vi "Controle_Manip_Main_GUI.vi"() -> ()   [LabVIEW 2019]
doc: "VI for micro-photoluminescence setup in GH013 to study the emission properties of single nanoemitters in the visible range."
uses:
  subVIs/TypeDefs/AcqMode.ctl
  D:/Users/manip-thz/Documents/Controle_Manip_2020/Thorlabs.MotionControl.Controls.dll
  Thorlabs.MotionControl.Controls.dll
  D:/Users/manip-thz/Documents/Controle_Manip_2020/Thorlabs.MotionControl.KCube.SolenoidCLI.dll
  Thorlabs.MotionControl.KCube.SolenoidCLI.dll
  D:/Users/manip-thz/Documents/Controle_Manip_2020/Thorlabs.MotionControl.KCube.PiezoCLI.dll
  Thorlabs.MotionControl.KCube.PiezoCLI.dll
  subVIs/Light Field/lightfield-automation-labview/LightField Automation.lvclass
  subVIs/Light Field/lightfield-automation-labview/VIs/TypeDefs/OpticalPortLocation.ctl
  C:/Program Files/Thorlabs/Scientific Imaging/DCx Camera Support/Develop/DotNet/uc480DotNet.dll
  <vilib>/DAQmx/write.llb/DAQmx Write (Analog DBL 1Chan 1Samp).vi
  <vilib>/DAQmx/create/channels.llb/DAQmx Create Channel (AO-Voltage-Basic).vi
  <vilib>/DAQmx/miscellaneous.llb/DAQmx Fill In Error Info.vi
  subVIs/Globals/Stops.vi
  subVIs/Newport/Newport ESP301/Newport ESP301.lvlib
panel:
  out "Shutter Ctrls":u16(ring)
  out "Laser on?":bool
  in  "Cryostat":enum16{"Montana", "Oxford"}(ring) caption="Cryo :"
  out "Excitation Power (uW)":dbl=0.2 caption="P    =" format="%#_3p"
  in  "Acq Time (ms)":dbl=100.0 caption="Acq Time :" min=0.0 max=360000.0 step=50.0
  in  "Auto< ?":bool
  in  "Acq Mode":T1=enum."Spectrum" caption="Mode :"
  in  "Comment":string
  out "Log file":string caption="Status"
  in  "Experiment Name":string="B1802CF_QD0"
  in  "Experiment Graph Controls":T2(tab)
  in  "CCD 1D Spectrum Main  Cursor2WL 2 Mono 2":bool caption="CCD 1D Spectrum Main  Cursor2WL"
  in  "CCD 1D Spectrum Main  Cursor2WL 1 Mono 2":bool caption="CCD 1D Spectrum Main  Cursor2WL"
  in  "CCD 1D Spectrum Main  Cursor2WL 2 Mono 1":bool caption="CCD 1D Spectrum Main  Cursor2WL"
  in  "CCD 1D Spectrum Main  Cursor2WL 1 Mono 1":bool caption="CCD 1D Spectrum Main  Cursor2WL"
  out "CCD 1D Spectrum Main Cursor 1 nm":dbl caption="nm"
  out "CCD 1D Spectrum Main Cursor 2 nm":dbl caption="nm"
  in  "Full scale":bool
  in  "Acquire Continuous Spectrum":bool
  in  "Acquire Spectrum":bool
  out "CCD 2D Image Main":dbl[][](graph)
  in  "Save Spectrum N":bool
  in  "Save Spectrum":bool
  out "CCD 1D Spectrum Main":cluster{dbl[], dbl[]}(graph)
  in  "Stop continuous":bool
  out "CCD 1D Spectrum Main Energy Scale":cluster{dbl[], dbl[]}(graph)
  out "CCD 1D Spectrum Main Cursor":dbl caption="eV" format="%#_6p"
  out "CCD 1D Spectrum Main Cursor 2":dbl caption="eV" format="%#_6p"
  out "CCD 1D Spectrum Main deltaE":dbl caption="eV" format="%#_3p"
  out "CCD 1D Spectrum Main deltanm":dbl caption="m" format="%#_3p"
  out "XY Intensity Map":dbl[][](graph)=[[3.904687043201515e-13, 6.684989195773002e-11, 3.649880430807626e-09, 6.355065252727497e-08, 3.5287820878809013e-07, 6.248749509463085e-07, 3.5287820878809013e-07, 6.355065252727497e-08, 3.649880430807626e-09, 6.684989195773002e-11, 3.904687043201515e-13], [6.684989195773002e-11, 1.1444983952148092e-08, 6.248749509463097e-07, 1.0880140221963334e-05, 6.041424029819161e-05, 0.0001069812317752422, 6.041424029819161e-05, 1.0880140221963334e-05, 6.248749509463097e-07, 1.1444983952148092e-08, 6.684989195773002e-11], [3.649880430807626e-09, 6.248749509463097e-07, 3.41170163237202e-05, 0.0005940355282204004, 0.003298505755939091, 0.005840977343195246, 0.003298505755939091, 0.0005940355282204004, 3.41170163237202e-05, 6.248749509463097e-07, 3.649880430807626e-09], [6.355065252727497e-08, 1.0880140221963334e-05, 0.0005940355282204004, 0.01034317319661825, 0.05743261926761737, 0.10170139230422684, 0.05743261926761737, 0.01034317319661825, 0.0005940355282204004, 1.0880140221963334e-05, 6.355065252727497e-08], [3.5287820878809013e-07, 6.041424029819161e-05, 0.003298505755939091, 0.05743261926761737, 0.31890655732397044, 0.5647181220077593, 0.31890655732397044, 0.05743261926761737, 0.003298505755939091, 6.041424029819161e-05, 3.5287820878809013e-07], [6.248749509463085e-07, 0.0001069812317752422, 0.005840977343195246, 0.10170139230422684, 0.5647181220077593, 1.0, 0.5647181220077593, 0.10170139230422684, 0.005840977343195246, 0.0001069812317752422, 6.248749509463085e-07], [3.5287820878809013e-07, 6.041424029819161e-05, 0.003298505755939091, 0.05743261926761737, 0.31890655732397044, 0.5647181220077593, 0.31890655732397044, 0.05743261926761737, 0.003298505755939091, 6.041424029819161e-05, 3.5287820878809013e-07], [6.355065252727497e-08, 1.0880140221963334e-05, 0.0005940355282204004, 0.01034317319661825, 0.05743261926761737, 0.10170139230422684, 0.05743261926761737, 0.01034317319661825, 0.0005940355282204004, 1.0880140221963334e-05, 6.355065252727497e-08], [3.649880430807626e-09, 6.248749509463097e-07, 3.41170163237202e-05, 0.0005940355282204004, 0.003298505755939091, 0.005840977343195246, 0.003298505755939091, 0.0005940355282204004, 3.41170163237202e-05, 6.248749509463097e-07, 3.649880430807626e-09], [6.684989195773002e-11, 1.1444983952148092e-08, 6.248749509463097e-07, 1.0880140221963334e-05, 6.041424029819161e-05, 0.0001069812317752422, 6.041424029819161e-05, 1.0880140221963334e-05, 6.248749509463097e-07, 1.1444983952148092e-08, 6.684989195773002e-11], [3.904687043201515e-13, 6.684989195773002e-11, 3.649880430807626e-09, 6.355065252727497e-08, 3.5287820878809013e-07, 6.248749509463085e-07, 3.5287820878809013e-07, 6.355065252727497e-08, 3.649880430807626e-09, 6.684989195773002e-11, 3.904687043201515e-13]]
  out "CCD 2D Image XY Map":dbl[][](graph)
  out "CCD 1D Spectrum XY Map":dbl[][](graph)
  out "Polarisation 2D Image":dbl[][](graph)
  out "Polarisation 1D Spectrum":cluster{dbl[], dbl[]}(graph) caption="64.0°"
  out "Polarisation 1D Spectrum Energy Scale":cluster{dbl[], dbl[]}(graph)
  out "Contrast":dbl
  out "Contrast Oscillations":cluster{dbl[], dbl[]}(graph)
  out "Contrast 1D Spectrum":cluster{dbl[], dbl[]}(graph) caption="143871"
  in  "Cursor controls":bool
  out "Contrast 1D Spectrum from Cursors":cluster{dbl[], dbl[]}(graph) caption="2708"
  in  "Conv/Energy (eV)":dbl caption="Energy :" format="%#_6p"
  in  "Conv/Wavelength (nm)":dbl caption="Wavelength :"
  in  "Conv/Wavenumber (m-1)":dbl caption="Wavenumber :"
  in  "Conv/Time (s)":dbl caption="Time :" format="%#_6p"
  in  "PZC200 COM Port":dbl=10.0 caption="COM Port"
  in  "PZC200 On?":bool
  in  "Laser Diode Current Set":dbl(slide)=0.02 caption="Laser Power (a.u.)" min=0.02 max=0.061 scale=0.02..0.05 scale format="%#_3g"
  in  "Laser on? Control":bool
  in  "Diode Driver COM":refnum<visa-resource-name>="USB0::0x1313::0x804F::M00549740::INSTR"
  in  "Laser Comm On?":bool
  in  "KCube Shutter On?":bool
  in  "KCubes Piezo On?":bool
  in  "LightField On?":bool
  in  "PM16-120 On?":bool
  in  "ESP 300 On?":bool
  in  "ESP 301 On?":bool
  in  "FSM 300 On?":bool
  in  "ESP 300 COM Port":refnum<visa-resource-name>="COM1" caption="COM Port"
  in  "Excitation Wavelength (nm)":dbl=450.0 caption="Exc WL (nm)" min=400.0 max=1100.0 step=1.0
  out "Photodiode Status":bool caption="Status"
  in  "Photodiode COM Port":refnum<visa-resource-name>="USB0::0x1313::0x807B::190927109::INSTR" caption="COM Port"
  in  "ESP 301 COM Port":refnum<visa-resource-name>="COM4" caption="COM Port"
  in  "FSM Y Axis":tag="cDAQ2Mod1/ao1"
  in  "FSM X Axis":tag="cDAQ2Mod1/ao2"
  in  "Slit Width (mm)":dbl
  out "Initialise all devices?":bool caption="OK"
  in  "TEC Output":bool
  out "TEC Temperature":dbl caption="TEC Temp" format="%#_4f"
  out "Laser Safety":u16(ring)
  in  "LF Visible":bool=TRUE
  out "PZC200 Instrument Channel":string="RS232/10"
  out "Left Limit (mm)":dbl format="%#.3g"
  out "Right Limit (mm)":dbl format="%#.3g"
  out "PZC Error":errorcluster
  in  "Diode Driver Error":errorcluster caption="error in (no error)" {"code" format="%.0x"}
  in  "ESP 301 Error":errorcluster
  out "KCubeSolenoidControl Reference":refnum<k24>
  out "KCube Shutter Device Reference":refnum<k24>
  out "KCubePiezoDevice Z Reference":refnum<k24>
  out "KCubePiezoControl Z Reference":refnum<k24>
  out "KCubePiezoControl Y Reference":refnum<k24>
  out "KCubePiezoDevice Y Reference":refnum<k24>
  out "KCubePiezoDevice X Reference":refnum<k24>
  out "KCubePiezoControl X Reference":refnum<k24>
  out "Wavelength calibration":dbl[](array[numeric])
  out "Photodiode handle out":refnum<visa-resource-name> caption="instrument handle out"
  out "Photodiode error out":errorcluster caption="error out" {"code" format="%.0x"}
  out "LightField Automation error out":errorcluster
  out "Scan Polar Params":refnum<vi>[](array[refnum])
  out "Angles":dbl[](array[numeric])
  out "Scan XY Map Params":refnum<vi>[](array[refnum])
  out "Thorcam Error":errorcluster caption="Error Out"
  out "Data":T3(array[cluster])
  in  "ESP300 Error":errorcluster
  out "Serial Number":string
  out "ThorCam Reference":refnum<k24>
  out "LightField Automation out":refnum<class "LightField Automation.lvclass">
  out "Response":string
  out "Scan LinTFine Params":refnum<vi>[](array[refnum])
  out "Contrast Oscill data":dbl[](array[numeric])
  out "PZA12 Positions":dbl[](array[numeric])
  out "Contrast Array Out":dbl[][](array[numeric])
  out "Michelson Array Out":dbl[][][](array[numeric])
  in  "Stop Everything & Quit?":bool
  in  "Excitation Source":enum16{"P", "CW"}(ring)=enum."CW" caption="Laser"
  in  "Temperature (K)":dbl=5.0 caption="T ="
  in  "Experimental parameters tab":T4(tab)
  in  "Center Wavelength (nm) Mono 2":dbl
  in  "Mono2 Motor Position":dbl
  out "Mono2 On":bool
  in  "CCD ROI":T5(ring)
  in  "Spectrum Step Wavelength (nm)":dbl=490.12 caption="Step WL (nm)"
  in  "Spectrum End Wavelength (nm)":dbl=490.12 caption="End WL (nm)"
  in  "Spectrum Start Wavelength (nm)":dbl=490.12 caption="Start WL (nm)"
  in  "Accumulations":dbl=1.0 caption="Accum."
  in  "Background substract":enum16{"None", "Shutter"}(ring) caption="Bkg substract"
  in  "Exit mirror":enum16{"CCD", "APD"}(ring) caption="Exit :"
  in  "Center Wavelength (nm)":dbl=490.12 caption="Center WL :"
  in  "Exposure Time (ms)":dbl=500.0 caption="Exp Time :" min=0.0 max=360000.0 step=50.0
  in  "Grating":string(combo)="[h-vis,2400][0][0]"
  out "CCD T° :":dbl
  out "Exit Port Location":T6 items=["None"=1, "SideEntrance"=2, "FrontEntrance"=3, "SideExit"=5, "FrontExit"=4]
  out "Scan Spectrum Progess Bar":u8(slide) scale=0.0..100.0
  in  "Stop XY Map":bool
  out "Scan X Readout (V)":dbl caption="X Readout (V)" min=-10.0 max=10.0
  out "Scan Y Readout (V)":dbl caption="Y Readout (V)" min=-10.0 max=10.0
  out "Scan XY Map Progess Bar":u8(slide) scale=0.0..100.0
  in  "Scan Y Tot. Length":dbl caption="Y Length"
  in  "Scan X Tot. Length (V)":dbl caption="X Length (V)"
  in  "Scan Y Num. Pts":dbl caption="Y # Pts"
  in  "Scan X Num. Pts":dbl caption="X # Pts"
  in  "Scan Y Res. (V)":dbl caption="Res. Y (V)"
  in  "Scan X Res. (V)":dbl caption="Res. X (V)"
  in  "Scan Y Center (V)":dbl caption="Y Center (V)"
  in  "Scan X Center (V)":dbl caption="X Center (V)"
  in  "FSM Home":bool
  in  "FSM Right":bool
  in  "FSM Left":bool
  in  "FSM Down":bool
  in  "FSM Up":bool
  in  "FSM X Axis Pos":dbl min=-10.0 max=10.0
  in  "FSM Y Axis Pos":dbl min=-10.0 max=10.0
  in  "FSM Axis Step":dbl=0.1
  in  "Save XY Map":bool
  in  "Acquire XY Map":bool
  in  "Scanning Mode":T7(ring) caption="Mode"
  in  "Scan Fast Axis":enum16{"Y", "X"}(ring)=enum."X" caption="Fast Axis"
  in  "PausePolar":bool
  out "RotStage Det Angle Readout (°)":dbl=2.0 caption="Readout (°)" min=-360.0 max=360.0 format="%#_4g"
  out "RotStage Exc Angle Readout (°)":dbl=2.0 caption="Readout (°)" min=-360.0 max=360.0 format="%#_4g"
  in  "Acquire Polarisation":bool
  in  "RotStage Det Angle Step (°)":dbl=10.0 caption="Step (°)"
  in  "RotStage Exc Angle Step (°)":dbl=10.0 caption="Step (°)"
  in  "RotStage Det Jog Forward":bool
  in  "RotStage Exc Jog Forward":bool
  in  "RotStage Det Jog Backward":bool
  in  "RotStage Det Home":bool caption="Home"
  in  "RotStage Exc Home":bool caption="Home"
  in  "RotStage Det Angle (°)":dbl=2.0 caption="Target (°)" min=-360.0 max=360.0 format="%#_4g"
  in  "RotStage Exc Angle (°)":dbl=2.0 caption="Target (°)" min=-360.0 max=360.0 format="%#_4g"
  in  "RotStage Exc Jog Backward":bool
  in  "Polar Start Angle (°)":dbl caption="Start angle (°)" min=0.0 max=360.0 step=10.0
  in  "Polar End Angle (°)":dbl=360.0 caption="End Angle (°)" min=0.0 max=360.0 step=10.0
  in  "Polar Step Angle (°)":dbl=10.0 caption="Step Angle (°)" min=1.0 max=360.0
  in  "Polar mode":u16(ring)=3 caption="Rotate polarisation" items=["Excitation"=3, "Detection"=2]
  in  "Save Polarisation":bool
  out "Scan Polarisation Progess Bar":u8(slide) scale=0.0..100.0
  in  "RotStage Det Velocity (°/s)":dbl=2.0 caption="Velocity (°/s)" min=1.0 max=20.0 step=1.0
  in  "RotStage Exc Velocity (°/s)":dbl=2.0 caption="Velocity (°/s)" min=1.0 max=20.0 step=1.0
  in  "StopPolar":bool
  in  "Motor RotStage Exc On?":bool
  in  "Motor RotStage Det On?":bool
  in  "Stop Contrast":bool
  in  "Pause Contrast":bool
  in  "Save Contrast":bool
  in  "Newport PZA12 Stage Position (usteps)":dbl caption="Target (usteps)" min=-8.0 max=392.0
  in  "Reset origins":bool
  in  "LinTFine Motor On?":bool caption="Motor on?"
  in  "Acquire Contrast":bool
  in  "LinTFines Step Pos (usteps)":dbl=1.0 caption="Step pos (usteps)" min=1.0 max=100.0 step=1.0
  in  "LinTFine End Pos (usteps)":dbl=10.0 caption="End pos (usteps)" min=-1000000.0 max=1000000.0 step=1.0
  in  "LinTFine Start Pos (usteps)":dbl caption="Start pos (usteps)" min=-1000000.0 max=1000000.0 step=1.0
  in  "PZC Speed (usteps/s)":u16(ring) caption="Velocity (usteps/s)" items=["0", "3.2", "16", "80", "400", "2000", "10000", "48000"]
  in  "PZC Jog Forward":bool
  in  "PZC Jog Backward":bool
  in  "PZC Home":bool caption="Home"
  out "PZC Position Readout (usteps)":dbl caption="Readout (usteps)" min=-8.0 max=392.0
  out "Newport Linear Translation Stage Position Readout (mm)":dbl caption="Readout (mm)" min=-8.0 max=392.0 format="%#_7g"
  in  "Newport Linear Translation Stage Step (mm)":dbl=5.0 caption="Step (mm)"
  in  "Delay Line Position (mm)":dbl caption="Delay line position (mm)"
  in  "Newport Linear Translation Stage Position (mm)":dbl caption="Target (mm)" min=-8.0 max=392.0
  out "Scan Linear Stage Progess Bar":u8(slide) scale=0.0..100.0
  in  "Newport Linear Translation Stage Home":bool caption="Home"
  in  "Newport Linear Translation Stage Jog Forward":bool
  in  "Newport Linear Translation Stage Jog Backward":bool
  in  "Newport Linear Translation Stage Velocity (mm/s)":dbl=1.0 caption="Velocity (mm/s)" min=1.0 max=100.0 step=1.0
  in  "LinT Step Pos (mm)":dbl=10.0 caption="Step pos (mm)" min=1.0 max=250.0 step=0.001
  in  "LinT End pos (mm)":dbl=250.0 caption="End pos (mm)" min=0.0 max=250.0 step=10.0
  in  "LinT Start Pos (mm)":dbl caption="Start pos (mm)" min=0.0 max=360.0 step=10.0
  in  "Motor LinT On?":bool
  in  "KCubePiezoControl Z":refnum<k24>(container) caption="Focus"
  in  "KCubePiezoControl X":refnum<k24>(container) caption="Lateral"
  in  "KCubePiezoControl Y":refnum<k24>(container) caption="Vertical"
  in  "KCubeSolenoidControl":refnum<k24>(container)
  in  "Shutter Mode":i32(ring)=1 items=["Manual"=1, "SingleToggle"=2, "AutoToggle"=3, "Triggered"=4]
  in  "Shutter mode":bool
  # "K"
  # "exc"
  # "W"
  # "ms"
  # "Mono 1"
  # "Mono 2"
  # "--|--"
  # "CenterWL"
  # "l   ="
  # "E  ="
  # "DE ="
  # "1"
  # "1"
  # "--|--"
  # "Dl ="
  # "CenterWL"
  # "l   ="
  # "E   ="
  # "2"
  # "2"
  # "Absolute conversions"
  # "change one value manually and the others will update automatically"
  # "Relative conversions"
  # "eV"
  # "nm"
  # "-1"
  # "cm"
  # "s"
  # "Thorlabs Laser Diode Driver CLD1010"
  # "Newport FSM-300-01"
  # "Newport ESP 301"
  # "Newport PZC200"
  # "Newport ESP 300"
  # "Thorlabs PM16-120"
  # "Thorlabs Shutter SH05"
  # "Thorlabs NanoMax + 3 Axis Piezos"
  # "Princeton HRS-500 + Pixis"
  # "min"
  # "max"
  # "Controls"
  # "Scans"
  # "add functionnality spectrum with APD 1 or APD 2\nwith option AcqMode (with frw&bckw talk to Exit mirror)"
  # "Possibly add a slit size option to determine the resolution"
  # "nm"
  # "ms"
  # "°C"
  # "Controls"
  # "Scans"
  # "Controls"
  # "Scans"
  # "Excitation"
  # "Detection"
  # "Controls"
  # "Scans"
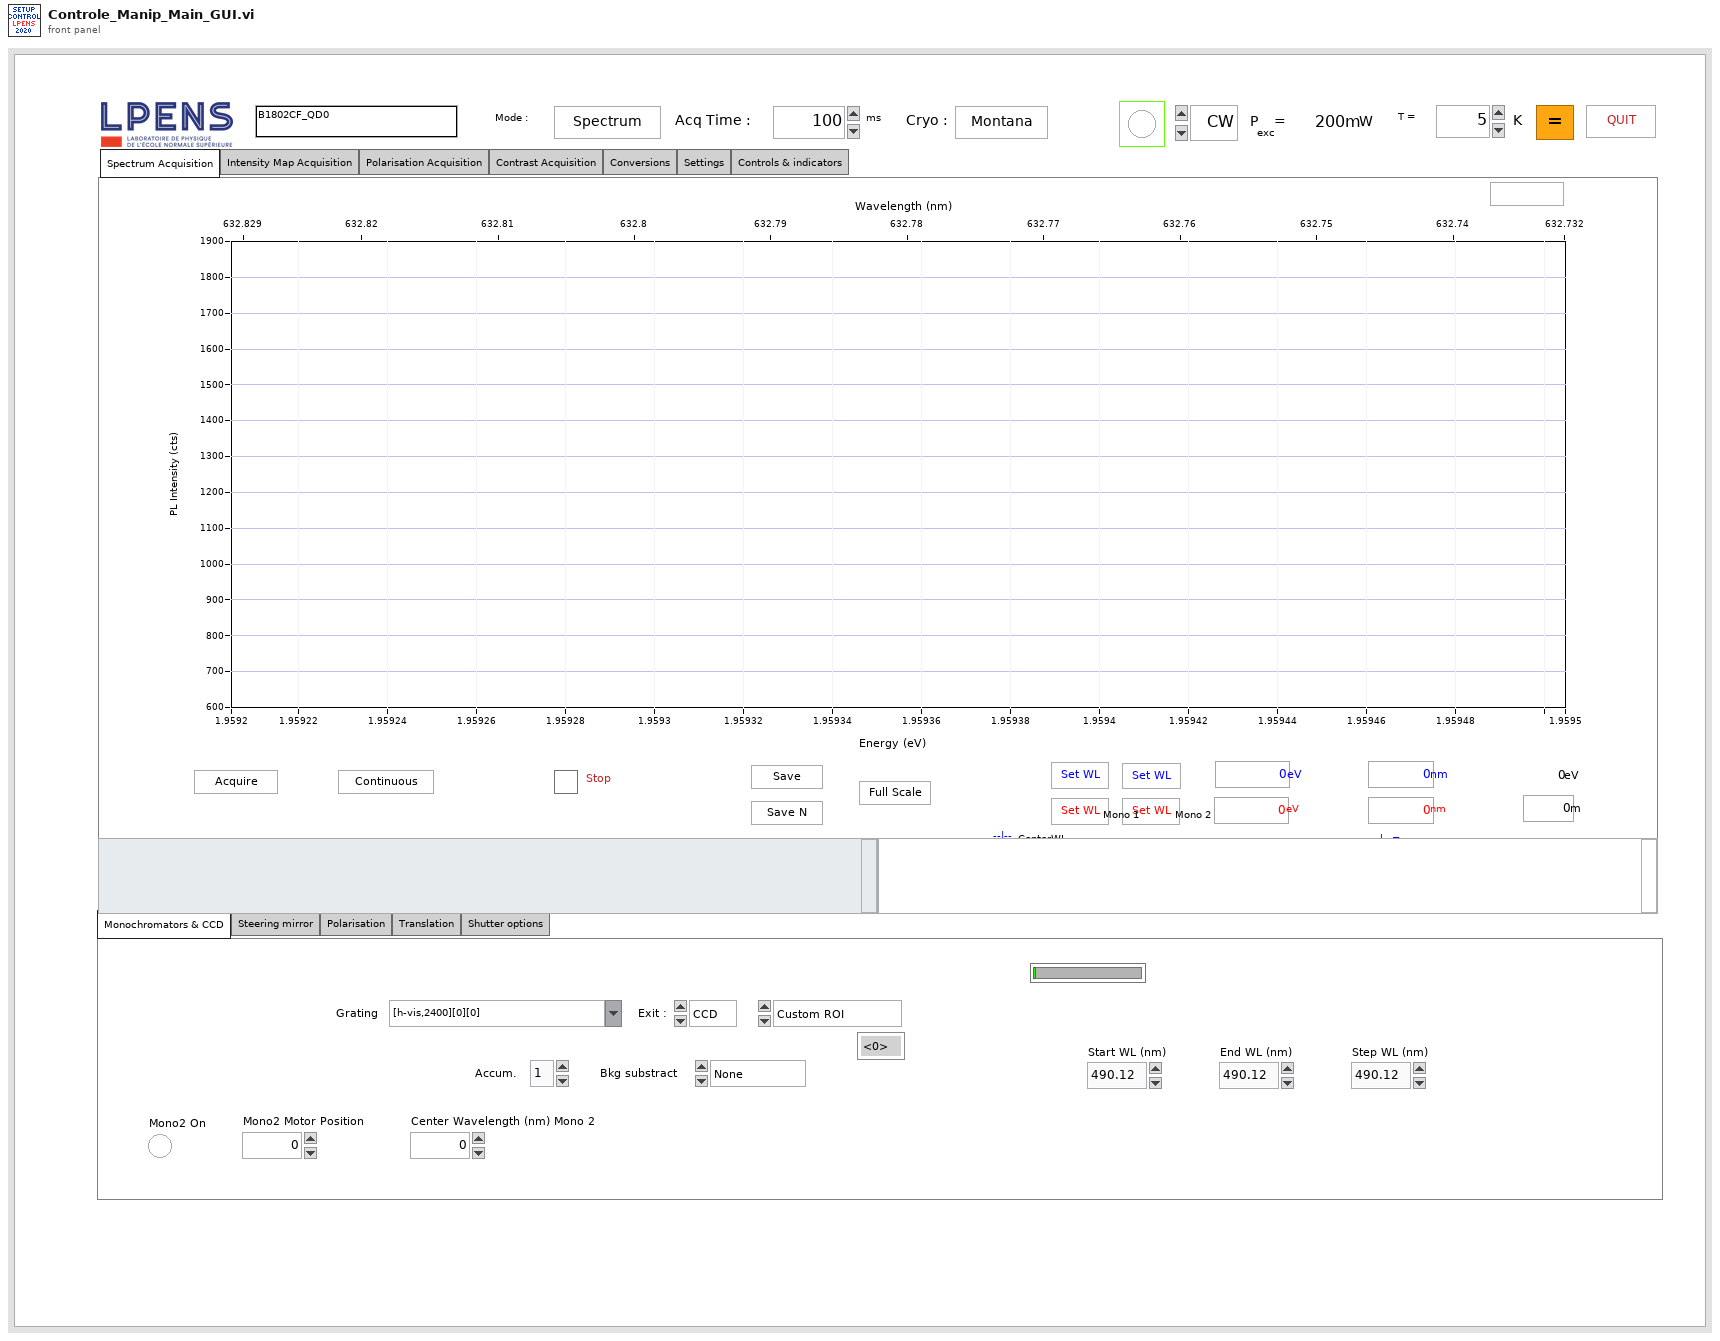
[diagram p1: front panel]
types:
  T1 = typedef "AcqMode.ctl" = enum16{"Image", "Spectrum", "APD 1", "APD 2", "APD 1+2"}
  T2 = enum32{"Spectrum Acquisition", "Intensity Map Acquisition", "Polarisation Acquisition", "Contrast Acquisition", "APDs Acquisition", "Conversions", "Settings", "Controls & indicators"}
  T3 = cluster{"Image":dbl[][][], "Frame Size":cluster{"F":i32, "Y":i32, "X":i32}}[]
  T4 = enum32{"Monochromators & CCD", "Steering mirror", "Polarisation", "Translation", "Microscope objective", "Shutter options"}
  T5 = enum16{"Custom ROI", "Full sensor", "Binned full sensor"}
  T6 = typedef "LightField Automation.lvclass/OpticalPortLocation.ctl" = i32
  T7 = enum16{"Default", "Snail", "Random", "Snake", "Line"}
  T8 = enum32{"Page Enabled", "Page Disabled", "Page Disabled & Grayed"}
  T9 = enum16{"Contrast", "Spectre", "Polarisation", "XY Intensity Map"}
  T10 = enum16{"Image", "Spectrum", "APD 1", "APD 2", "APD 1+2"}
  T11 = enum32{"Spectrum Acquisition", "XY Intensity Map Acquisition", "Polarisation Acquisition", "APDs Acquisition", "Conversions", "Settings"}
  T12 = enum16{"Contrast", "XY Intensity Map", "Polarisation", "Spectrum"}
  T13 = typedef "LVRangeTypeDef.ctl" = cluster{"Minimum":dbl, "Maximum":dbl, "Increment":dbl, "Minor Increment":dbl, "Start":dbl}
  T14 = cluster{"PZA12 Positions":dbl[], "Contrast of ROI vs PZC":dbl[]}
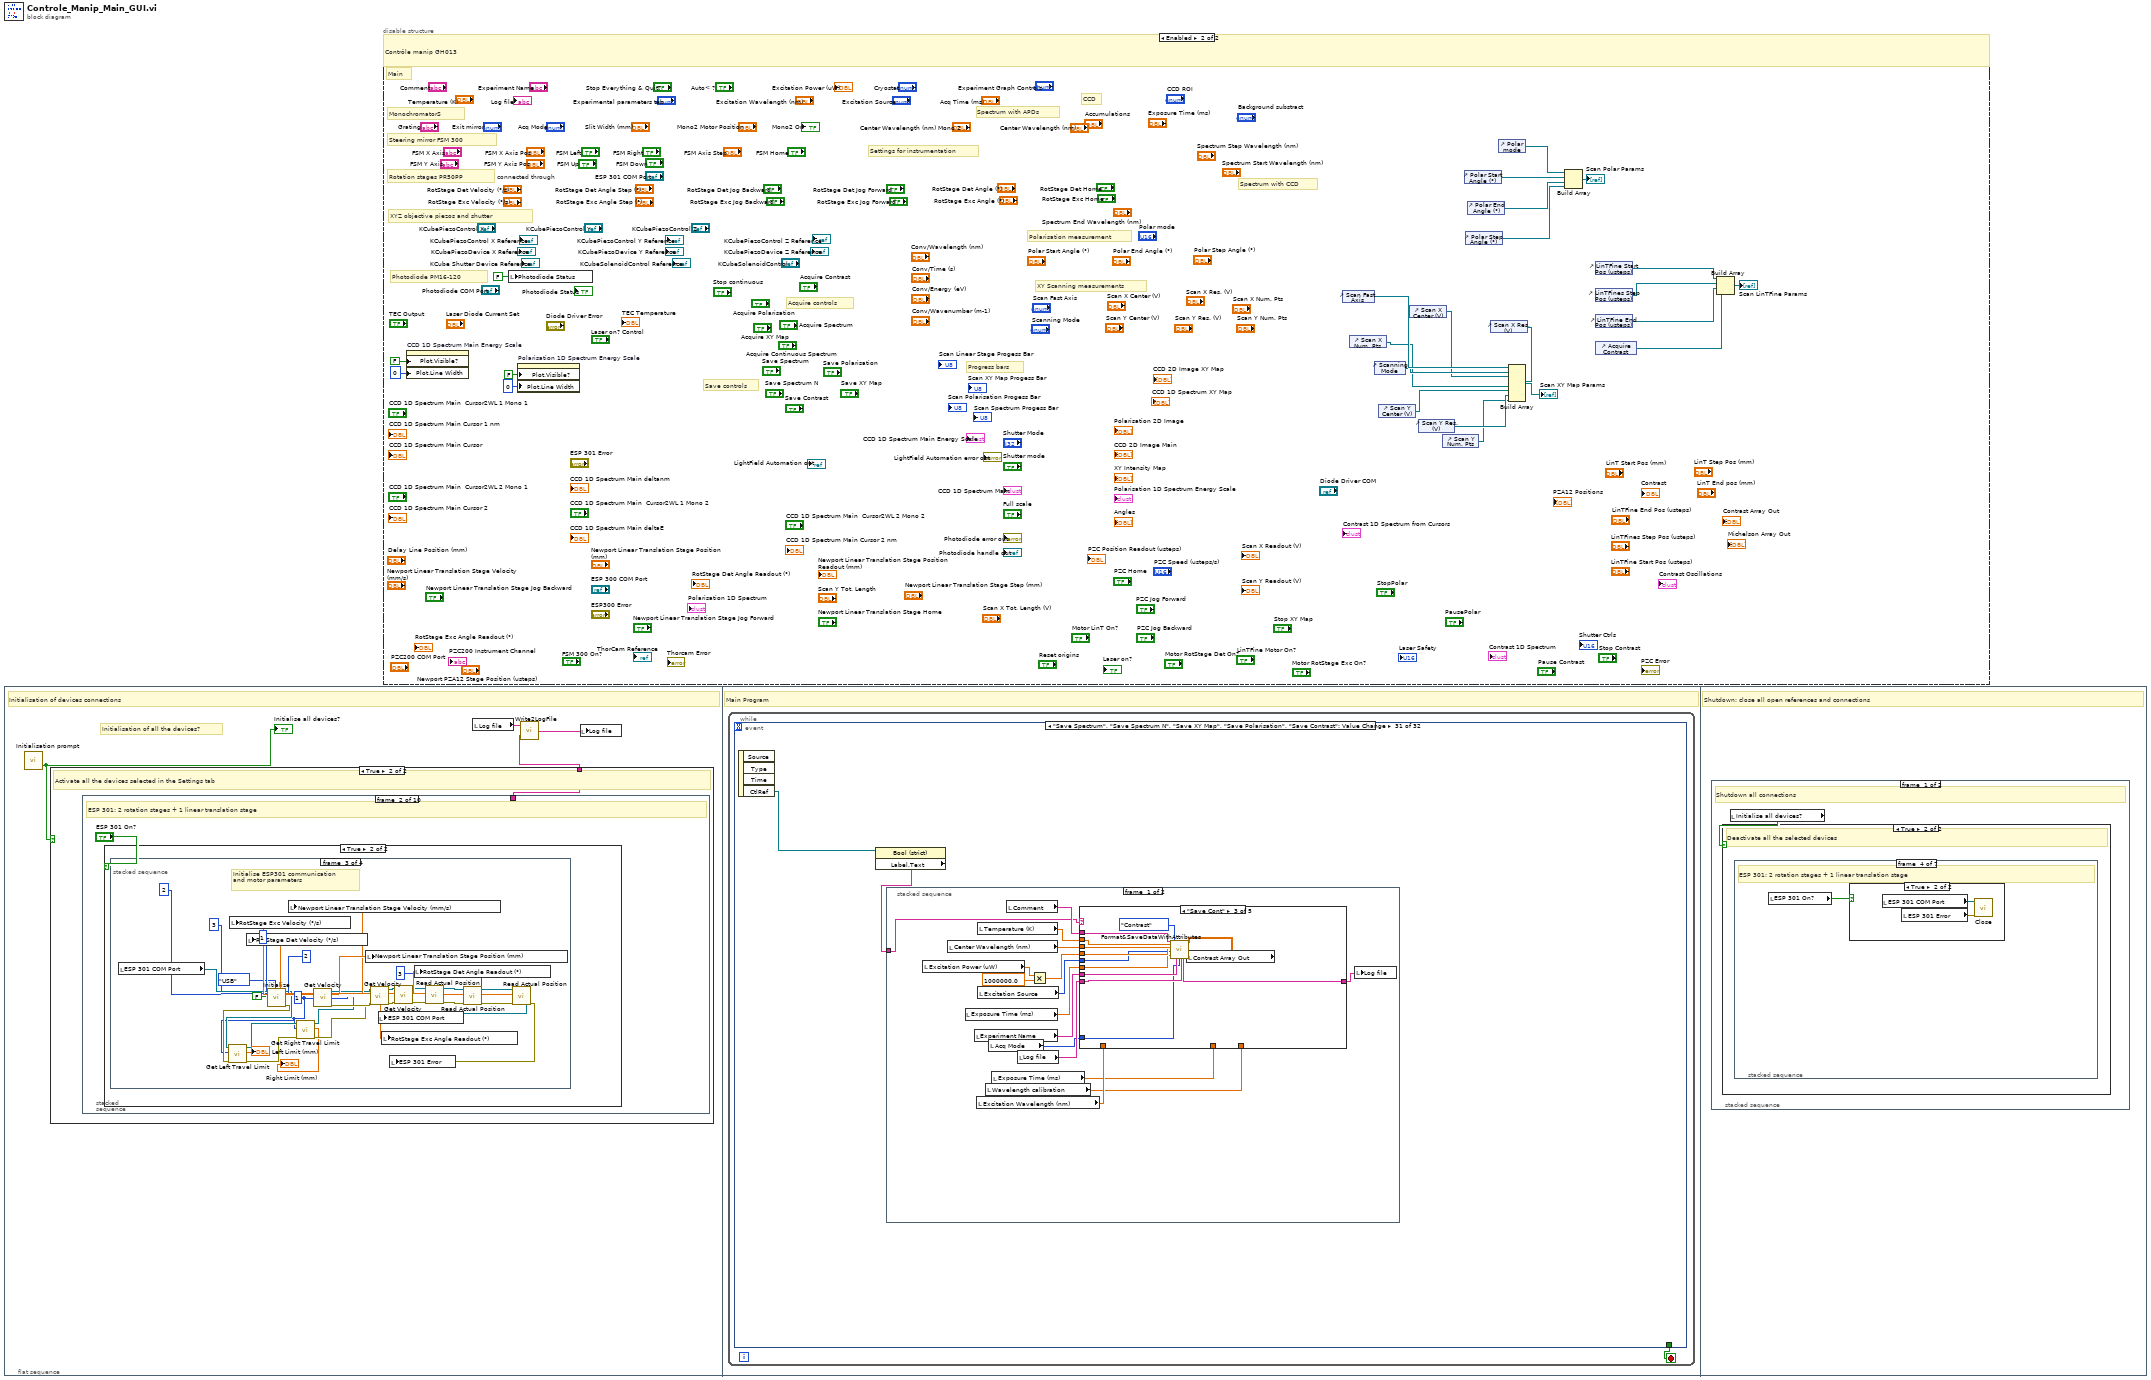
[diagram p0: block diagram]
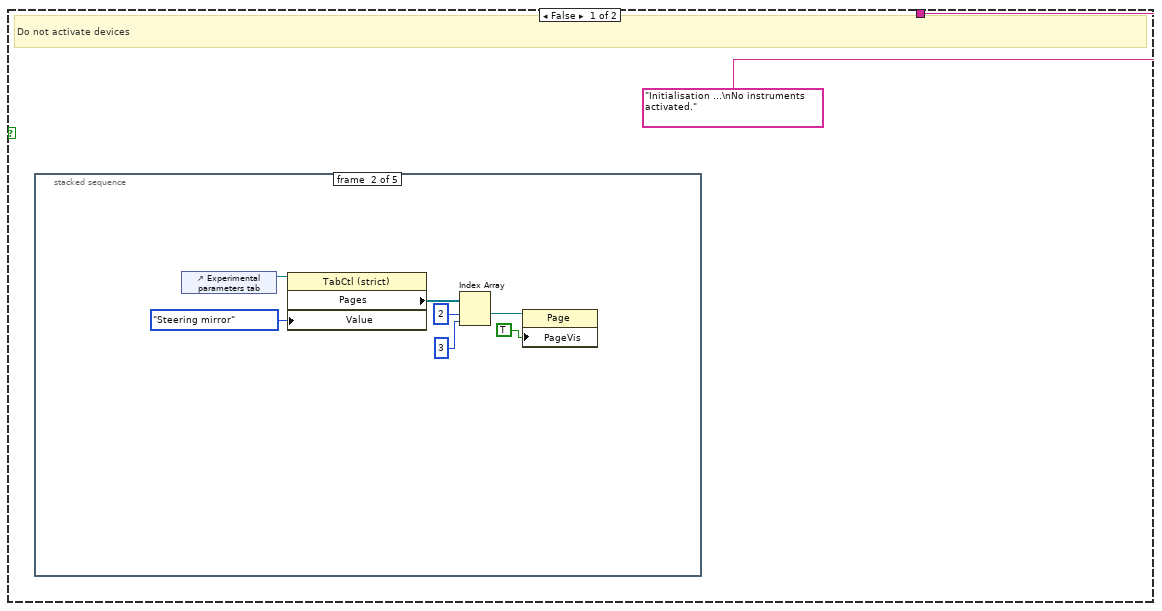
[diagram p3: hidden frame]
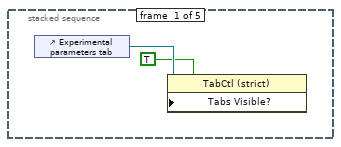
[diagram p4: hidden frame]
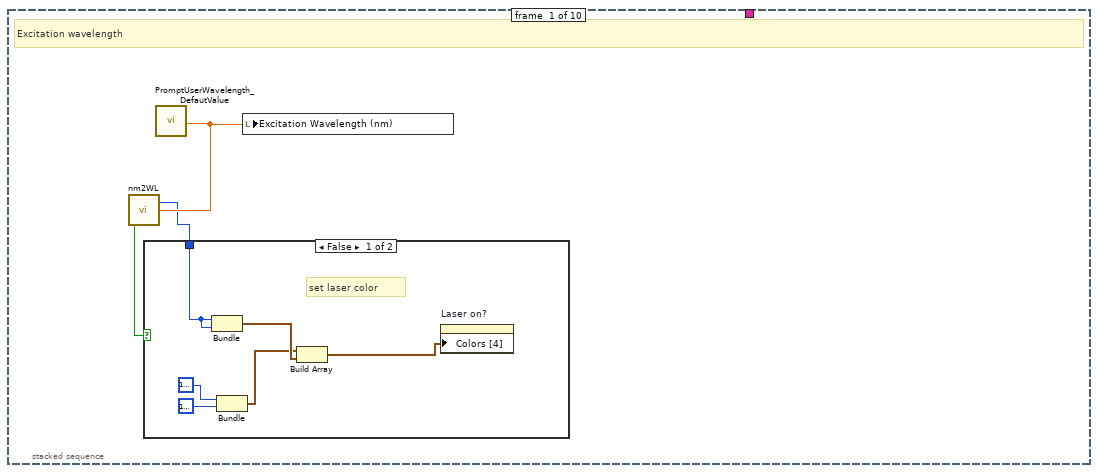
[diagram p8: hidden frame]
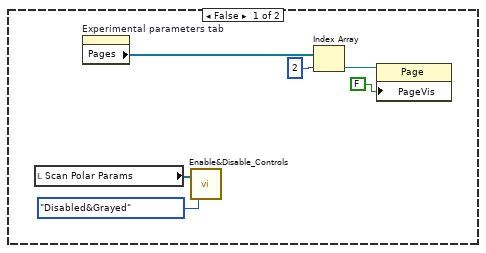
[diagram p10: hidden frame]
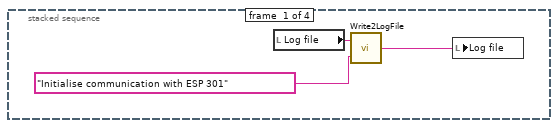
[diagram p11: hidden frame]
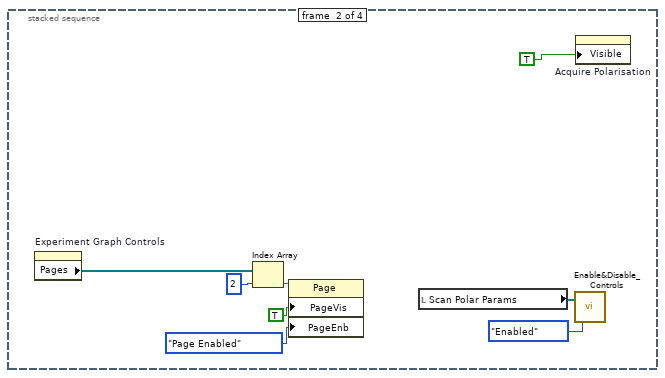
[diagram p12: hidden frame]
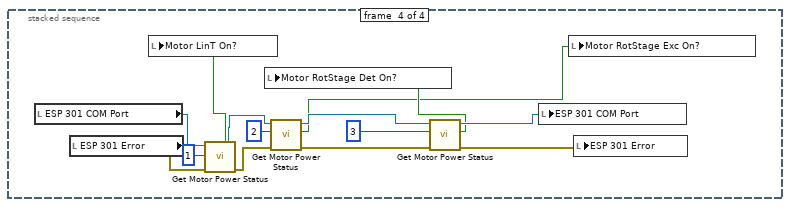
[diagram p13: hidden frame]
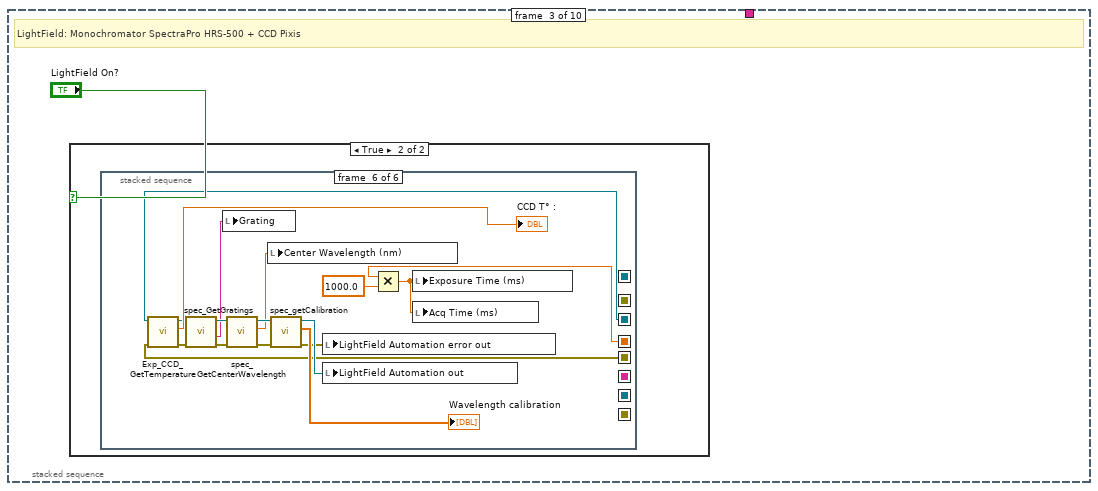
[diagram p14: hidden frame]
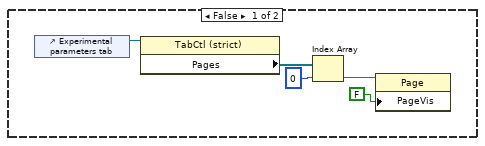
[diagram p15: hidden frame]
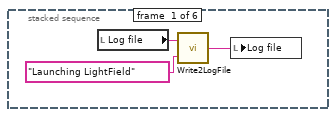
[diagram p16: hidden frame]
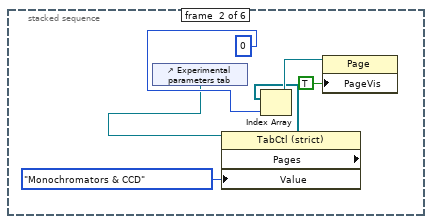
[diagram p17: hidden frame]
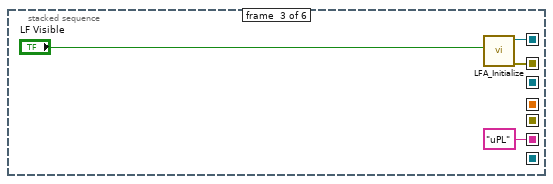
[diagram p18: hidden frame]
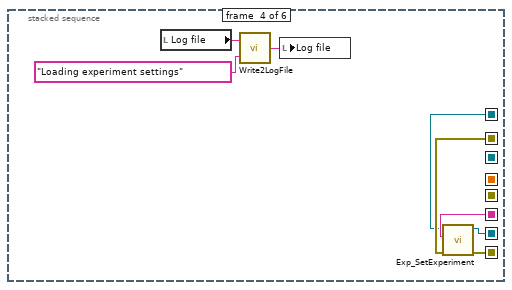
[diagram p19: hidden frame]
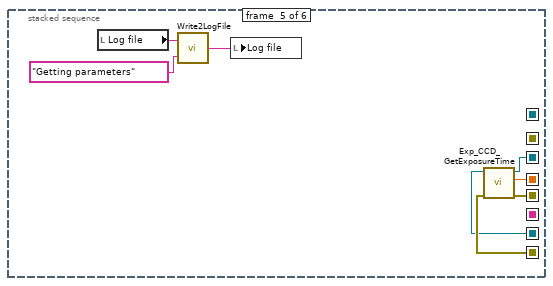
[diagram p20: hidden frame]
diagram:
  n1 = flat-sequence {
    frame #0 {
      # "Initialisation of all the devices?"
      # "Initialisation of devices connections"
      n2 = call "Initialisation prompt"() -> ("Yes please!"=w1:bool)  [unwired: 18 in, 1 out]
      "Initialise all devices?" <- w1
      n3 = case shown="True" w1 {
        tunnel: ["Initialisation ...\nNo instruments activated." w15] -> w3
        frame False {
          # "Do not activate devices"
          n4 = stacked-sequence {
            frame #0 {
              n5 = control-ref of="Experimental parameters tab"() -> (w7:refnum<vi>)
              n6 = property class="TabCtl (strict)"(reference=w7, "Tabs Visible?"=TRUE) -> ()  [unwired: 1 in, 2 out]
            }
            frame #1 {
              n7 = control-ref of="Experimental parameters tab"() -> (w12:refnum<vi>)
              n8 = property class="TabCtl (strict)"(reference=w12, "Value"=T4."Steering mirror") -> ("Pages"=w13:refnum<vi>[])  [unwired: 1 in, 2 out]
              n9 = Index Array(array=w13, index #1=2 ("index"), index #2=3 ("index")) -> (element #1=w14:refnum<vi>)  [unwired: 1 out]
              n10 = property class="Page"(reference=w14, "PageVis"=TRUE ("Page Visible")) -> ()  [unwired: 1 in, 2 out]
            }
            frame #2 {
            }
            frame #3 {
            }
            frame #4 {
            }
          }
        }
        frame True {
          # "Activate all the devices selected in the Settings tab"
          n11 = stacked-sequence {
            tunnel: [_ _ _ _ _ _ _ _ _ "All devices activated !"] -> w15
            frame #0 {
              # "Excitation wavelength"
              n12 = call "PromptUserWavelength_DefautValue.vi"() -> ("Wavelength"=w18:dbl)  [unwired: 17 in, 2 out]
              n13 = call "nm2WL.vi"("Wavelength (380 - 780)"=w18) -> ("Color"=w16:u32, "Out Of Range"=w17:bool)
              n14 = case shown="False" w17 {
                tunnel: w16 -> [w22 _]
                frame False {
                  # "set laser color"
                  n15 = Bundle("Color"=w22, "Color"=w22) -> (w21:cluster{"Color":u32, "Color":u32})  [unwired: 1 in]
                  n16 = Bundle(u32 16777216, u32 16777216) -> (w20:cluster{u32, u32})  [unwired: 1 in]
                  n17 = Build Array(w20, w21) -> (w19:cluster{"Color":u32, "Color":u32}[])
                  n18 = property on="Laser on?" class="Bool (strict)"("Colors [4]"=w19) -> ()  [unwired: 2 in, 2 out]
                }
                frame True {
                }
              }
              n19 = local write "Excitation Wavelength (nm)"(w18) -> ()
            }
            frame #1 {
              # "ESP 301: 2 rotation stages + 1 linear translation stage"
              n20 = case shown="True" "ESP 301 On?" {
                frame False {
                  n21 = local read "Scan Polar Params"() -> (w27:refnum<vi>[])
                  n22 = property on="Experimental parameters tab" class="TabCtl (strict)"() -> ("Pages"=w31:refnum<vi>[])  [unwired: 2 in, 2 out]
                  n23 = call "Enable&Disable_Controls.vi"("Enum"=enum16{"Enabled", "Disabled", "Disabled&Grayed"}."Disabled&Grayed", "References"=w27) -> ()  [unwired: 1 in]
                  n24 = Index Array(array=w31, index=2) -> (element=w29:refnum<vi>)
                  n25 = property class="Page"(reference=w29, "PageVis"=FALSE ("Page Visible")) -> ()  [unwired: 1 in, 2 out]
                }
                frame True {
                  n26 = stacked-sequence {
                    frame #0 {
                      n27 = local read "Log file"() -> (w34:string)
                      n28 = call "Write2LogFile.vi"("Add to log file"="Initialise communication with ESP 301", "Log file before"=w34) -> ("Log file after"=w32:string)
                      n29 = local write "Log file"(w32) -> ()
                    }
                    frame #1 {
                      n30 = property on="Experiment Graph Controls" class="TabCtl (strict)"() -> ("Pages"=w39:refnum<vi>[])  [unwired: 2 in, 2 out]
                      n31 = Index Array(array=w39, index=2) -> (element=w37:refnum<vi>)
                      n32 = property class="Page"(reference=w37, "PageVis"=TRUE ("Page Visible"), "PageEnb"=T8."Page Enabled" ("Page Enabled State")) -> ()  [unwired: 1 in, 2 out]
                      n33 = local read "Scan Polar Params"() -> (w42:refnum<vi>[])
                      n34 = call "Enable&Disable_Controls.vi"("Enum"=enum16{"Enabled", "Disabled", "Disabled&Grayed"}."Enabled", "References"=w42) -> ()  [unwired: 1 in]
                      n35 = property on="Acquire Polarisation" class="Bool (strict)"("Visible"=TRUE ("Acquire Polarisation")) -> ()  [unwired: 2 in, 2 out]
                    }
                    frame #2 {
                      w44 = 1 ("Axis (1)")
                      # "Initialise ESP301 communication\nand motor parameters"
                      n36 = local read "ESP 301 COM Port"() -> (w59:refnum<visa-resource-name>)
                      n37 = call "Initialize.vi"("VISA resource name"=w59, "ID Query (True)"=FALSE, "Serial Link (RS232)"=enum16{"RS232", "USB"}."USB") -> ("VISA resource name out"=w48:refnum<visa-resource-name>, "error out"=w45:errorcluster)  [unwired: 6 in]
                      n38 = call "Get Left Travel Limit.vi"("error in (no error)"=w45, "Axis (1)"=w44, "VISA resource name"=w48) -> ("error out"=w46:errorcluster, "Left Travel Limit (units)"=→"Left Limit (mm)":dbl, "VISA resource name out"=w47:refnum<visa-resource-name>)  [unwired: 2 in]
                      n39 = call "Get Right Travel Limit.vi"("error in (no error)"=w46, "Axis (1)"=w44, "VISA resource name"=w47) -> ("error out"=w50:errorcluster, "Right Travel Limit (units)"=→"Right Limit (mm)":dbl, "VISA resource name out"=w51:refnum<visa-resource-name>)  [unwired: 2 in]
                      n40 = call "Get Velocity.vi"("error in (no error)"=w50, "Axis (1)"=w44, "VISA resource name"=w51) -> ("error out"=w62:errorcluster, "Velocity (units/s)"=w64:dbl, "VISA resource name out"=w61:refnum<visa-resource-name>)  [unwired: 2 in]
                      n41 = local write "Newport Linear Translation Stage Velocity (mm/s)"(w64) -> ()
                      n42 = call "Get Velocity.vi"("error in (no error)"=w62, "Axis (1)"=2, "VISA resource name"=w61) -> ("error out"=w63:errorcluster, "Velocity (units/s)"=w66:dbl, "VISA resource name out"=w60:refnum<visa-resource-name>)  [unwired: 2 in]
                      n43 = local write "RotStage Exc Velocity (°/s)"(w66) -> ()
                      n44 = call "Get Velocity.vi"("error in (no error)"=w63, "Axis (1)"=3, "VISA resource name"=w60) -> ("error out"=w68:errorcluster, "Velocity (units/s)"=w65:dbl, "VISA resource name out"=w67:refnum<visa-resource-name>)  [unwired: 2 in]
                      n45 = local write "RotStage Det Velocity (°/s)"(w65) -> ()
                      n46 = call "Read Actual Position.vi"("error in (no error)"=w68, "Axis (1)"=1, "VISA resource name"=w67) -> ("error out"=w74:errorcluster, "Position (units)"=w75:dbl, "VISA resource name out"=w73:refnum<visa-resource-name>)  [unwired: 2 in]
                      n47 = local write "Newport Linear Translation Stage Position (mm)"(w75) -> ()
                      n48 = call "Read Actual Position.vi"("error in (no error)"=w74, "Axis (1)"=2, "VISA resource name"=w73) -> ("error out"=w71:errorcluster, "Position (units)"=w69:dbl, "VISA resource name out"=w72:refnum<visa-resource-name>)  [unwired: 2 in]
                      n49 = local write "RotStage Det Angle Readout (°)"(w69) -> ()
                      n50 = call "Read Actual Position.vi"("error in (no error)"=w71, "Axis (1)"=3, "VISA resource name"=w72) -> ("error out"=w77:errorcluster, "Position (units)"=w70:dbl, "VISA resource name out"=w76:refnum<visa-resource-name>)  [unwired: 2 in]
                      n51 = local write "ESP 301 COM Port"(w76) -> ()
                      n52 = local write "RotStage Exc Angle Readout (°)"(w70) -> ()
                      n53 = local write "ESP 301 Error"(w77) -> ()
                    }
                    frame #3 {
                      n54 = local read "ESP 301 COM Port"() -> (w91:refnum<visa-resource-name>)
                      n55 = local read "ESP 301 Error"() -> (w90:errorcluster)
                      n56 = call "Get Motor Power Status.vi"("error in (no error)"=w90, "Axis (1)"=1, "VISA resource name"=w91) -> ("error out"=w84:errorcluster, "Power Status"=w80:bool, "VISA resource name out"=w85:refnum<visa-resource-name>)  [unwired: 2 in]
                      n57 = local write "Motor LinT On?"(w80) -> ()
                      n58 = call "Get Motor Power Status.vi"("error in (no error)"=w84, "Axis (1)"=2, "VISA resource name"=w85) -> ("error out"=w87:errorcluster, "Power Status"=w78:bool, "VISA resource name out"=w86:refnum<visa-resource-name>)  [unwired: 2 in]
                      n59 = call "Get Motor Power Status.vi"("error in (no error)"=w87, "Axis (1)"=3, "VISA resource name"=w86) -> ("error out"=w88:errorcluster, "Power Status"=w79:bool, "VISA resource name out"=w89:refnum<visa-resource-name>)  [unwired: 2 in]
                      n60 = local write "Motor RotStage Det On?"(w79) -> ()
                      n61 = local write "ESP 301 COM Port"(w89) -> ()
                      n62 = local write "Motor RotStage Exc On?"(w78) -> ()
                      n63 = local write "ESP 301 Error"(w88) -> ()
                    }
                  }
                }
              }
            }
            frame #2 {
              # "LightField: Monochromator SpectraPro HRS-500 + CCD Pixis"
              n64 = case shown="True" "LightField On?" {
                frame False {
                  n65 = control-ref of="Experimental parameters tab"() -> (w93:refnum<vi>)
                  n66 = property class="TabCtl (strict)"(reference=w93) -> ("Pages"=w96:refnum<vi>[])  [unwired: 1 in, 2 out]
                  n67 = Index Array(array=w96, index=0) -> (element=w97:refnum<vi>)
                  n68 = property class="Page"(reference=w97, "PageVis"=FALSE ("Page Visible")) -> ()  [unwired: 1 in, 2 out]
                }
                frame True {
                  n69 = stacked-sequence {
                    seq-local: [_ _ "uPL" ("ExperimentName") _ _ _] -> [_ _ _ w117 _ _]
                    seq-local: [_ _ w109 _ _ _] -> [_ _ _ w118 _ _]
                    seq-local: [_ _ w108 _ _ _] -> [_ _ _ w116 _ _]
                    seq-local: [_ _ _ w115 _ _] -> [_ _ _ _ w126 _]
                    seq-local: [_ _ _ w114 _ _] -> [_ _ _ _ w125 _]
                    seq-local: [_ _ _ _ w120 _] -> [_ _ _ _ _ w128]
                    seq-local: [_ _ _ _ w121 _] -> [_ _ _ _ _ w129]
                    seq-local: [_ _ _ _ w119 _] -> [_ _ _ _ _ w127]
                    frame #0 {
                      n70 = local read "Log file"() -> (w99:string)
                      n71 = call "Write2LogFile.vi"("Add to log file"="Launching LightField", "Log file before"=w99) -> ("Log file after"=w100:string)
                      n72 = local write "Log file"(w100) -> ()
                    }
                    frame #1 {
                      n73 = control-ref of="Experimental parameters tab"() -> (w102:refnum<vi>)
                      n74 = property class="TabCtl (strict)"(reference=w102, "Value"=T4."Monochromators & CCD") -> ("Pages"=w105:refnum<vi>[])  [unwired: 1 in, 2 out]
                      n75 = Index Array(array=w105, index=0) -> (element=w106:refnum<vi>)
                      n76 = property class="Page"(reference=w106, "PageVis"=TRUE ("Page Visible")) -> ()  [unwired: 1 in, 2 out]
                    }
                    frame #2 {
                      n77 = call "LFA_Initialize.vi"("Is Visible?"="LF Visible") -> ("error out"=w109:errorcluster, "LightField Automation out"=w108:refnum<class "LightField Automation.lvclass">)  [unwired: 9 in]
                    }
                    frame #3 {
                      n78 = local read "Log file"() -> (w111:string)
                      n79 = call "Write2LogFile.vi"("Add to log file"="Loading experiment settings", "Log file before"=w111) -> ("Log file after"=w112:string)
                      n80 = local write "Log file"(w112) -> ()
                      n81 = call "Exp_SetExperiment.vi"("error in (no error)"=w118, "ExperimentName"=w117, "LightField Automation in"=w116) -> ("error out"=w115:errorcluster, "LightField Automation out"=w114:refnum<class "LightField Automation.lvclass">)  [unwired: 7 in]
                    }
                    frame #4 {
                      n82 = local read "Log file"() -> (w124:string)
                      n83 = call "Write2LogFile.vi"("Add to log file"="Getting parameters", "Log file before"=w124) -> ("Log file after"=w123:string)
                      n84 = local write "Log file"(w123) -> ()
                      n85 = call "Exp_CCD_GetExposureTime.vi"("error in (no error)"=w126, "LightField Automation in"=w125) -> ("error out"=w120:errorcluster, "Exposure Time (s)"=w119:dbl, "LightField Automation out"=w121:refnum<class "LightField Automation.lvclass">)  [unwired: 7 in]
                    }
                    frame #5 {
                      n86 = call "Exp_CCD_GetTemperature.vi"("error in (no error)"=w128, "LightField Automation in"=w129) -> ("error out"=w133:errorcluster, "Temperature (°C)"=→"CCD T° :":dbl, "LightField Automation out"=w132:refnum<class "LightField Automation.lvclass">)  [unwired: 7 in]
                      n87 = call "spec_GetGratings.vi"("error in (no error)"=w133, "LightField Automation in"=w132) -> ("error out"=w142:errorcluster, "Current Grating"=w135:string, "LightField Automation out"=w143:refnum<class "LightField Automation.lvclass">)  [unwired: 6 in, 1 out]
                      n88 = local write "Grating"(w135) -> ()
                      n89 = call "spec_GetCenterWavelength.vi"("error in (no error)"=w142, "LightField Automation in"=w143) -> ("error out"=w140:errorcluster, "Center Wavelength"=w136:dbl, "LightField Automation out"=w138:refnum<class "LightField Automation.lvclass">)  [unwired: 7 in]
                      n90 = local write "Center Wavelength (nm)"(w136) -> ()
                      n91 = call "spec_getCalibration.vi"("error in (no error)"=w140, "LightField Automation in"=w138) -> ("error out"=w131:errorcluster, "ColumnCalibration"=→"Wavelength calibration":dbl[], "LightField Automation out"=w139:refnum<class "LightField Automation.lvclass">)  [unwired: 7 in]
                      n92 = local write "LightField Automation error out"(w131) -> ()
                      n93 = local write "LightField Automation out"(w139) -> ()
                      n94 = Multiply(x=w127, y=1000.0) -> (x*y=w137:dbl)
                      n95 = local write "Exposure Time (ms)"(w137) -> ()
                      n96 = local write "Acq Time (ms)"(w137) -> ()
                    }
                  }
                }
              }
            }
            frame #3 {
              # "Thorlabs USB photodiode"
              n97 = case shown="False" "PM16-120 On?" {
                frame False {
                  n98 = property on="Excitation Power (uW)" class="DigNum (strict)"("Label.BG Color"=u32 16711680 ("Label.Colors:BG Color")) -> ()  [unwired: 2 in, 2 out]
                }
                frame True {
                  # "Initialise powermeter"
                  n99 = call <instrlib>:"TLPM Find Resources.vi"("instrument handle"=refnum<visa-resource-name> refnum) -> ("error out"=w151:errorcluster, "Resource Count"=w153:u32)  [unwired: 8 in, 1 out]
                  n100 = property on="Excitation Power (uW)" class="DigNum (strict)"("Blinking"=FALSE) -> ()  [unwired: 2 in, 2 out]
                  n101 = Greater Or Equal?(x=w153, y=1) -> (x >= y?=w152:bool)
                  n102 = case shown="True" w152 {
                    tunnel: w151 -> [_ w162]
                    frame False {
                    }
                    frame True {
                      w161 = FALSE ("Reset Device (Reset Device)")
                      # "Select first Device\n(Device Index 0)"
                      n103 = call <instrlib>:"TLPM Get Resource Name.vi"("error in (no error)"=w162, "Index (0)"=u32 0) -> ("error out"=w159:errorcluster, "Resource Name"=w160:string)  [unwired: 7 in, 1 out]
                      n104 = local write "Photodiode Status"(TRUE) -> ()
                      n105 = call <instrlib>:"TLPM Initialize.vi"("error in (no error)"=w159, "Reset Device (Reset Device)"=w161, "ID Query (Do Query)"=w161, "resource name"=w160) -> ("error out"=w156:errorcluster, "instrument handle out"=w157:refnum<visa-resource-name>)  [unwired: 6 in]
                      n106 = local write "Photodiode handle out"(w157) -> ()
                      n107 = local write "Photodiode error out"(w156) -> ()
                    }
                  }
                  n108 = local read "Log file"() -> (w149:string)
                  n109 = call "Write2LogFile.vi"("Add to log file"="Initialise communication with Photodiode", "Log file before"=w149) -> ("Log file after"=w148:string)
                  n110 = local write "Log file"(w148) -> ()
                }
              }
            }
            frame #4 {
              # "Set all graph styles according to CCD Acq Mode: Spectrum or 2D Image"
              n111 = local read "Acq Mode"() -> (w163:T1)
              n112 = case shown="\"APD 1+2\"" w163 {
                frame "Image" {
                  w170 = TRUE
                  w169 = FALSE
                  n113 = property on="CCD 2D Image Main" class="IntGraph (strict)"("Visible"=w170) -> ()  [unwired: 2 in, 2 out]
                  n114 = property on="CCD 2D Image XY Map" class="IntGraph (strict)"("Visible"=w170) -> ()  [unwired: 2 in, 2 out]
                  n115 = property on="CCD 1D Spectrum Main" class="XYGraph (strict)"("Visible"=w169) -> ()  [unwired: 2 in, 2 out]
                  n116 = property on="CCD 1D Spectrum XY Map" class="WFGraph (strict)"("Visible"=w169) -> ()  [unwired: 2 in, 2 out]
                  n117 = control-ref of="Experiment Graph Controls"() -> (w167:refnum<vi>)
                  n118 = property class="TabCtl (strict)"(reference=w167) -> ("Pages"=w166:refnum<vi>[])  [unwired: 1 in, 2 out]
                  n119 = Index Array(array=w166, index=4) -> (element=w165:refnum<vi>)
                  n120 = property class="Page"(reference=w165, "PageVis"=FALSE ("Page Visible")) -> ()  [unwired: 1 in, 2 out]
                }
                frame "Spectrum" {
                  w176 = FALSE
                  w177 = TRUE
                  n121 = property on="CCD 2D Image Main" class="IntGraph (strict)"("Visible"=w176) -> ()  [unwired: 2 in, 2 out]
                  n122 = property on="CCD 2D Image XY Map" class="IntGraph (strict)"("Visible"=w176) -> ()  [unwired: 2 in, 2 out]
                  n123 = property on="CCD 1D Spectrum Main" class="XYGraph (strict)"("Visible"=w177) -> ()  [unwired: 2 in, 2 out]
                  n124 = property on="CCD 1D Spectrum XY Map" class="WFGraph (strict)"("Visible"=w177) -> ()  [unwired: 2 in, 2 out]
                  n125 = control-ref of="Experiment Graph Controls"() -> (w173:refnum<vi>)
                  n126 = property class="TabCtl (strict)"(reference=w173) -> ("Pages"=w172:refnum<vi>[])  [unwired: 1 in, 2 out]
                  n127 = Index Array(array=w172, index=4) -> (element=w171:refnum<vi>)
                  n128 = property class="Page"(reference=w171, "PageVis"=FALSE ("Page Visible")) -> ()  [unwired: 1 in, 2 out]
                }
                frame "APD 1" {
                  w183 = FALSE
                  w184 = TRUE
                  n129 = property on="CCD 2D Image Main" class="IntGraph (strict)"("Visible"=w183) -> ()  [unwired: 2 in, 2 out]
                  n130 = property on="CCD 2D Image XY Map" class="IntGraph (strict)"("Visible"=w183) -> ()  [unwired: 2 in, 2 out]
                  n131 = property on="CCD 1D Spectrum Main" class="XYGraph (strict)"("Visible"=w184) -> ()  [unwired: 2 in, 2 out]
                  n132 = property on="CCD 1D Spectrum XY Map" class="WFGraph (strict)"("Visible"=w184) -> ()  [unwired: 2 in, 2 out]
                  n133 = control-ref of="Experiment Graph Controls"() -> (w180:refnum<vi>)
                  n134 = property class="TabCtl (strict)"(reference=w180) -> ("Pages"=w179:refnum<vi>[])  [unwired: 1 in, 2 out]
                  n135 = Index Array(array=w179, index=4) -> (element=w178:refnum<vi>)
                  n136 = property class="Page"(reference=w178, "PageVis"=TRUE ("Page Visible")) -> ()  [unwired: 1 in, 2 out]
                }
                frame "APD 2" {
                  w190 = FALSE
                  w191 = TRUE
                  n137 = property on="CCD 2D Image Main" class="IntGraph (strict)"("Visible"=w190) -> ()  [unwired: 2 in, 2 out]
                  n138 = property on="CCD 2D Image XY Map" class="IntGraph (strict)"("Visible"=w190) -> ()  [unwired: 2 in, 2 out]
                  n139 = property on="CCD 1D Spectrum Main" class="XYGraph (strict)"("Visible"=w191) -> ()  [unwired: 2 in, 2 out]
                  n140 = property on="CCD 1D Spectrum XY Map" class="WFGraph (strict)"("Visible"=w191) -> ()  [unwired: 2 in, 2 out]
                  n141 = control-ref of="Experiment Graph Controls"() -> (w187:refnum<vi>)
                  n142 = property class="TabCtl (strict)"(reference=w187) -> ("Pages"=w186:refnum<vi>[])  [unwired: 1 in, 2 out]
                  n143 = Index Array(array=w186, index=4) -> (element=w185:refnum<vi>)
                  n144 = property class="Page"(reference=w185, "PageVis"=TRUE ("Page Visible")) -> ()  [unwired: 1 in, 2 out]
                }
                frame "APD 1+2" {
                  w197 = FALSE
                  w198 = TRUE
                  n145 = property on="CCD 2D Image Main" class="IntGraph (strict)"("Visible"=w197) -> ()  [unwired: 2 in, 2 out]
                  n146 = property on="CCD 2D Image XY Map" class="IntGraph (strict)"("Visible"=w197) -> ()  [unwired: 2 in, 2 out]
                  n147 = property on="CCD 1D Spectrum Main" class="XYGraph (strict)"("Visible"=w198) -> ()  [unwired: 2 in, 2 out]
                  n148 = property on="CCD 1D Spectrum XY Map" class="WFGraph (strict)"("Visible"=w198) -> ()  [unwired: 2 in, 2 out]
                  n149 = control-ref of="Experiment Graph Controls"() -> (w196:refnum<vi>)
                  n150 = property class="TabCtl (strict)"(reference=w196) -> ("Pages"=w195:refnum<vi>[])  [unwired: 1 in, 2 out]
                  n151 = Index Array(array=w195, index=4) -> (element=w194:refnum<vi>)
                  n152 = property class="Page"(reference=w194, "PageVis"=TRUE ("Page Visible")) -> ()  [unwired: 1 in, 2 out]
                }
              }
            }
            frame #5 {
              # "KCubes: 1 Shutter + 3 Piezos for XYZ microscope objective"
              n153 = case shown="True" "KCubes Piezo On?" {
                frame False {
                  n154 = control-ref of="Experimental parameters tab"() -> (w226:refnum<vi>)
                  n155 = property class="TabCtl (strict)"(reference=w226) -> ("Pages"=w229:refnum<vi>[])  [unwired: 1 in, 2 out]
                  n156 = Index Array(array=w229, index=4) -> (element=w230:refnum<vi>)
                  n157 = property class="Page"(reference=w230, "PageVis"=FALSE ("Page Visible")) -> ()  [unwired: 1 in, 2 out]
                }
                frame True {
                  n158 = stacked-sequence {
                    frame #0 {
                      n159 = local read "Log file"() -> (w232:string)
                      n160 = call "Write2LogFile.vi"("Add to log file"="Initialise communication with Piezos", "Log file before"=w232) -> ("Log file after"=w233:string)
                      n161 = local write "Log file"(w233) -> ()
                    }
                    frame #1 {
                      n162 = control-ref of="Experimental parameters tab"() -> (w236:refnum<vi>)
                      n163 = property class="TabCtl (strict)"(reference=w236) -> ("Pages"=w237:refnum<vi>[])  [unwired: 1 in, 2 out]
                      n164 = Index Array(array=w237, index=4) -> (element=w238:refnum<vi>)
                      n165 = property class="Page"(reference=w238, "PageVis"=TRUE ("Page Visible")) -> ()  [unwired: 1 in, 2 out]
                    }
                    frame #2 {
                      n166 = local read "KCubePiezoControl X"() -> (w244:refnum<k24>)
                      n167 = property class="KCubePiezoControl"(reference=w244, "SerialNumber"="29250034") -> (reference out=w242:refnum<k24>)  [unwired: 1 in, 1 out]
                      n168 = invoke class="KCubePiezoControl" method="CreateDevice"(reference=w242) -> (reference out=w241:refnum<k24>)  [unwired: 2 in, 2 out]
                      n169 = property class="KCubePiezoControl"(reference=w241) -> (reference out=w239:refnum<k24>, "Device"=w240:refnum<k24>)  [unwired: 1 in, 1 out]
                      n170 = local write "KCubePiezoDevice X Reference"(w240) -> ()
                      n171 = local write "KCubePiezoControl X Reference"(w239) -> ()
                    }
                    frame #3 {
                      n172 = local read "KCubePiezoControl Y"() -> (w245:refnum<k24>)
                      n173 = property class="KCubePiezoControl"(reference=w245, "SerialNumber"="29502721") -> (reference out=w247:refnum<k24>)  [unwired: 1 in, 1 out]
                      n174 = invoke class="KCubePiezoControl" method="CreateDevice"(reference=w247) -> (reference out=w248:refnum<k24>)  [unwired: 2 in, 2 out]
                      n175 = property class="KCubePiezoControl"(reference=w248) -> (reference out=w249:refnum<k24>, "Device"=w250:refnum<k24>)  [unwired: 1 in, 1 out]
                      n176 = local write "KCubePiezoControl Y Reference"(w249) -> ()
                      n177 = local write "KCubePiezoDevice Y Reference"(w250) -> ()
                    }
                    frame #4 {
                      n178 = local read "KCubePiezoControl Z"() -> (w252:refnum<k24>)
                      n179 = property class="KCubePiezoControl"(reference=w252, "SerialNumber"="29502682") -> (reference out=w253:refnum<k24>)  [unwired: 1 in, 1 out]
                      n180 = invoke class="KCubePiezoControl" method="CreateDevice"(reference=w253) -> (reference out=w254:refnum<k24>)  [unwired: 2 in, 2 out]
                      n181 = property class="KCubePiezoControl"(reference=w254) -> (reference out=w255:refnum<k24>, "Device"=w256:refnum<k24>)  [unwired: 1 in, 1 out]
                      n182 = local write "KCubePiezoControl Z Reference"(w255) -> ()
                      n183 = local write "KCubePiezoDevice Z Reference"(w256) -> ()
                    }
                  }
                }
              }
              n184 = case shown="True" "KCube Shutter On?" {
                frame False {
                  n185 = control-ref of="Experimental parameters tab"() -> (w205:refnum<vi>)
                  n186 = property class="TabCtl (strict)"(reference=w205) -> ("Pages"=w203:refnum<vi>[])  [unwired: 1 in, 2 out]
                  n187 = Index Array(array=w203, index=5) -> (element=w202:refnum<vi>)
                  n188 = property class="Page"(reference=w202, "PageVis"=FALSE ("Page Visible")) -> ()  [unwired: 1 in, 2 out]
                }
                frame True {
                  n189 = stacked-sequence {
                    frame #0 {
                      n190 = local read "Log file"() -> (w208:string)
                      n191 = call "Write2LogFile.vi"("Add to log file"="Initialise communication with Shutter", "Log file before"=w208) -> ("Log file after"=w207:string)
                      n192 = local write "Log file"(w207) -> ()
                    }
                    frame #1 {
                      n193 = control-ref of="Experimental parameters tab"() -> (w214:refnum<vi>)
                      n194 = property class="TabCtl (strict)"(reference=w214, "Value"=T4."Shutter options") -> ("Pages"=w212:refnum<vi>[])  [unwired: 1 in, 2 out]
                      n195 = Index Array(array=w212, index=5) -> (element=w211:refnum<vi>)
                      n196 = property class="Page"(reference=w211, "PageVis"=TRUE ("Page Visible")) -> ()  [unwired: 1 in, 2 out]
                    }
                    frame #2 {
                      n197 = Wait (ms)(milliseconds to wait=u32 50) -> ()  [unwired: 1 out]
                    }
                    frame #3 {
                      n198 = local read "KCubeSolenoidControl"() -> (w217:refnum<k24>)
                      n199 = property class="KCubeSolenoidControl"(reference=w217, "SerialNumber"="68001425") -> (reference out=w218:refnum<k24>)  [unwired: 1 in, 1 out]
                      n200 = invoke class="KCubeSolenoidControl" method="CreateDevice"(reference=w218) -> (reference out=w219:refnum<k24>)  [unwired: 2 in, 2 out]
                      n201 = property class="KCubeSolenoidControl"(reference=w219) -> (reference out=w220:refnum<k24>, "Device"=w221:refnum<k24>)  [unwired: 1 in, 1 out]
                      n202 = local write "KCubeSolenoidControl Reference"(w220) -> ()
                      n203 = invoke class="KCubeSolenoid" method="GetOperatingState"(reference=w221) -> (reference out=w222:refnum<k24>, "GetOperatingState"=w223:i32)  [unwired: 2 in, 1 out]
                      n204 = local write "KCube Shutter Device Reference"(w222) -> ()
                      n205 = case shown="2, Default" w223 {
                        frame 1 {
                          n206 = property on="Shutter Ctrls" class="Ring (strict)"("Value"=u16 5 ("Shutter Ctrls")) -> ()  [unwired: 2 in, 2 out]
                        }
                        frame 2, Default {
                          n207 = property on="Shutter Ctrls" class="Ring (strict)"("Value"=u16 0 ("Shutter Ctrls")) -> ()  [unwired: 2 in, 2 out]
                        }
                      }
                    }
                  }
                }
              }
            }
            frame #6 {
              # "ESP 300: 1 Jobin Yvon 320 Monochromator"
              n208 = case shown="True" "ESP 300 On?" {
                frame False {
                }
                frame True {
                  w266 = 1 ("Axis")
                  # "Initialise communication with ESP300"
                  n209 = local read "ESP 300 COM Port"() -> (w271:refnum<visa-resource-name>)
                  n210 = local read "ESP300 Error"() -> (w270:errorcluster)
                  n211 = local read "Log file"() -> (w260:string)
                  n212 = call "Write2LogFile.vi"("Add to log file"="Initialise communication with ESP 300", "Log file before"=w260) -> ("Log file after"=w259:string)
                  n213 = call "Init Communication.vi"("error in (no error)"=w270, "VISA resource name in"=w271) -> ("error out"=w268:errorcluster, "VISA resource name out"=w269:refnum<visa-resource-name>)  [unwired: 8 in]
                  n214 = local write "Log file"(w259) -> ()
                  n215 = call "QMotor On.vi"("error in (no error)"=w268, "Axis"=w266, "VISA resource name in"=w269) -> ("error out"=w265:errorcluster, "Motor On?"=w267:bool, "VISA resource name out"=w262:refnum<visa-resource-name>)  [unwired: 6 in]
                  n216 = local write "Mono2 On"(w267) -> ()
                  n217 = call "QPosition.vi"("error in (no error)"=w265, "Axis"=w266, "VISA resource name in"=w262) -> ("error out"=w264:errorcluster, "Position"=w261:dbl, "VISA resource name out"=w263:refnum<visa-resource-name>)  [unwired: 6 in]
                  n218 = local write "ESP 300 COM Port"(w263) -> ()
                  n219 = local write "Mono2 Motor Position"(w261) -> ()
                  n220 = local write "ESP300 Error"(w264) -> ()
                }
              }
            }
            frame #7 {
              # "448.3nm Laser Diode + Temp Controller & Driver"
              n221 = case shown="True" "Laser Comm On?" {
                frame False {
                  w273 = FALSE ("Visible")
                  n222 = property on="TEC Temperature" class="DigNum (strict)"("Visible"=w273) -> ()  [unwired: 2 in, 2 out]
                  n223 = property on="Laser on? Control" class="Bool (strict)"("Visible"=w273) -> ()  [unwired: 2 in, 2 out]
                  n224 = property on="TEC Output" class="Bool (strict)"("Visible"=w273) -> ()  [unwired: 2 in, 2 out]
                  n225 = property on="Laser Diode Current Set" class="Slide (strict)"("Visible"=w273) -> ()  [unwired: 2 in, 2 out]
                }
                frame True {
                  n226 = local read "Diode Driver Error"() -> (w282:errorcluster)
                  n227 = call <instrlib>:"TL4000 Initialize.vi"("error in (no error)"=w282, "resource name"=refnum<visa-resource-name> "USB0::0x1313::0x804F::M00549740::INSTR" ("Diode Driver COM")) -> ("error out"=w290:errorcluster, "instrument handle out"=w291:refnum<visa-resource-name>)  [unwired: 8 in]
                  n228 = call <instrlib>:"TL4000 Identification Query.vi"("error in (no error)"=w290, "instrument handle"=w291) -> ("error out"=w286:errorcluster, "instrument handle out"=w288:refnum<visa-resource-name>, "Serial Number"=→"Serial Number":string)  [unwired: 4 in, 3 out]
                  n229 = local read "Laser Diode Current Set"() -> (w293:dbl)
                  n230 = call <instrlib>:"TL4000 Beep.vi"("error in (no error)"=w286, "instrument handle"=w288) -> ("error out"=w285:errorcluster, "instrument handle out"=w287:refnum<visa-resource-name>)  [unwired: 8 in]
                  n231 = call <instrlib>:"TL4000 Get TEC Output State.vi"("error in (no error)"=w285, "instrument handle"=w287) -> ("error out"=w300:errorcluster, "TEC Output"=w274:bool, "instrument handle out"=w299:refnum<visa-resource-name>)  [unwired: 7 in]
                  n232 = property on="Laser Safety" class="Ring (strict)"("Visible"=w274) -> ()  [unwired: 2 in, 2 out]
                  n233 = property on="Laser on? Control" class="Bool (strict)"("Visible"=w274) -> ()  [unwired: 2 in, 2 out]
                  n234 = Not(x=w274) -> (.not. x?=w296:bool)
                  n235 = local write "TEC Output"(w274) -> ()
                  n236 = call <instrlib>:"TL4000 Get LD Output State.vi"("error in (no error)"=w300, "instrument handle"=w299) -> ("error out"=w297:errorcluster, "LD Output"=w301:bool, "instrument handle out"=w298:refnum<visa-resource-name>)  [unwired: 7 in]
                  n237 = local write "Laser on?"(w301) -> ()
                  n238 = call <instrlib>:"TL4000 Measure Temperature.vi"("error in (no error)"=w297, "instrument handle"=w298) -> ("error out"=w294:errorcluster, "Temperature"=w275:dbl, "instrument handle out"=w295:refnum<visa-resource-name>)  [unwired: 7 in]
                  n239 = property on="TEC Output" class="Bool (strict)"("Visible"=w296) -> ()  [unwired: 2 in, 2 out]
                  n240 = call <instrlib>:"TL4000 Set Laser Diode Current Setpoint.vi"("error in (no error)"=w294, "Laser Diode Current Setpoint (0.0)"=w293, "instrument handle"=w295) -> ("error out"=w280:errorcluster, "instrument handle out"=w279:refnum<visa-resource-name>)  [unwired: 7 in]
                  n241 = property on="Laser Diode Current Set" class="Slide (strict)"("Visible"=w274) -> ()  [unwired: 2 in, 2 out]
                  n242 = call <instrlib>:"TL4000 Set Laser Diode Current Limit.vi"("error in (no error)"=w280, "Laser Diode Current Limit (0.0)"=0.061, "instrument handle"=w279) -> ("error out"=w277:errorcluster, "instrument handle out"=w278:refnum<visa-resource-name>)  [unwired: 7 in]
                  n243 = local write "TEC Temperature"(w275) -> ()
                  n244 = call <instrlib>:"TL4000 Set Temperature Setpoint.vi"("error in (no error)"=w277, "Temperature Setpoint (25.0)"=25.0, "instrument handle"=w278) -> ("error out"=w284:errorcluster, "instrument handle out"=w283:refnum<visa-resource-name>)  [unwired: 7 in]
                  n245 = local write "Diode Driver COM"(w283) -> ()
                  n246 = local write "Diode Driver Error"(w284) -> ()
                }
              }
            }
            frame #8 {
              # "PZA12 Fine Delay Translation Stage"
              n247 = case shown="True" "PZC200 On?" {
                frame False {
                  n248 = local read "Scan LinTFine Params"() -> (w304:refnum<vi>[])
                  n249 = call "Enable&Disable_Controls.vi"("Enum"=enum16{"Enabled", "Disabled", "Disabled&Grayed"}."Disabled&Grayed", "References"=w304) -> ()  [unwired: 1 in]
                }
                frame True {
                  n250 = stacked-sequence {
                    frame #0 {
                      w306 = TRUE
                      w305 = FALSE
                      n251 = property on="Stop Contrast" class="Bool (strict)"("Visible"=w305) -> ()  [unwired: 2 in, 2 out]
                      n252 = property on="Pause Contrast" class="Bool (strict)"("Visible"=w305) -> ()  [unwired: 2 in, 2 out]
                      n253 = property on="Save Contrast" class="Bool (strict)"("Visible"=w306) -> ()  [unwired: 2 in, 2 out]
                      n254 = property on="Acquire Contrast" class="Bool (strict)"("Visible"=w306) -> ()  [unwired: 2 in, 2 out]
                      n255 = local read "Scan LinTFine Params"() -> (w308:refnum<vi>[])
                      n256 = call "Enable&Disable_Controls.vi"("Enum"=enum16{"Enabled", "Disabled", "Disabled&Grayed"}."Enabled", "References"=w308) -> ()  [unwired: 1 in]
                    }
                    frame #1 {
                      n257 = local read "PZC200 COM Port"() -> (w321:dbl)
                      n258 = call "Create Instrument Channel.vi"("XON/XOFF Handshaking(F)"=TRUE, "Baud Rate (38400)"=u32 19200, "COM Port (1)"=w321, "(T) - GPIB, F - RS232"=FALSE) -> ("Instrument Channel out"=w309:string)  [unwired: 5 in, 2 out]
                      n259 = call "SendCommand.vi"("Command"="1TS?", "Instrument Channel"=w309) -> ("error out"=w314:errorcluster)  [unwired: 8 in, 1 out]
                      n260 = call "ReadCommand.vi"("Disable MAV check (F)"=FALSE, "error in"=w314, "Instrument Channel"=w309) -> ("error out"=w311:errorcluster, "Response"=w312:string)  [unwired: 6 in, 1 out]
                      "Response" <- w312
                      n261 = String Length(string=w312) -> (length=w319:i32)
                      n262 = Subtract(x=w319, y=1) -> (x-y=w317:i32)
                      n263 = String Subset(string=w312, offset (0)=w317) -> (substring=w316:string)  [unwired: 1 in]
                      n264 = case shown="\"Q\"" w316 {
                        tunnel: w316 -> [_ _ _]
                        tunnel: [FALSE TRUE TRUE] -> w315
                        frame "@", Default {
                        }
                        frame "Q" {
                        }
                        frame "P" {
                        }
                      }
                      n265 = local write "LinTFine Motor On?"(w315) -> ()
                      n266 = call "PZCGetPos.vi"("error in"=w311, "Instrument Channel"=w309) -> ("Position"=w310:i32)  [unwired: 2 out]
                      n267 = local write "PZC Position Readout (usteps)"(w310) -> ()
                    }
                  }
                }
              }
            }
            frame #9 {
              # "Final activation message"
              n268 = property on="Experiment Graph Controls" class="TabCtl (strict)"("Value"=T2."Settings" ("Experiment Graph Controls")) -> ()  [unwired: 2 in, 2 out]
            }
          }
        }
      }
      n269 = local read "Log file"() -> (w4:string)
      n270 = call "Write2LogFile.vi"("Add to log file"=w3, "Log file before"=w4) -> ("Log file after"=w2:string)
      n271 = local write "Log file"(w2) -> ()
    }
    frame #1 {
      # "Main Program"
      n272 = while {
        stop <- w330 stop-if-true
        n273 = event shown="[30] \"Save Spectrum\", \"Save Spectrum N\", \"Save XY Map\", \"Save Polarisation\", \"Save Contrast\": Value Change" {
          selector: _ -> [_ _ _ _ _ _ _ _ _ _ _ _ _ _ _ _ _ _ _ _ _ _ _ _ _ _ _ _ _ _ _ _]
          dyn-events: _ -> [_ _ _ _ _ _ _ _ _ _ _ _ _ _ _ _ _ _ _ _ _ _ _ _ _ _ _ _ _ _ _ _]
          timeout: _ -> [_ _ _ _ _ _ _ _ _ _ _ _ _ _ _ _ _ _ _ _ _ _ _ _ _ _ _ _ _ _ _ _]
          tunnel: [w331 _ _ _ _ _ _ _ _ _ _ _ _ _ _ _ _ _ _ _ _ _ _ _ _ _ _ _ _ _ _ _] -> w330
          event "Stop Everything & Quit?": Value Change {
            n274 = event-data() -> ("NewVal"=w331:bool)  [unwired: 1 in, 5 out]
          }
          event Value Change {
            n275 = event-data() -> ()  [unwired: 1 in, 6 out]
            n276 = local read "Acq Mode"() -> (w332:T1)
            n277 = case shown="\"APD 1\"" w332 {
              frame "Image" {
                w334 = TRUE
                w335 = FALSE
                n278 = property on="CCD 1D Spectrum XY Map" class="WFGraph (strict)"("Visible"=w335) -> ()  [unwired: 2 in, 2 out]
                n279 = property on="CCD 1D Spectrum Main" class="XYGraph (strict)"("Visible"=w335) -> ()  [unwired: 2 in, 2 out]
                n280 = property on="Exit mirror" class="Enum (strict)"("Val(Sgnl)"=enum16{"CCD", "APD"}."CCD" ("Exit mirror")) -> ()  [unwired: 2 in, 2 out]
                n281 = property on="Background substract" class="Enum (strict)"("Visible"=w334) -> ()  [unwired: 2 in, 2 out]
                n282 = property on="CCD ROI" class="Enum (strict)"("Visible"=w334) -> ()  [unwired: 2 in, 2 out]
                n283 = property on="Accumulations" class="DigNum (strict)"("Visible"=w334) -> ()  [unwired: 2 in, 2 out]
                n284 = property on="CCD 2D Image Main" class="IntGraph (strict)"("Visible"=w334) -> ()  [unwired: 2 in, 2 out]
                n285 = property on="CCD 2D Image XY Map" class="IntGraph (strict)"("Visible"=w334) -> ()  [unwired: 2 in, 2 out]
                n286 = property on="Exposure Time (ms)" class="DigNum (strict)"("Visible"=w334) -> ()  [unwired: 2 in, 2 out]
              }
              frame "Spectrum" {
                w338 = FALSE
                w337 = TRUE
                n287 = property on="Exit mirror" class="Enum (strict)"("Val(Sgnl)"=enum16{"CCD", "APD"}."CCD" ("Exit mirror")) -> ()  [unwired: 2 in, 2 out]
                n288 = property on="CCD 2D Image XY Map" class="IntGraph (strict)"("Visible"=w338) -> ()  [unwired: 2 in, 2 out]
                n289 = property on="CCD 2D Image Main" class="IntGraph (strict)"("Visible"=w338) -> ()  [unwired: 2 in, 2 out]
                n290 = property on="Background substract" class="Enum (strict)"("Visible"=w337) -> ()  [unwired: 2 in, 2 out]
                n291 = property on="CCD ROI" class="Enum (strict)"("Visible"=w337) -> ()  [unwired: 2 in, 2 out]
                n292 = property on="Accumulations" class="DigNum (strict)"("Visible"=w337) -> ()  [unwired: 2 in, 2 out]
                n293 = property on="CCD 1D Spectrum XY Map" class="WFGraph (strict)"("Visible"=w337) -> ()  [unwired: 2 in, 2 out]
                n294 = property on="Exposure Time (ms)" class="DigNum (strict)"("Visible"=w337) -> ()  [unwired: 2 in, 2 out]
                n295 = property on="CCD 1D Spectrum Main" class="XYGraph (strict)"("Visible"=w337) -> ()  [unwired: 2 in, 2 out]
              }
              frame "APD 1" {
                w340 = FALSE
                w341 = TRUE
                n296 = property on="CCD 1D Spectrum XY Map" class="WFGraph (strict)"("Visible"=w341) -> ()  [unwired: 2 in, 2 out]
                n297 = property on="CCD 1D Spectrum Main" class="XYGraph (strict)"("Visible"=w341) -> ()  [unwired: 2 in, 2 out]
                n298 = property on="Exit mirror" class="Enum (strict)"("Val(Sgnl)"=enum16{"CCD", "APD"}."APD" ("Exit mirror")) -> ()  [unwired: 2 in, 2 out]
                n299 = property on="Background substract" class="Enum (strict)"("Visible"=w340) -> ()  [unwired: 2 in, 2 out]
                n300 = property on="CCD ROI" class="Enum (strict)"("Visible"=w340) -> ()  [unwired: 2 in, 2 out]
                n301 = property on="Accumulations" class="DigNum (strict)"("Visible"=w340) -> ()  [unwired: 2 in, 2 out]
                n302 = property on="CCD 2D Image Main" class="IntGraph (strict)"("Visible"=w340) -> ()  [unwired: 2 in, 2 out]
                n303 = property on="CCD 2D Image XY Map" class="IntGraph (strict)"("Visible"=w340) -> ()  [unwired: 2 in, 2 out]
                n304 = property on="Exposure Time (ms)" class="DigNum (strict)"("Visible"=w340) -> ()  [unwired: 2 in, 2 out]
              }
              frame "APD 2" {
                w343 = FALSE
                w344 = TRUE
                n305 = property on="CCD 1D Spectrum XY Map" class="WFGraph (strict)"("Visible"=w344) -> ()  [unwired: 2 in, 2 out]
                n306 = property on="CCD 1D Spectrum Main" class="XYGraph (strict)"("Visible"=w344) -> ()  [unwired: 2 in, 2 out]
                n307 = property on="Exit mirror" class="Enum (strict)"("Val(Sgnl)"=enum16{"CCD", "APD"}."APD" ("Exit mirror")) -> ()  [unwired: 2 in, 2 out]
                n308 = property on="Background substract" class="Enum (strict)"("Visible"=w343) -> ()  [unwired: 2 in, 2 out]
                n309 = property on="CCD ROI" class="Enum (strict)"("Visible"=w343) -> ()  [unwired: 2 in, 2 out]
                n310 = property on="Accumulations" class="DigNum (strict)"("Visible"=w343) -> ()  [unwired: 2 in, 2 out]
                n311 = property on="CCD 2D Image Main" class="IntGraph (strict)"("Visible"=w343) -> ()  [unwired: 2 in, 2 out]
                n312 = property on="CCD 2D Image XY Map" class="IntGraph (strict)"("Visible"=w343) -> ()  [unwired: 2 in, 2 out]
                n313 = property on="Exposure Time (ms)" class="DigNum (strict)"("Visible"=w343) -> ()  [unwired: 2 in, 2 out]
              }
              frame "APD 1+2" {
                w346 = FALSE
                w347 = TRUE
                n314 = property on="CCD 1D Spectrum XY Map" class="WFGraph (strict)"("Visible"=w347) -> ()  [unwired: 2 in, 2 out]
                n315 = property on="CCD 1D Spectrum Main" class="XYGraph (strict)"("Visible"=w347) -> ()  [unwired: 2 in, 2 out]
                n316 = property on="Exit mirror" class="Enum (strict)"("Val(Sgnl)"=enum16{"CCD", "APD"}."APD" ("Exit mirror")) -> ()  [unwired: 2 in, 2 out]
                n317 = property on="Background substract" class="Enum (strict)"("Visible"=w346) -> ()  [unwired: 2 in, 2 out]
                n318 = property on="Accumulations" class="DigNum (strict)"("Visible"=w346) -> ()  [unwired: 2 in, 2 out]
                n319 = property on="CCD ROI" class="Enum (strict)"("Visible"=w346) -> ()  [unwired: 2 in, 2 out]
                n320 = property on="CCD 2D Image Main" class="IntGraph (strict)"("Visible"=w346) -> ()  [unwired: 2 in, 2 out]
                n321 = property on="CCD 2D Image XY Map" class="IntGraph (strict)"("Visible"=w346) -> ()  [unwired: 2 in, 2 out]
                n322 = property on="Exposure Time (ms)" class="DigNum (strict)"("Visible"=w346) -> ()  [unwired: 2 in, 2 out]
              }
            }
          }
          event "FSM X Axis Pos", "FSM Y Axis Pos": Value Change {
            n323 = event-data() -> ("CtlRef"=w350:refnum<vi>, "NewVal"=w349:dbl)  [unwired: 1 in, 4 out]
            n324 = local read "FSM 300 On?"() -> (w348:bool)
            n325 = case shown="True" w348 {
              tunnel: w350 -> [_ w357]
              tunnel: w349 -> [_ w356]
              frame False {
              }
              frame True {
                w352 = 10.0 ("maximum value")
                n326 = property class="DigNum (strict)"(reference=w357) -> ("Label.Text"=w355:string)  [unwired: 1 in, 2 out]
                n327 = case shown="\"FSM X Axis Pos\", Default" w355 {
                  tunnel: [w358 w359] -> w351
                  frame "FSM Y Axis Pos" {
                    n328 = local read "FSM Y Axis"() -> (w358:tag)
                  }
                  frame "FSM X Axis Pos", Default {
                    n329 = local read "FSM X Axis"() -> (w359:tag)
                  }
                }
                n330 = Negate(x=w352) -> (-x=w353:dbl)
                n331 = call-poly <vilib>:"DAQmx Create Virtual Channel.vi"("maximum value"=w352, "minimum value"=w353, "physical channels"=w351) -> ("task out"=w354:refnum<k21>)  [unwired: 11 in, 1 out]
                n332 = call-poly <vilib>:"DAQmx Write.vi"("task/channels in"=w354, "data"=w356) -> ()  [unwired: 11 in, 3 out]
              }
            }
          }
          event "FSM Up", "FSM Down", "FSM Left", "FSM Right": Mouse Down {
            n333 = event-data() -> ("CtlRef"=w361:refnum<vi>)  [unwired: 1 in, 5 out]
            n334 = local read "FSM 300 On?"() -> (w360:bool)
            n335 = case shown="True" w360 {
              tunnel: w361 -> [_ w369]
              frame False {
              }
              frame True {
                w367 = 10.0 ("maximum value")
                n336 = property class="Bool (strict)"(reference=w369) -> ("Label.Text"=w362:string)  [unwired: 1 in, 2 out]
                n337 = local read "FSM Axis Step"() -> (w365:dbl)
                n338 = case shown="\"FSM Right\"" w362 {
                  tunnel: [w373 w377 w381 w385] -> w368
                  tunnel: w365 -> [w371 w375 w379 w383]
                  tunnel: [w370 w374 w378 w382] -> w364
                  frame "FSM Up", Default {
                    n339 = local read "FSM Y Axis Pos"() -> (w372:dbl)
                    n340 = Add(x=w372, y=w371) -> (x+y=w370:dbl)
                    n341 = local write "FSM Y Axis Pos"(w370) -> ()
                    n342 = local read "FSM Y Axis"() -> (w373:tag)
                  }
                  frame "FSM Down" {
                    n343 = local read "FSM Y Axis Pos"() -> (w376:dbl)
                    n344 = Subtract(x=w376, y=w375) -> (x-y=w374:dbl)
                    n345 = local write "FSM Y Axis Pos"(w374) -> ()
                    n346 = local read "FSM Y Axis"() -> (w377:tag)
                  }
                  frame "FSM Left" {
                    n347 = local read "FSM X Axis Pos"() -> (w380:dbl)
                    n348 = Subtract(x=w380, y=w379) -> (x-y=w378:dbl)
                    n349 = local write "FSM X Axis Pos"(w378) -> ()
                    n350 = local read "FSM X Axis"() -> (w381:tag)
                  }
                  frame "FSM Right" {
                    n351 = local read "FSM X Axis Pos"() -> (w384:dbl)
                    n352 = Add(x=w384, y=w383) -> (x+y=w382:dbl)
                    n353 = local write "FSM X Axis Pos"(w382) -> ()
                    n354 = local read "FSM X Axis"() -> (w385:tag)
                  }
                }
                n355 = Negate(x=w367) -> (-x=w366:dbl)
                n356 = call-poly <vilib>:"DAQmx Create Virtual Channel.vi"("maximum value"=w367, "minimum value"=w366, "physical channels"=w368) -> ("task out"=w363:refnum<k21>)  [unwired: 11 in, 1 out]
                n357 = call-poly <vilib>:"DAQmx Write.vi"("task/channels in"=w363, "data"=w364) -> ()  [unwired: 11 in, 3 out]
              }
            }
          }
          event "Conv/Energy (eV)", "Conv/Wavelength (nm)", "Conv/Time (s)", "Conv/Wavenumber (m-1)": Value Change {
            n358 = event-data() -> ("CtlRef"=w388:refnum<vi>, "NewVal"=w386:dbl)  [unwired: 1 in, 4 out]
            n359 = property class="DigNum (strict)"(reference=w388) -> ("Label.Text"=w387:string)  [unwired: 1 in, 2 out]
            n360 = case shown="\"Conv/Wavenumber (m-1)\"" w387 {
              tunnel: w386 -> [w396 _ w409 _]
              frame "Conv/Wavelength (nm)", Default {
                n361 = Multiply(x=w396, y=1e-09) -> (x*y=w394:dbl)
                n362 = Divide(x=1.0, y=w394) -> (x/y=w391:dbl)
                n363 = Divide(x=w394, y=299792458.0) -> (x/y=w393:dbl)
                n364 = Divide(x=w391, y=100.0) -> (x/y=w389:dbl)
                n365 = Divide(x=1239.841, y=w396) -> (x/y=w398:dbl)
                n366 = local write "Conv/Energy (eV)"(w398) -> ()
                n367 = local write "Conv/Wavenumber (m-1)"(w389) -> ()
                n368 = local write "Conv/Time (s)"(w393) -> ()
              }
              frame "Conv/Time (s)" {
              }
              frame "Conv/Energy (eV)" {
                n369 = Divide(x=1239.841, y=w409) -> (x/y=w408:dbl)
                n370 = Multiply(x=w408, y=1e-09) -> (x*y=w405:dbl)
                n371 = local write "Conv/Wavelength (nm)"(w408) -> ()
                n372 = Divide(x=1.0, y=w405) -> (x/y=w402:dbl)
                n373 = Divide(x=w402, y=100.0) -> (x/y=w400:dbl)
                n374 = Divide(x=w405, y=299792458.0) -> (x/y=w403:dbl)
                n375 = local write "Conv/Wavenumber (m-1)"(w400) -> ()
                n376 = local write "Conv/Time (s)"(w403) -> ()
              }
              frame "Conv/Wavenumber (m-1)" {
              }
            }
          }
          event "FSM Home": Mouse Down {
            w415 = 0.0 ("FSM X Axis Pos")
            w416 = 0.0 ("FSM X Axis Pos")
            n377 = event-data() -> ()  [unwired: 1 in, 6 out]
            n378 = local read "FSM X Axis"() -> (w417:tag)
            n379 = local read "FSM Y Axis"() -> (w414:tag)
            n380 = Negate(x=10.0 ("maximum value")) -> (-x=w411:dbl)
            n381 = Negate(x=10.0 ("maximum value")) -> (-x=w420:dbl)
            n382 = call-poly <vilib>:"DAQmx Create Virtual Channel.vi"("minimum value"=w411, "physical channels"=w414) -> ("task out"=w413:refnum<k21>)  [unwired: 12 in, 1 out]
            n383 = call-poly <vilib>:"DAQmx Create Virtual Channel.vi"("minimum value"=w420, "physical channels"=w417) -> ("task out"=w418:refnum<k21>)  [unwired: 12 in, 1 out]
            n384 = local write "FSM Y Axis Pos"(w415) -> ()
            n385 = local write "FSM X Axis Pos"(w416) -> ()
            n386 = call-poly <vilib>:"DAQmx Write.vi"("task/channels in"=w413, "data"=w415) -> ()  [unwired: 11 in, 3 out]
            n387 = call-poly <vilib>:"DAQmx Write.vi"("task/channels in"=w418, "data"=w416) -> ()  [unwired: 11 in, 3 out]
          }
          event "Exit mirror": Value Change {
            n388 = event-data() -> ("NewVal"=w422:enum16{"CCD", "APD"})  [unwired: 1 in, 5 out]
            n389 = case shown="\"CCD\"" w422 {
              tunnel: ["uPL" w455] -> w425
              tunnel: [TRUE FALSE] -> w424
              tunnel: ["CCD" w455] -> w421
              frame "CCD" {
                # "mono + CCD"
              }
              frame "APD" {
                w455 = "APD"
                # "mono only\nAPD exit port"
              }
            }
            n390 = local read "LightField Automation error out"() -> (w428:errorcluster)
            n391 = local read "LightField Automation out"() -> (w429:refnum<class "LightField Automation.lvclass">)
            n392 = stacked-sequence {
              seq-local: [w438 _ _] -> [_ w444 _]
              seq-local: [w437 _ _] -> [_ w443 _]
              seq-local: [w436 _ _] -> [_ w440 _]
              seq-local: [w435 _ _] -> [_ w439 _]
              seq-local: [_ w442 _] -> [_ _ w451]
              seq-local: [_ w441 _] -> [_ _ w450]
              seq-local: [_ w439 _] -> [_ _ w447]
              tunnel: w429 -> [w438 _ _]
              tunnel: w428 -> [w437 _ _]
              tunnel: w425 -> [w436 _ _]
              tunnel: w421 -> [w435 _ _]
              tunnel: [_ _ w451] -> w427
              tunnel: [_ _ w450] -> w426
              frame #0 {
                n393 = local read "Log file"() -> (w433:string)
                n394 = call "Write2LogFile.vi"("Add to log file"="Changing SpectraPro HRS-500 exit port ...", "Log file before"=w433) -> ("Log file after"=w434:string)
                n395 = local write "Log file"(w434) -> ()
              }
              frame #1 {
                n396 = call "Exp_SetExperiment.vi"("error in (no error)"=w443, "ExperimentName"=w440, "LightField Automation in"=w444) -> ("error out"=w442:errorcluster, "LightField Automation out"=w441:refnum<class "LightField Automation.lvclass">)  [unwired: 7 in]
              }
              frame #2 {
                n397 = local read "Log file"() -> (w449:string)
                n398 = Concatenate Strings("SpectraPro HRS-500 exit mirror set to " ("string"), w447) -> (w445:string)
                n399 = call "Write2LogFile.vi"("Add to log file"=w445, "Log file before"=w449) -> ("Log file after"=w448:string)
                n400 = local write "Log file"(w448) -> ()
              }
            }
            n401 = call "spec_GetOpticalExitPort.vi"("error in (no error)"=w427, "LightField Automation in"=w426) -> ("error out"=w430:errorcluster, "Exit Port Location"=→"Exit Port Location":T6, "LightField Automation out"=w431:refnum<class "LightField Automation.lvclass">)  [unwired: 7 in]
            n402 = local write "LightField Automation error out"(w430) -> ()
            n403 = local write "LightField Automation out"(w431) -> ()
            n404 = property on="Exposure Time (ms)" class="DigNum (strict)"("Visible"=w424) -> ()  [unwired: 2 in, 2 out]
          }
          event "Mono2 On": Value Change {
            n405 = event-data() -> ("NewVal"=w457:bool)  [unwired: 1 in, 5 out]
            n406 = case shown="True" w457 {
              frame False {
                n407 = stacked-sequence {
                  frame #0 {
                    n408 = local read "ESP 300 COM Port"() -> (w461:refnum<visa-resource-name>)
                    n409 = local read "ESP300 Error"() -> (w462:errorcluster)
                    n410 = call "Motor Off.vi"("error in (no error)"=w462, "Axis"=1, "VISA resource name in"=w461) -> ("error out"=w459:errorcluster, "VISA resource name out"=w458:refnum<visa-resource-name>)  [unwired: 7 in]
                    n411 = local write "ESP 300 COM Port"(w458) -> ()
                    n412 = local write "ESP300 Error"(w459) -> ()
                  }
                  frame #1 {
                    n413 = local read "Log file"() -> (w464:string)
                    n414 = call "Write2LogFile.vi"("Add to log file"="Mono2 motor turned off", "Log file before"=w464) -> ("Log file after"=w465:string)
                    n415 = local write "Log file"(w465) -> ()
                  }
                }
              }
              frame True {
                n416 = stacked-sequence {
                  frame #0 {
                    n417 = local read "ESP 300 COM Port"() -> (w469:refnum<visa-resource-name>)
                    n418 = local read "ESP300 Error"() -> (w470:errorcluster)
                    n419 = call "Motor On.vi"("error in (no error)"=w470, "Axis"=1, "VISA resource name in"=w469) -> ("error out"=w467:errorcluster, "VISA resource name out"=w466:refnum<visa-resource-name>)  [unwired: 7 in]
                    n420 = local write "ESP 300 COM Port"(w466) -> ()
                    n421 = local write "ESP300 Error"(w467) -> ()
                  }
                  frame #1 {
                    n422 = local read "Log file"() -> (w472:string)
                    n423 = call "Write2LogFile.vi"("Add to log file"="Mono2 motor turned on", "Log file before"=w472) -> ("Log file after"=w473:string)
                    n424 = local write "Log file"(w473) -> ()
                  }
                }
              }
            }
          }
          event "Excitation Power (uW)": Mouse Down; "Excitation Wavelength (nm)": Value Change {
            n425 = event-data() -> ()  [unwired: 1 in, 4 out]
            n426 = local read "Excitation Wavelength (nm)"() -> (w480:dbl)
            n427 = local read "Photodiode handle out"() -> (w481:refnum<visa-resource-name>)
            n428 = local read "Photodiode error out"() -> (w479:errorcluster)
            n429 = call <instrlib>:"TLPM Set Wavelength.vi"("error in (no error)"=w479, "Wavelength (0.0)"=w480, "instrument handle"=w481) -> ("error out"=w478:errorcluster, "instrument handle out"=w477:refnum<visa-resource-name>)  [unwired: 7 in]
            n430 = call <instrlib>:"TLPM Measure Power.vi"("error in (no error)"=w478, "instrument handle"=w477) -> ("error out"=w474:errorcluster, "Power"=w476:dbl, "instrument handle out"=w475:refnum<visa-resource-name>)  [unwired: 7 in]
            n431 = local write "Photodiode handle out"(w475) -> ()
            n432 = local write "Excitation Power (uW)"(w476) -> ()
            n433 = local write "Photodiode error out"(w474) -> ()
          }
          event "CCD 1D Spectrum Main", "Polarisation 1D Spectrum": Scale Range Change {
            n434 = event-data() -> ("CtlRef"=w483:refnum<vi>, "ScaleRef"=w485:refnum<vi>, "NewRange"=w482:T13)  [unwired: 1 in, 5 out]
            n435 = property class="GrphScl"(reference=w485) -> ("NameLbl.Text"=w484:string)  [unwired: 1 in, 2 out]
            n436 = case shown="\"PL Intensity (cts)\", Default" w484 {
              tunnel: w483 -> [w488 _]
              tunnel: w482 -> [w486 _]
              frame "Energy (eV)" {
                w487 = 1239.841
                n437 = property class="XYGraph (strict)"(reference=w488) -> ("Label.Text"=w493:string)  [unwired: 1 in, 2 out]
                n438 = Unbundle By Name(w486) -> ("Minimum"=w490:dbl, "Maximum"=w489:dbl)
                n439 = Divide(x=w487, y=w490) -> (x/y=w491:dbl)
                n440 = Divide(x=w487, y=w489) -> (x/y=w492:dbl)
                n441 = case shown="\"Polarisation 1D Spectrum\"" w493 {
                  tunnel: w491 -> [w495 w497]
                  tunnel: w492 -> [w494 w496]
                  frame "CCD 1D Spectrum Main", Default {
                    n442 = property on="CCD 1D Spectrum Main Energy Scale" class="XYGraph (strict)"("XScale.Maximum"=w495, "XScale.Minimum"=w494) -> ()  [unwired: 2 in, 2 out]
                  }
                  frame "Polarisation 1D Spectrum" {
                    n443 = property on="Polarisation 1D Spectrum Energy Scale" class="XYGraph (strict)"("XScale.Maximum"=w497, "XScale.Minimum"=w496) -> ()  [unwired: 2 in, 2 out]
                  }
                }
              }
              frame "PL Intensity (cts)", Default {
              }
            }
          }
          event "Full scale": Mouse Down {
            w502 = 1239.84
            n444 = event-data() -> ()  [unwired: 1 in, 8 out]
            n445 = property on="CCD 1D Spectrum Main" class="XYGraph (strict)"("XScale.ScaleFit"=u8 1 ("X Scale.Scale Fit")) -> ("XScale.Minimum"=w501:dbl, "XScale.Maximum"=w500:dbl)  [unwired: 2 in, 2 out]
            n446 = Divide(x=w502, y=w501) -> (x/y=w499:dbl)
            n447 = Divide(x=w502, y=w500) -> (x/y=w498:dbl)
            n448 = property on="CCD 1D Spectrum Main Energy Scale" class="XYGraph (strict)"("XScale.Maximum"=w499, "XScale.Minimum"=w498) -> ()  [unwired: 2 in, 2 out]
          }
          event "Grating": Value Change {
            n449 = event-data() -> ("NewVal"=w512:string)  [unwired: 1 in, 5 out]
            n450 = local read "LightField Automation error out"() -> (w513:errorcluster)
            n451 = local read "LightField Automation out"() -> (w514:refnum<class "LightField Automation.lvclass">)
            n452 = stacked-sequence {
              seq-local: [w520 _ _] -> [_ w525 _]
              seq-local: [w519 _ _] -> [_ w524 _]
              seq-local: [w518 _ _] -> [_ w521 _]
              seq-local: [_ w523 _] -> [_ _ w532]
              seq-local: [_ w522 _] -> [_ _ w531]
              seq-local: [_ w521 _] -> [_ _ w529]
              tunnel: w514 -> [w520 _ _]
              tunnel: w513 -> [w519 _ _]
              tunnel: w512 -> [w518 _ _]
              tunnel: [_ _ w532] -> w508
              tunnel: [_ _ w531] -> w507
              frame #0 {
                n453 = local read "Log file"() -> (w516:string)
                n454 = call "Write2LogFile.vi"("Add to log file"="Changing grating ...", "Log file before"=w516) -> ("Log file after"=w517:string)
                n455 = local write "Log file"(w517) -> ()
              }
              frame #1 {
                n456 = call "spec_SetGrating.vi"("error in (no error)"=w524, "GratingSelected"=w521, "LightField Automation in"=w525) -> ("error out"=w522:errorcluster, "LightField Automation out"=w523:refnum<class "LightField Automation.lvclass">)  [unwired: 7 in]
              }
              frame #2 {
                n457 = local read "Log file"() -> (w528:string)
                n458 = Concatenate Strings("Grating changed to" ("string"), w529) -> (w527:string)
                n459 = call "Write2LogFile.vi"("Add to log file"=w527, "Log file before"=w528) -> ("Log file after"=w526:string)
                n460 = local write "Log file"(w526) -> ()
              }
            }
            n461 = call "spec_GetCenterWavelength.vi"("error in (no error)"=w507, "LightField Automation in"=w508) -> ("error out"=w506:errorcluster, "Center Wavelength"=w504:dbl, "LightField Automation out"=w505:refnum<class "LightField Automation.lvclass">)  [unwired: 7 in]
            n462 = local write "Center Wavelength (nm)"(w504) -> ()
            n463 = call "spec_getCalibration.vi"("error in (no error)"=w506, "LightField Automation in"=w505) -> ("error out"=w510:errorcluster, "ColumnCalibration"=w509:dbl[], "LightField Automation out"=w511:refnum<class "LightField Automation.lvclass">)  [unwired: 7 in]
            n464 = local write "LightField Automation out"(w511) -> ()
            n465 = local write "Wavelength calibration"(w509) -> ()
            n466 = local write "LightField Automation error out"(w510) -> ()
          }
          event "Acquire Spectrum", "Acquire Continuous Spectrum", "Acquire Polarisation", "Acquire XY Map", "Acquire Contrast": Mouse Down {
            # "Launch an acquisition or an experiment"
            n467 = event-data() -> ("CtlRef"=w533:refnum<vi>)  [unwired: 1 in, 7 out]
            n468 = stacked-sequence {
              tunnel: w533 -> [w537 w867]
              frame #0 {
                # "Actual measurements"
                n469 = local read "LightField Automation out"() -> (w540:refnum<class "LightField Automation.lvclass">)
                n470 = local read "LightField Automation error out"() -> (w541:errorcluster)
                n471 = property class="Bool (strict)"(reference=w537) -> ("Label.Text"=w538:string)  [unwired: 1 in, 2 out]
                n472 = local read "Accumulations"() -> (w539:dbl)
                n473 = local read "CCD ROI"() -> (w535:T5)
                n474 = case shown="\"Acquire Polarisation\"" w538 {
                  tunnel: [w544 w587 w693 w748 w784 w847] -> w536
                  tunnel: [w545 w584 w692 w747 w783 w846] -> w534
                  tunnel: w541 -> [w548 w585 w694 w749 w785 w846]
                  tunnel: w540 -> [w547 w586 w695 w750 w786 w847]
                  tunnel: w539 -> [w546 w588 w690 _ _ _]
                  tunnel: w535 -> [w542 w583 w691 _ _ _]
                  frame "Acquire Spectrum", Default {
                    n475 = call "Adv_SetROI.vi"("error in (no error)"=w548, "ROI"=w542, "LightField Automation in"=w547) -> ("error out"=w549:errorcluster, "LightField Automation out"=w550:refnum<class "LightField Automation.lvclass">)  [unwired: 7 in]
                    n476 = stacked-sequence {
                      seq-local: [w559 _ _] -> [_ w567 _]
                      seq-local: [w558 _ _] -> [_ w562 _]
                      seq-local: [w557 _ _] -> [_ w566 _]
                      tunnel: w550 -> [w559 _ _]
                      tunnel: w549 -> [w558 _ _]
                      tunnel: w546 -> [w557 _ _]
                      tunnel: [_ w565 _] -> w545
                      tunnel: [_ w564 _] -> w544
                      tunnel: [_ w563 _] -> w543
                      frame #0 {
                        # "open shutter"
                        n477 = control-ref of="Shutter Ctrls"() -> (w555:refnum<vi>)
                        n478 = property class="Ring (strict)"(reference=w555) -> ("Value"=w554:u16)  [unwired: 1 in, 2 out]
                        n479 = control-ref of="KCube Shutter Device Reference"() -> (w556:refnum<vi>)
                        n480 = Equal?(x=w554, y=u16 0) -> (x = y?=w552:bool)
                        n481 = case shown="True" w552 {
                          tunnel: w556 -> [_ w561]
                          tunnel: w555 -> [_ w560]
                          frame False {
                          }
                          frame True {
                            n482 = call "Shutter.vi"("KCube Shutter Device Reference 2"=w561, "Shutter Ctrls 2"=w560) -> ()
                          }
                        }
                      }
                      frame #1 {
                        # "acquire"
                        n483 = call "LFA_Capture.vi"("error in (no error)"=w562, "Frames"=w566, "LightField Automation in"=w567) -> ("error out"=w565:errorcluster, "Data"=w563:T3, "LightField Automation out"=w564:refnum<class "LightField Automation.lvclass">)  [unwired: 6 in]
                      }
                      frame #2 {
                        # "close shutter"
                        n484 = control-ref of="Shutter Ctrls"() -> (w569:refnum<vi>)
                        n485 = control-ref of="KCube Shutter Device Reference"() -> (w568:refnum<vi>)
                        n486 = call "Shutter.vi"("KCube Shutter Device Reference 2"=w568, "Shutter Ctrls 2"=w569) -> ()
                      }
                    }
                    "Data" <- w543
                    n487 = local read "Acq Mode"() -> (w551:T1)
                    n488 = case shown="\"Image\"" w551 {
                      selector: w551 -> [w575 w580]
                      tunnel: w543 -> [w577 w582]
                      frame "Spectrum", Default {
                        n489 = local read "Wavelength calibration"() -> (w574:dbl[])
                        n490 = Divide(x=1239.841, y=w574) -> (x/y=w572:dbl[])
                        n491 = call "PrepareData4Graph.vi"("Wavelength nm"=w572, "DataLF"=w577, "AcqMode"=w575, "Data type"=T9."Spectre") -> ("Spectrum"=w576:cluster{"Array 2":dbl[], "Array":dbl[]})  [unwired: 2 in, 3 out]
                        n492 = local write "CCD 1D Spectrum Main"(w576) -> ()
                        n493 = property on="Experiment Graph Controls" class="TabCtl (strict)"("Value"=T2."Spectrum Acquisition" ("Experiment Graph Controls")) -> ()  [unwired: 2 in, 2 out]
                      }
                      frame "Image" {
                        n494 = local read "Wavelength calibration"() -> (w581:dbl[])
                        n495 = call "PrepareData4Graph.vi"("Wavelength nm"=w581, "DataLF"=w582, "AcqMode"=w580, "Data type"=T9."Spectre") -> ("Intensity Graph"=w579:dbl[][])  [unwired: 2 in, 3 out]
                        n496 = local write "CCD 2D Image Main"(w579) -> ()
                      }
                    }
                  }
                  frame "Acquire Contrast EVERYTHING OK BUT NO SUBVI" {
                    n497 = stacked-sequence {
                      tunnel: w588 -> [_ w608 _]
                      tunnel: [_ w607 _] -> w587
                      tunnel: w586 -> [_ w600 _]
                      tunnel: w585 -> [_ w599 _]
                      tunnel: [_ w595 _] -> w584
                      tunnel: w583 -> [_ w592 _]
                      frame #0 {
                        n498 = property on="Experiment Graph Controls" class="TabCtl (strict)"("Value"=T2."Contrast Acquisition" ("Experiment Graph Controls")) -> (error out=w590:errorcluster)  [unwired: 2 in, 1 out]
                        n499 = property on="Acquire Contrast" class="Bool (strict)"(error in=w590, "Visible"=FALSE) -> ()  [unwired: 1 in, 2 out]
                      }
                      frame #1 {
                        # "fine interferogram"
                        # "Spectra"
                        # "Position PZA12"
                        n500 = local read "LinTFines Step Pos (usteps)"() -> (w601:dbl)
                        n501 = call "Adv_SetROI.vi"("error in (no error)"=w599, "ROI"=w592, "LightField Automation in"=w600) -> ("error out"=w598:errorcluster, "LightField Automation out"=w597:refnum<class "LightField Automation.lvclass">)  [unwired: 7 in]
                        n502 = local read "LinTFine Start Pos (usteps)"() -> (w602:dbl)
                        n503 = local read "LinTFine End Pos (usteps)"() -> (w618:dbl)
                        n504 = local read "PZC200 Instrument Channel"() -> (w611:string)
                        n505 = Number To Decimal String(number=w601) -> (decimal integer string=w613:string)  [unwired: 1 in]
                        n506 = Subtract(x=w618, y=w602) -> (x-y=w617:dbl)
                        n507 = local read "PZC Error"() -> (w610:errorcluster)
                        n508 = Divide(x=w617, y=w601) -> (x/y=w616:dbl)
                        n509 = Concatenate Strings("1PR", w613) -> (w593:string)
                        n510 = Add(x=w616, y=1.0) -> (x+y=w614:dbl)
                        n511 = for {
                          N: w614 -> [_]
                          tunnel: w611 -> [w648]
                          tunnel: w593 -> [w649]
                          shift-right: [w646] -> w609
                          shift-left: w610 -> [w647]
                          shift-right: [w644] -> w607
                          shift-left: w597 -> [w645]
                          shift-right: [w642] -> w595
                          shift-left: w598 -> [w643]
                          tunnel: w608 -> [w641]
                          shift-right: [w634] -> w596
                          shift-left: dbl[][] [] -> [w632]
                          shift-right: [w631] -> _
                          shift-left: dbl[] [] -> [w633]
                          shift-right: [w627] -> w603
                          shift-left: dbl[] [] -> [w629]
                          tunnel: w602 -> [w626]
                          tunnel: w601 -> [w624]
                          tunnel: [FALSE] -> w594
                          i -> [w625]
                          n512 = Multiply(x=w625, y=w624) -> (x*y=w623:dbl)
                          n513 = Add(x=w626, y=w623) -> (x+y=w622:dbl)
                          n514 = stacked-sequence {
                            seq-local: [w655 _ _ _ _ _] -> [_ w657 _ _ _ _]
                            seq-local: [w654 _ _ _ _ _] -> [_ w656 _ _ _ _]
                            seq-local: [_ w657 _ _ _ _] -> [_ _ w664 _ _ _]
                            seq-local: [_ w656 _ _ _ _] -> [_ _ w663 _ _ _]
                            seq-local: [_ _ w666 _ _ _] -> [_ _ _ w672 _ _]
                            seq-local: [_ _ _ w672 _ _] -> [_ _ _ _ w681 _]
                            seq-local: [_ _ _ _ w681 _] -> [_ _ _ _ _ w684]
                            tunnel: w649 -> [w653 _ _ _ _ _]
                            tunnel: w647 -> [w652 _ _ _ _ _]
                            tunnel: w648 -> [w651 _ _ _ _ _]
                            tunnel: [_ _ w665 _ _ _] -> w650
                            tunnel: w633 -> [_ _ w662 _ _ _]
                            tunnel: [_ _ w660 _ _ _] -> w631
                            tunnel: w622 -> [_ _ w659 _ _ _]
                            tunnel: w645 -> [_ _ _ _ w680 _]
                            tunnel: [_ _ _ _ w678 _] -> w644
                            tunnel: w643 -> [_ _ _ _ w675 _]
                            tunnel: [_ _ _ _ w676 _] -> w642
                            tunnel: w641 -> [_ _ _ _ w679 _]
                            tunnel: [_ _ _ _ w677 _] -> w640
                            tunnel: [_ _ _ _ _ w684] -> w646
                            frame #0 {
                              # "move piezo"
                              n515 = call "SendCommand.vi"("error in"=w652, "Command"=w653, "Instrument Channel"=w651) -> ("error out"=w654:errorcluster, "Instrument Channel out"=w655:string)  [unwired: 7 in]
                            }
                            frame #1 {
                              # "wait"
                              n516 = Wait (ms)(milliseconds to wait=u32 50) -> ()  [unwired: 1 out]
                            }
                            frame #2 {
                              # "get position"
                              n517 = Insert Into Array(array=w662, new element=w659) -> (w660:dbl[])  [unwired: 1 in]
                              n518 = call "PZCGetPos.vi"("error in"=w663, "Instrument Channel"=w664) -> ("Instrument Channel Out"=w665:string, "Position"=w661:i32, "error out"=w666:errorcluster)
                              n519 = local write "PZC Position Readout (usteps)"(w661) -> ()
                            }
                            frame #3 {
                              # "open shutter"
                              n520 = control-ref of="Shutter Ctrls"() -> (w670:refnum<vi>)
                              n521 = property class="Ring (strict)"(reference=w670) -> ("Value"=w669:u16)  [unwired: 1 in, 2 out]
                              n522 = control-ref of="KCube Shutter Device Reference"() -> (w671:refnum<vi>)
                              n523 = Equal?(x=w669, y=u16 0) -> (x = y?=w668:bool)
                              n524 = case shown="True" w668 {
                                tunnel: w671 -> [_ w674]
                                tunnel: w670 -> [_ w673]
                                frame False {
                                }
                                frame True {
                                n525 = call "Shutter.vi"("KCube Shutter Device Reference 2"=w674, "Shutter Ctrls 2"=w673) -> ()
                                }
                              }
                            }
                            frame #4 {
                              # "acquire"
                              n526 = call "LFA_Capture.vi"("error in (no error)"=w675, "Frames"=w679, "LightField Automation in"=w680) -> ("error out"=w676:errorcluster, "Data"=w677:T3, "LightField Automation out"=w678:refnum<class "LightField Automation.lvclass">)  [unwired: 6 in]
                            }
                            frame #5 {
                              # "close shutter"
                              n527 = control-ref of="Shutter Ctrls"() -> (w683:refnum<vi>)
                              n528 = control-ref of="KCube Shutter Device Reference"() -> (w682:refnum<vi>)
                              n529 = call "Shutter.vi"("KCube Shutter Device Reference 2"=w682, "Shutter Ctrls 2"=w683) -> ()
                            }
                          }
                          n530 = local write "PZC200 Instrument Channel"(w650) -> ()
                          n531 = local read "Wavelength calibration"() -> (w637:dbl[])
                          n532 = Divide(x=1239.841, y=w637) -> (x/y=w636:dbl[])
                          n533 = call "PrepareData4Graph.vi"("Wavelength nm"=w636, "DataLF"=w640, "AcqMode"=T10."Spectrum", "Data type"=T9."Spectre") -> ("Spectrum"=w635:cluster{"Array 2":dbl[], "Array":dbl[]}, "PLInt out"=w630:dbl[])  [unwired: 2 in, 2 out]
                          n534 = Add Array Elements(numeric array=w630) -> (sum=w628:dbl)
                          n535 = Insert Into Array(array=w629, new element=w628) -> (w627:dbl[])  [unwired: 1 in]
                          n536 = Bundle(w631, w627) -> (w621:cluster{dbl[], dbl[]})  [unwired: 1 in]
                          n537 = local write "Contrast Oscillations"(w621) -> ()
                          n538 = local write "Contrast 1D Spectrum"(w635) -> ()
                          n539 = Insert Into Array(array=w632, new element=w630) -> (w634:dbl[][])  [unwired: 2 in]
                        }
                        "Contrast Oscill data" <- w603
                        n540 = local write "Acquire Contrast"(w594) -> ()
                        n541 = local write "Contrast Array Out"(w596) -> ()
                        n542 = local write "PZC Error"(w609) -> ()
                      }
                      frame #2 {
                        n543 = property on="Acquire Contrast" class="Bool (strict)"("Visible"=TRUE) -> ()  [unwired: 2 in, 2 out]
                        n544 = property on="CCD 1D Spectrum Main" class="XYGraph (strict)"() -> ("XScale.Maximum"=w688:dbl, "XScale.Minimum"=w687:dbl, "YScale.Minimum"=w686:dbl, "YScale.Maximum"=w685:dbl)  [unwired: 2 in, 2 out]
                        n545 = property on="Contrast 1D Spectrum" class="XYGraph (strict)"("XScale.Maximum"=w688, "XScale.Minimum"=w687, "YScale.Minimum"=w686, "YScale.Maximum"=w685) -> ()  [unwired: 2 in, 2 out]
                      }
                    }
                  }
                  frame "Acquire Contrast" {
                    n546 = stacked-sequence {
                      tunnel: w695 -> [_ w727 _]
                      tunnel: w694 -> [_ w725 _]
                      tunnel: [_ w730 _] -> w693
                      tunnel: [_ w731 _] -> w692
                      tunnel: w691 -> [_ w708 _]
                      tunnel: w690 -> [_ w716 _]
                      frame #0 {
                        w703 = FALSE
                        w706 = TRUE
                        n547 = property on="Stop Contrast" class="Bool (strict)"("Visible"=w706) -> ()  [unwired: 2 in, 2 out]
                        n548 = property on="Pause Contrast" class="Bool (strict)"("Visible"=w706) -> ()  [unwired: 2 in, 2 out]
                        n549 = local read "Scan LinTFine Params"() -> (w704:refnum<vi>[])
                        n550 = property on="Experiment Graph Controls" class="TabCtl (strict)"("Value"=T2."Contrast Acquisition" ("Experiment Graph Controls")) -> ()  [unwired: 2 in, 2 out]
                        n551 = property on="Save Contrast" class="Bool (strict)"("Visible"=w703) -> ()  [unwired: 2 in, 2 out]
                        n552 = property on="Acquire Contrast" class="Bool (strict)"("Visible"=w703) -> ()  [unwired: 2 in, 2 out]
                        n553 = call "Enable&Disable_Controls.vi"("Enum"=enum16{"Enabled", "Disabled", "Disabled&Grayed"}."Disabled&Grayed", "References"=w704) -> ()  [unwired: 1 in]
                        n554 = property on="CCD 1D Spectrum Main" class="XYGraph (strict)"() -> ("XScale.Maximum"=w701:dbl, "XScale.Minimum"=w700:dbl, "YScale.Minimum"=w699:dbl, "YScale.Maximum"=w698:dbl)  [unwired: 2 in, 2 out]
                        n555 = property on="Scan Linear Stage Progess Bar" class="Slide (strict)"("Visible"=TRUE, "Value"=u8 0 ("Scan Linear Stage Progess Bar")) -> ()  [unwired: 2 in, 2 out]
                        n556 = property on="Contrast 1D Spectrum" class="XYGraph (strict)"("XScale.Maximum"=w701, "XScale.Minimum"=w700, "YScale.Minimum"=w699, "YScale.Maximum"=w698) -> ()  [unwired: 2 in, 2 out]
                      }
                      frame #1 {
                        n557 = local read "LinTFines Step Pos (usteps)"() -> (w712:dbl)
                        n558 = local read "LinTFine Start Pos (usteps)"() -> (w714:dbl)
                        n559 = local read "LinTFine End Pos (usteps)"() -> (w713:dbl)
                        n560 = local read "Exposure Time (ms)"() -> (w709:dbl)
                        n561 = local read "Acq Mode"() -> (w707:T1)
                        n562 = control-ref of="KCube Shutter Device Reference"() -> (w717:refnum<vi>)
                        n563 = local read "PZC200 Instrument Channel"() -> (w715:string)
                        n564 = control-ref of="PZC Position Readout (usteps)"() -> (w724:refnum<vi>)
                        n565 = control-ref of="Scan Linear Stage Progess Bar"() -> (w723:refnum<vi>)
                        n566 = control-ref of="Contrast 1D Spectrum"() -> (w720:refnum<vi>)
                        n567 = control-ref of="Contrast Oscillations"() -> (w721:refnum<vi>)
                        n568 = control-ref of="Pause Contrast"() -> (w722:refnum<vi>)
                        n569 = control-ref of="Stop Contrast"() -> (w719:refnum<vi>)
                        n570 = local read "PZC Error"() -> (w726:errorcluster)
                        n571 = control-ref of="Shutter Ctrls"() -> (w718:refnum<vi>)
                        n572 = Open VI Reference(type specifier VI Refnum (for type only)=refnum<vi> refnum ("application reference (local)"), vi path=path "D:/Users/manip-thz/Documents/Controle_Manip_2020/subVIs/Scans/FineContrast.vi", options=256) -> (vi reference=w735:refnum<vi>, error out=w734:errorcluster)  [unwired: 3 in]
                        n573 = call-by-ref "Start Asynchronous Call"(reference=w735, error in=w734, "LightField Automation"=w727, "PZC200 Instrument Channel"=w715, "PZC Error"=w726, "Acq Time (ms) 2"=w709, "Acq Mode"=w707, "CCD ROI"=w708, "LightField Automation error"=w725, "Shutter Device Reference"=w717, "PZC Position Readout (usteps) 2"=w724, "LinTFine Start"=w714, "LinTFine End"=w713, "Shutter Controls"=w718, "Scan Spectrum Progess Bar 2"=w723, "Stop Contrast 2"=w719, "Pause Contrast 2"=w722, "Contrast 1D Spectrum 2"=w720, "LinTFine Step"=w712, "Accumulations"=w716, "Contrast Oscillations 2"=w721) -> ()  [unwired: 3 in, 8 out]
                        n574 = call-by-ref "Wait On Asynchronous Call"(reference=w735, error in=w734) -> (reference out=w729:refnum<vi>, error out=w728:errorcluster, "LightField Automation out"=w730:refnum<class "LightField Automation.lvclass">, "PZC200 Instrument Channel 2"=w733:string, "PZC Error 2"=w732:errorcluster, "PZA Positions"=w710:i32[], "Spectra vs PZA"=w711:i32[][], "LightField Automation error  out"=w731:errorcluster)  [unwired: 22 in]
                        n575 = Close Reference(reference=w729, error in (no error)=w728) -> ()  [unwired: 1 out]
                        n576 = local write "PZC200 Instrument Channel"(w733) -> ()
                        n577 = local write "PZC Error"(w732) -> ()
                        n578 = local write "Contrast Array Out"(w711) -> ()
                        n579 = local write "PZA12 Positions"(w710) -> ()
                      }
                      frame #2 {
                        w741 = FALSE ("Acq Cont")
                        w743 = TRUE
                        w746 = FALSE
                        n580 = property on="Stop Contrast" class="Bool (strict)"("Visible"=w746) -> ()  [unwired: 2 in, 2 out]
                        n581 = property on="Pause Contrast" class="Bool (strict)"("Visible"=w746) -> ()  [unwired: 2 in, 2 out]
                        n582 = local read "Scan LinTFine Params"() -> (w744:refnum<vi>[])
                        n583 = property on="Save Contrast" class="Bool (strict)"("Visible"=w743) -> ()  [unwired: 2 in, 2 out]
                        n584 = property on="Acquire Contrast" class="Bool (strict)"("Visible"=w743) -> ()  [unwired: 2 in, 2 out]
                        n585 = call "Enable&Disable_Controls.vi"("Enum"=enum16{"Enabled", "Disabled", "Disabled&Grayed"}."Enabled", "References"=w744) -> ()  [unwired: 1 in]
                        n586 = local write "Acquire Contrast"(FALSE ("Acq Cont")) -> ()
                        n587 = local write "Pause Contrast"(w741) -> ()
                        n588 = local write "Stop Contrast"(w741) -> ()
                        n589 = property on="Scan Linear Stage Progess Bar" class="Slide (strict)"("Visible"=TRUE, "Value"=u8 0 ("Scan Linear Stage Progess Bar")) -> ()  [unwired: 2 in, 2 out]
                      }
                    }
                  }
                  frame "Acquire Continuous Spectrum" {
                    n590 = stacked-sequence {
                      seq-local: [w754 _ _] -> [_ w760 _]
                      seq-local: [w753 _ _] -> [_ w759 _]
                      tunnel: w750 -> [w754 _ _]
                      tunnel: w749 -> [w753 _ _]
                      tunnel: [_ w758 _] -> w748
                      tunnel: [_ w757 _] -> w747
                      frame #0 {
                        # "open shutter once"
                        n591 = control-ref of="Shutter Ctrls"() -> (w752:refnum<vi>)
                        n592 = control-ref of="KCube Shutter Device Reference"() -> (w751:refnum<vi>)
                        n593 = call "Shutter.vi"("KCube Shutter Device Reference 2"=w751, "Shutter Ctrls 2"=w752) -> ()
                      }
                      frame #1 {
                        # "acquire 1000 spectra"
                        n594 = control-ref of="Stop continuous"() -> (w755:refnum<vi>)
                        n595 = for {
                          N: 1000 -> [_]
                          tunnel: w760 -> [w770]
                          tunnel: w759 -> [w769]
                          tunnel: [w768] -> w758
                          tunnel: [w767] -> w757
                          tunnel: w755 -> [w761]
                          stop <- w762 stop-if-true
                          n596 = local read "Accumulations"() -> (w766:dbl)
                          n597 = local read "Acq Mode"() -> (w765:T1)
                          n598 = call "LFA_Capture.vi"("error in (no error)"=w769, "Frames"=w766, "LightField Automation in"=w770) -> ("error out"=w767:errorcluster, "Data"=w764:T3, "LightField Automation out"=w768:refnum<class "LightField Automation.lvclass">)  [unwired: 6 in]
                          n599 = case shown="\"Image\"" w765 {
                            selector: w765 -> [w773 w778]
                            tunnel: w764 -> [w775 w780]
                            frame "Spectrum", Default {
                              n600 = local read "Wavelength calibration"() -> (w774:dbl[])
                              n601 = call "PrepareData4Graph.vi"("Wavelength nm"=w774, "DataLF"=w775, "AcqMode"=w773, "Data type"=T9."Spectre") -> ("Spectrum"=w772:cluster{"Array 2":dbl[], "Array":dbl[]})  [unwired: 2 in, 3 out]
                              n602 = local write "CCD 1D Spectrum Main"(w772) -> ()
                            }
                            frame "Image" {
                              n603 = local read "Wavelength calibration"() -> (w779:dbl[])
                              n604 = call "PrepareData4Graph.vi"("Wavelength nm"=w779, "DataLF"=w780, "AcqMode"=w778, "Data type"=T9."Spectre") -> ("Intensity Graph"=w777:dbl[][])  [unwired: 2 in, 3 out]
                              n605 = local write "CCD 2D Image Main"(w777) -> ()
                            }
                          }
                          n606 = property class="Bool (strict)"(reference=w761) -> ("Value"=w762:bool)  [unwired: 1 in, 2 out]
                          n607 = Wait (ms)(milliseconds to wait=u32 50) -> ()  [unwired: 1 out]
                        }
                      }
                      frame #2 {
                        # "close shutter"
                        n608 = control-ref of="Shutter Ctrls"() -> (w782:refnum<vi>)
                        n609 = control-ref of="KCube Shutter Device Reference"() -> (w781:refnum<vi>)
                        n610 = call "Shutter.vi"("KCube Shutter Device Reference 2"=w781, "Shutter Ctrls 2"=w782) -> ()
                      }
                    }
                  }
                  frame "Acquire Polarisation" {
                    n611 = stacked-sequence {
                      tunnel: w786 -> [_ w835 _]
                      tunnel: w785 -> [_ w832 _]
                      tunnel: [_ w834 _] -> w784
                      tunnel: [_ w833 _] -> w783
                      frame #0 {
                        w788 = TRUE ("Visible")
                        w790 = TRUE ("Visible")
                        # "shift scale to center"
                        # "from HWP to polarisation units"
                        # "Initialise measurement graphs and controls"
                        n612 = property on="CCD 1D Spectrum Main" class="XYGraph (strict)"() -> ("XScale.Maximum"=w794:dbl, "XScale.Minimum"=w793:dbl, "YScale.Minimum"=w792:dbl, "YScale.Maximum"=w791:dbl)  [unwired: 2 in, 2 out]
                        n613 = property on="StopPolar" class="Bool (strict)"("Visible"=w788) -> ()  [unwired: 2 in, 2 out]
                        n614 = property on="PausePolar" class="Bool (strict)"("Visible"=w788) -> ()  [unwired: 2 in, 2 out]
                        n615 = property on="Acquire Polarisation" class="Bool (strict)"("Value"=w790) -> ()  [unwired: 2 in, 2 out]
                        n616 = local read "Polar Start Angle (°)"() -> (w804:dbl)
                        n617 = local read "Scan Polar Params"() -> (w802:refnum<vi>[])
                        n618 = local read "Polar Step Angle (°)"() -> (w799:dbl)
                        n619 = local read "Polar Step Angle (°)"() -> (w796:dbl)
                        n620 = call "Enable&Disable_Controls.vi"("Enum"=enum16{"Enabled", "Disabled", "Disabled&Grayed"}."Disabled&Grayed", "References"=w802) -> ()  [unwired: 1 in]
                        n621 = property on="Polarisation 1D Spectrum" class="XYGraph (strict)"("XScale.Maximum"=w794, "XScale.Minimum"=w793, "YScale.Minimum"=w792, "YScale.Maximum"=w791) -> ()  [unwired: 2 in, 2 out]
                        n622 = Multiply(x=2.0, y=w804) -> (x*y=w797:dbl)
                        n623 = property on="Scan Polarisation Progess Bar" class="Slide (strict)"("Visible"=w790, "Value"=u8 0 ("Scan Polarisation Progess Bar")) -> ()  [unwired: 2 in, 2 out]
                        n624 = Subtract(x=w797, y=w796) -> (x-y=w795:dbl)
                        n625 = Multiply(x=2.0, y=w799) -> (x*y=w798:dbl)
                        n626 = property on="Polarisation 2D Image" class="IntGraph (strict)"("XScale.Multiplier"=w798, "XScale.Offset"=w795) -> ()  [unwired: 2 in, 2 out]
                        n627 = property on="Acquire Polarisation" class="Bool (strict)"("Visible"=FALSE) -> ()  [unwired: 2 in, 2 out]
                        n628 = property on="Experiment Graph Controls" class="TabCtl (strict)"("Value"=T2."Polarisation Acquisition" ("Experiment Graph Controls")) -> ()  [unwired: 2 in, 2 out]
                      }
                      frame #1 {
                        # "acquire polarisation"
                        n629 = control-ref of="KCube Shutter Device Reference"() -> (w808:refnum<vi>)
                        n630 = control-ref of="StopPolar"() -> (w826:refnum<vi>)
                        n631 = control-ref of="PausePolar"() -> (w827:refnum<vi>)
                        n632 = control-ref of="Polarisation 2D Image"() -> (w816:refnum<vi>)
                        n633 = local read "Polar mode"() -> (w812:u16)
                        n634 = case shown="3" w812 {
                          tunnel: [w836 w837] -> w811
                          frame 3 {
                            n635 = control-ref of="RotStage Exc Angle (°)"() -> ()  [unwired: 1 out]
                            n636 = control-ref of="RotStage Exc Angle Readout (°)"() -> (w836:refnum<vi>)
                          }
                          frame 2, Default {
                            n637 = control-ref of="RotStage Det Angle (°)"() -> ()  [unwired: 1 out]
                            n638 = control-ref of="RotStage Det Angle Readout (°)"() -> (w837:refnum<vi>)
                          }
                        }
                        n639 = local read "Acq Mode"() -> (w820:T1)
                        n640 = local read "Polar End Angle (°)"() -> (w823:dbl)
                        n641 = control-ref of="Polarisation 1D Spectrum"() -> (w818:refnum<vi>)
                        n642 = local read "ESP 301 Error"() -> (w822:errorcluster)
                        n643 = local read "Polar Step Angle (°)"() -> (w821:dbl)
                        n644 = local read "Acq Time (ms)"() -> (w819:dbl)
                        n645 = local read "Polar Start Angle (°)"() -> (w824:dbl)
                        n646 = Open VI Reference(type specifier VI Refnum (for type only)=refnum<vi> refnum ("application reference (local)"), vi path=path "D:/Users/manip-thz/Documents/Controle_Manip_2020/subVIs/Scans/Polarisation.vi", options=256) -> (vi reference=w806:refnum<vi>, error out=w831:errorcluster)  [unwired: 3 in]
                        n647 = control-ref of="Shutter Ctrls"() -> (w807:refnum<vi>)
                        n648 = control-ref of="Scan Polarisation Progess Bar"() -> (w817:refnum<vi>)
                        n649 = local read "ESP 301 COM Port"() -> (w825:refnum<visa-resource-name>)
                        n650 = call-by-ref "Start Asynchronous Call"(reference=w806, error in=w831, "VISA resource name"=w825, "Start Angle (°)"=w824, "Shutter Ctrls 2"=w807, "Exposure time (ms)"=w819, "End Angle (°)"=w823, "ESP301 Error"=w822, "LightField Automation in"=w835, "RotStage Exc Angle Refnum"=w811, "KCube Shutter Device Reference 2"=w808, "StopPolar 2"=w826, "CCD 1D Spectrum Main 3"=w818, "LightField error"=w832, "Acq Mode"=w820, "Bool Refnum"=w827, "Step Angle (°)"=w821, "Axis ESP301 / RotStage"=w812, "IntGraph Refnum"=w816, "Slide Refnum"=w817) -> ()  [unwired: 3 in, 9 out]
                        n651 = call-by-ref "Wait On Asynchronous Call"(reference=w806, error in=w831) -> (reference out=w810:refnum<vi>, error out=w809:errorcluster, "Angles"=w815:dbl[], "VISA resource name out"=w814:refnum<visa-resource-name>, "LightField Automation out"=w834:refnum<class "LightField Automation.lvclass">, "LightField error out"=w833:errorcluster, "ESP301 Error out"=w813:errorcluster)  [unwired: 21 in, 2 out]
                        n652 = Close Reference(reference=w810, error in (no error)=w809) -> ()  [unwired: 1 out]
                        n653 = local write "ESP 301 COM Port"(w814) -> ()
                        n654 = local write "Angles"(w815) -> ()
                        n655 = local write "ESP 301 Error"(w813) -> ()
                      }
                      frame #2 {
                        w839 = FALSE ("Visible")
                        # "set markers to polarisation values"
                        # "Reset measurement controls"
                        n656 = local read "Angles"() -> (w842:dbl[])
                        n657 = property on="Scan Polarisation Progess Bar" class="Slide (strict)"("Visible"=w839) -> ()  [unwired: 2 in, 2 out]
                        n658 = property on="PausePolar" class="Bool (strict)"("Visible"=w839) -> ()  [unwired: 2 in, 2 out]
                        n659 = property on="StopPolar" class="Bool (strict)"("Visible"=w839) -> ()  [unwired: 2 in, 2 out]
                        n660 = property on="Acquire Polarisation" class="Bool (strict)"("Visible"=TRUE ("Acquire Polarisation"), "Value"=FALSE ("Acquire Polarisation")) -> ()  [unwired: 2 in, 2 out]
                        n661 = local read "Scan Polar Params"() -> (w845:refnum<vi>[])
                        n662 = Multiply(x=2.0, y=w842) -> (x*y=w841:dbl[])
                        n663 = property on="Polarisation 2D Image" class="IntGraph (strict)"("XScale.MarkerVals[]"=w841) -> ()  [unwired: 2 in, 2 out]
                        n664 = call "Enable&Disable_Controls.vi"("Enum"=enum16{"Enabled", "Disabled", "Disabled&Grayed"}."Enabled", "References"=w845) -> ()  [unwired: 1 in]
                      }
                    }
                  }
                  frame "Acquire XY Map" {
                    n665 = disable-structure shown="Disabled" {
                      frame Disabled {
                        n666 = stacked-sequence {
                          frame #0 {
                            n667 = local read "Scan XY Map Params"() -> (w850:refnum<vi>[])
                            n668 = call "Enable&Disable_Controls.vi"("Enum"=enum16{"Enabled", "Disabled", "Disabled&Grayed"}."Disabled&Grayed", "References"=w850) -> ()  [unwired: 1 in]
                            n669 = property on="Experiment Graph Controls" class="TabCtl (strict)"("Value"=T11."XY Intensity Map Acquisition" ("Experiment Graph Controls")) -> ()  [unwired: 2 in, 2 out]
                          }
                          frame #1 {
                            n670 = control-ref of="CCD 1D Spectrum XY Map"() -> (w857:refnum<vi>)
                            n671 = control-ref of="Scan XY Map Progess Bar"() -> (w853:refnum<vi>)
                            n672 = control-ref of="CCD 2D Image XY Map"() -> (w856:refnum<vi>)
                            n673 = control-ref of="Scan X Readout (V)"() -> (w855:refnum<vi>)
                            n674 = control-ref of="Scan Y Readout (V)"() -> (w854:refnum<vi>)
                            n675 = local read "Scan X Tot. Length (V)"() -> (w862:dbl)
                            n676 = control-ref of="Stop XY Map"() -> (w858:refnum<vi>)
                            n677 = local read "Scan X Center (V)"() -> (w864:dbl)
                            n678 = local read "Scan X Res. (V)"() -> (w863:dbl)
                            n679 = local read "Scanning Mode"() -> (w865:T7)
                            n680 = local read "Scan Fast Axis"() -> (w851:enum16{"Y", "X"})
                            n681 = Build Array(w858, w857, w856, w853, w855, w854) -> (w852:refnum<vi>[])
                            n682 = local read "Scan Y Tot. Length"() -> (w860:dbl)
                            n683 = local read "Scan Y Center (V)"() -> (w861:dbl)
                            n684 = local read "Scan Y Res. (V)"() -> (w859:dbl)
                            n685 = call "SubVI_SCAN_FSM300.vi"("X center (Volt)"=w864, "Total Length X (Volt)"=w862, "Scan mode"=w865, "appended array"=w852, "Y center (Volt)"=w861, "Total Length Y (Volt)"=w860, "Resolution X (Volt)"=w863, "Resolution Y (Volt)"=w859, "''fast mooving'' axis"=w851) -> ()  [unwired: 11 in]
                          }
                        }
                      }
                      frame Enabled {
                      }
                    }
                  }
                }
                n686 = local write "LightField Automation error out"(w534) -> ()
                n687 = local write "LightField Automation out"(w536) -> ()
              }
              frame #1 {
                # "AutoSave?"
                n688 = property class="Bool (strict)"(reference=w867) -> ("Label.Text"=w866:string)  [unwired: 1 in, 2 out]
                n689 = local read "Auto< ?"() -> (w868:bool)
                n690 = case shown="True" w868 {
                  tunnel: w866 -> [_ w869]
                  frame False {
                  }
                  frame True {
                    n691 = case shown="\"Acq Cont\"" w869 {
                      frame "Acquire Continuous Spectrum" {
                      }
                      frame "Acquire Polarisation" {
                        n692 = property on="Save Polarisation" class="Bool (strict)"("Val(Sgnl)"=TRUE ("Value (Signaling)")) -> ()  [unwired: 2 in, 2 out]
                      }
                      frame "Acquire XY Map" {
                        n693 = property on="Save XY Map" class="Bool (strict)"("Val(Sgnl)"=TRUE ("Value (Signaling)")) -> ()  [unwired: 2 in, 2 out]
                      }
                      frame "Acq Cont" {
                        n694 = property on="Save Contrast" class="Bool (strict)"("Val(Sgnl)"=TRUE ("Value (Signaling)")) -> ()  [unwired: 2 in, 2 out]
                      }
                      frame "Acquire Spectrum", Default {
                        n695 = property on="Save Spectrum" class="Bool (strict)"("Val(Sgnl)"=TRUE ("Value (Signaling)")) -> ()  [unwired: 2 in, 2 out]
                      }
                    }
                  }
                }
              }
            }
          }
          event "StopPolar": Mouse Down {
            n696 = event-data() -> ("CtlRef"=w875:refnum<vi>)  [unwired: 1 in, 7 out]
            n697 = property class="Bool (strict)"(reference=w875) -> ("Label.Text"=w874:string)  [unwired: 1 in, 2 out]
            n698 = case shown="\"Stop Polar\"" w874 {
              frame "False" {
              }
              frame "Stop Polar" {
                n699 = local read "StopPolar"() -> (w876:bool)
                n700 = global write "Stops.vi" "StopPolar"(w876) -> ()
              }
              frame Default {
              }
            }
          }
          event "RotStage Exc Angle (°)", "RotStage Det Angle (°)", "Newport Linear Translation Stage Position (mm)", "Newport PZA12 Stage Position (usteps)": Value Change {
            n701 = event-data() -> ("CtlRef"=w879:refnum<vi>, "NewVal"=w878:dbl)  [unwired: 1 in, 4 out]
            n702 = property class="DigNum (strict)"(reference=w879) -> ("Label.Text"=w877:string)  [unwired: 1 in, 2 out]
            n703 = case shown="\"RotStage Det Angle (°)\"" w877 {
              tunnel: w877 -> [_ _ w903 w928 w953]
              tunnel: w878 -> [_ w881 w891 w916 w941]
              frame "False", Default {
              }
              frame "Newport PZA12 Stage Position (usteps)" {
                n704 = local read "PZC200 Instrument Channel"() -> (w885:string)
                n705 = call "PZCGetPos.vi"("Instrument Channel"=w885) -> ("Instrument Channel Out"=w882:string, "Position"=w884:i32)  [unwired: 1 in, 1 out]
                n706 = Not Equal?(x=w881, y=w884) -> (x != y?=w883:bool)
                n707 = case shown="True" w883 {
                  tunnel: w882 -> [w886 w890]
                  tunnel: w881 -> [_ w889]
                  tunnel: [w886 w888] -> w880
                  frame False {
                  }
                  frame True {
                    n708 = call "PZC_MoveAbs.vi"("Target"=w889, "Instrument"=w890) -> ("Final Position"=w887:i32, "Instrument out"=w888:string)  [unwired: 1 in, 1 out]
                    n709 = local write "PZC Position Readout (usteps)"(w887) -> ()
                  }
                }
                n710 = local write "PZC200 Instrument Channel"(w880) -> ()
              }
              frame "Newport Linear Translation Stage Position (mm)" {
                n711 = case shown="\"Newport Linear Translation Stage Position (mm)\"" w903 {
                  tunnel: [2 1 3] -> w904
                  tunnel: [w908 w911 w914] -> w900
                  tunnel: w891 -> [w907 w910 w913]
                  frame "RotStage Det Angle (°)" {
                    n712 = local write "RotStage Det Angle (°)"(w907) -> ()
                    n713 = control-ref of="RotStage Det Angle Readout (°)"() -> (w908:refnum<vi>)
                  }
                  frame "Newport Linear Translation Stage Position (mm)" {
                    n714 = local write "Newport Linear Translation Stage Position (mm)"(w910) -> ()
                    n715 = control-ref of="Newport Linear Translation Stage Position Readout (mm)"() -> (w911:refnum<vi>)
                  }
                  frame "RotStage Exc Angle (°)", Default {
                    n716 = local write "RotStage Exc Angle (°)"(w913) -> ()
                    n717 = control-ref of="RotStage Exc Angle Readout (°)"() -> (w914:refnum<vi>)
                  }
                }
                n718 = local read "Excitation Wavelength (nm)"() -> (w896:dbl)
                n719 = local read "Photodiode COM Port"() -> (w898:refnum<visa-resource-name>)
                n720 = local read "Photodiode error out"() -> (w897:errorcluster)
                n721 = local read "ESP 301 Error"() -> (w905:errorcluster)
                n722 = control-ref of="Excitation Power (uW)"() -> (w899:refnum<vi>)
                n723 = call <instrlib>:"TLPM Set Wavelength.vi"("error in (no error)"=w897, "Wavelength (0.0)"=w896, "instrument handle"=w898) -> ("error out"=w894:errorcluster, "instrument handle out"=w895:refnum<visa-resource-name>)  [unwired: 7 in]
                n724 = local read "ESP 301 COM Port"() -> (w906:refnum<visa-resource-name>)
                n725 = call "Go2Angle.vi"("Excitation Power (uW) 2"=w899, "Position (units)"=w891, "Photodiode error"=w894, "Photodiode"=w895, "ESP301 Error"=w905, "Axis ESP301 / RotStage"=w904, "RotStage Det Angle Readout (°) 4"=w900, "VISA resource name"=w906) -> ("ESP301 Error out"=w901:errorcluster, "Photodiode"=w893:errorcluster, "VISA resource name out"=w902:refnum<visa-resource-name>, "Photodiode out"=w892:refnum<visa-resource-name>)
                n726 = local write "Photodiode COM Port"(w892) -> ()
                n727 = local write "ESP 301 COM Port"(w902) -> ()
                n728 = local write "Photodiode error out"(w893) -> ()
                n729 = local write "ESP 301 Error"(w901) -> ()
              }
              frame "RotStage Exc Angle (°)" {
                n730 = case shown="\"Newport Linear Translation Stage Position (mm)\"" w928 {
                  tunnel: [2 1 3] -> w929
                  tunnel: [w933 w936 w939] -> w925
                  tunnel: w916 -> [w932 w935 w938]
                  frame "RotStage Det Angle (°)" {
                    n731 = local write "RotStage Det Angle (°)"(w932) -> ()
                    n732 = control-ref of="RotStage Det Angle Readout (°)"() -> (w933:refnum<vi>)
                  }
                  frame "Newport Linear Translation Stage Position (mm)" {
                    n733 = local write "Newport Linear Translation Stage Position (mm)"(w935) -> ()
                    n734 = control-ref of="Newport Linear Translation Stage Position Readout (mm)"() -> (w936:refnum<vi>)
                  }
                  frame "RotStage Exc Angle (°)", Default {
                    n735 = local write "RotStage Exc Angle (°)"(w938) -> ()
                    n736 = control-ref of="RotStage Exc Angle Readout (°)"() -> (w939:refnum<vi>)
                  }
                }
                n737 = local read "Excitation Wavelength (nm)"() -> (w921:dbl)
                n738 = local read "Photodiode COM Port"() -> (w923:refnum<visa-resource-name>)
                n739 = local read "Photodiode error out"() -> (w922:errorcluster)
                n740 = local read "ESP 301 Error"() -> (w930:errorcluster)
                n741 = control-ref of="Excitation Power (uW)"() -> (w924:refnum<vi>)
                n742 = call <instrlib>:"TLPM Set Wavelength.vi"("error in (no error)"=w922, "Wavelength (0.0)"=w921, "instrument handle"=w923) -> ("error out"=w919:errorcluster, "instrument handle out"=w920:refnum<visa-resource-name>)  [unwired: 7 in]
                n743 = local read "ESP 301 COM Port"() -> (w931:refnum<visa-resource-name>)
                n744 = call "Go2Angle.vi"("Excitation Power (uW) 2"=w924, "Position (units)"=w916, "Photodiode error"=w919, "Photodiode"=w920, "ESP301 Error"=w930, "Axis ESP301 / RotStage"=w929, "RotStage Det Angle Readout (°) 4"=w925, "VISA resource name"=w931) -> ("ESP301 Error out"=w926:errorcluster, "Photodiode"=w918:errorcluster, "VISA resource name out"=w927:refnum<visa-resource-name>, "Photodiode out"=w917:refnum<visa-resource-name>)
                n745 = local write "Photodiode COM Port"(w917) -> ()
                n746 = local write "ESP 301 COM Port"(w927) -> ()
                n747 = local write "Photodiode error out"(w918) -> ()
                n748 = local write "ESP 301 Error"(w926) -> ()
              }
              frame "RotStage Det Angle (°)" {
                n749 = case shown="\"Newport Linear Translation Stage Position (mm)\"" w953 {
                  tunnel: [2 1 3] -> w954
                  tunnel: [w958 w961 w964] -> w950
                  tunnel: w941 -> [w957 w960 w963]
                  frame "RotStage Det Angle (°)" {
                    n750 = local write "RotStage Det Angle (°)"(w957) -> ()
                    n751 = control-ref of="RotStage Det Angle Readout (°)"() -> (w958:refnum<vi>)
                  }
                  frame "Newport Linear Translation Stage Position (mm)" {
                    n752 = local write "Newport Linear Translation Stage Position (mm)"(w960) -> ()
                    n753 = control-ref of="Newport Linear Translation Stage Position Readout (mm)"() -> (w961:refnum<vi>)
                  }
                  frame "RotStage Exc Angle (°)", Default {
                    n754 = local write "RotStage Exc Angle (°)"(w963) -> ()
                    n755 = control-ref of="RotStage Exc Angle Readout (°)"() -> (w964:refnum<vi>)
                  }
                }
                n756 = local read "Excitation Wavelength (nm)"() -> (w946:dbl)
                n757 = local read "Photodiode COM Port"() -> (w948:refnum<visa-resource-name>)
                n758 = local read "Photodiode error out"() -> (w947:errorcluster)
                n759 = local read "ESP 301 Error"() -> (w955:errorcluster)
                n760 = control-ref of="Excitation Power (uW)"() -> (w949:refnum<vi>)
                n761 = call <instrlib>:"TLPM Set Wavelength.vi"("error in (no error)"=w947, "Wavelength (0.0)"=w946, "instrument handle"=w948) -> ("error out"=w944:errorcluster, "instrument handle out"=w945:refnum<visa-resource-name>)  [unwired: 7 in]
                n762 = local read "ESP 301 COM Port"() -> (w956:refnum<visa-resource-name>)
                n763 = call "Go2Angle.vi"("Excitation Power (uW) 2"=w949, "Position (units)"=w941, "Photodiode error"=w944, "Photodiode"=w945, "ESP301 Error"=w955, "Axis ESP301 / RotStage"=w954, "RotStage Det Angle Readout (°) 4"=w950, "VISA resource name"=w956) -> ("ESP301 Error out"=w951:errorcluster, "Photodiode"=w943:errorcluster, "VISA resource name out"=w952:refnum<visa-resource-name>, "Photodiode out"=w942:refnum<visa-resource-name>)
                n764 = local write "Photodiode COM Port"(w942) -> ()
                n765 = local write "ESP 301 COM Port"(w952) -> ()
                n766 = local write "Photodiode error out"(w943) -> ()
                n767 = local write "ESP 301 Error"(w951) -> ()
              }
            }
          }
          event "PZC Position Readout (usteps)": Mouse Down {
            n768 = event-data() -> ()  [unwired: 1 in, 8 out]
            n769 = local read "PZC200 Instrument Channel"() -> (w969:string)
            n770 = call "PZCGetPos.vi"("Instrument Channel"=w969) -> ("Instrument Channel Out"=w966:string, "Position"=w968:i32, "error out"=w967:errorcluster)  [unwired: 1 in]
            n771 = local write "PZC Error"(w967) -> ()
            n772 = local write "PZC200 Instrument Channel"(w966) -> ()
            n773 = local write "PZC Position Readout (usteps)"(w968) -> ()
          }
          event "RotStage Exc Home", "RotStage Det Home", "Newport Linear Translation Stage Home": Mouse Down {
            n774 = event-data() -> ("CtlRef"=w972:refnum<vi>)  [unwired: 1 in, 7 out]
            n775 = property class="Bool (strict)"(reference=w972) -> ("Label.Text"=w971:string)  [unwired: 1 in, 2 out]
            n776 = case shown="\"Newport Linear Translation Stage Home\"" w971 {
              tunnel: 0.0 -> [w973 w974 w975]
              frame "RotStage Det Home", Default {
                n777 = property on="RotStage Det Angle (°)" class="DigNum (strict)"("Val(Sgnl)"=w973) -> ()  [unwired: 2 in, 2 out]
              }
              frame "Newport Linear Translation Stage Home" {
                n778 = property on="Newport Linear Translation Stage Position (mm)" class="DigNum (strict)"("Val(Sgnl)"=w974) -> ()  [unwired: 2 in, 2 out]
              }
              frame "RotStage Exc Home" {
                n779 = property on="RotStage Exc Angle (°)" class="DigNum (strict)"("Val(Sgnl)"=w975) -> ()  [unwired: 2 in, 2 out]
              }
            }
          }
          event "RotStage Exc Jog Backward", "RotStage Det Jog Backward", "RotStage Exc Jog Forward", "RotStage Det Jog Forward", "Newport Linear Translation Stage Jog Forward", "Newport Linear Translation Stage Jog Backward", "PZC Jog Forward", "PZC Jog Backward": Mouse Down {
            n780 = event-data() -> ("CtlRef"=w978:refnum<vi>)  [unwired: 1 in, 7 out]
            n781 = property class="Bool (strict)"(reference=w978) -> ("Label.Text"=w977:string, "Value"=w976:bool)  [unwired: 1 in, 2 out]
            n782 = case shown="\"PZC Jog Forward\"" w977 {
              tunnel: w976 -> [_ _ _ _ _ _ _ _ _]
              frame "RotStage Det Jog Backward" {
                n783 = local read "RotStage Det Angle Readout (°)"() -> (w981:dbl)
                n784 = local read "RotStage Det Angle Step (°)"() -> (w980:dbl)
                n785 = Subtract(x=w981, y=w980) -> (x-y=w979:dbl)
                n786 = property on="RotStage Det Angle (°)" class="DigNum (strict)"("Val(Sgnl)"=w979) -> ()  [unwired: 2 in, 2 out]
              }
              frame "RotStage Det Jog Forward" {
                n787 = local read "RotStage Det Angle Readout (°)"() -> (w983:dbl)
                n788 = local read "RotStage Det Angle Step (°)"() -> (w984:dbl)
                n789 = Add(x=w983, y=w984) -> (x+y=w982:dbl)
                n790 = property on="RotStage Det Angle (°)" class="DigNum (strict)"("Val(Sgnl)"=w982) -> ()  [unwired: 2 in, 2 out]
              }
              frame "RotStage Exc Jog Forward" {
                n791 = local read "RotStage Exc Angle Readout (°)"() -> (w987:dbl)
                n792 = local read "RotStage Exc Angle Step (°)"() -> (w986:dbl)
                n793 = Add(x=w987, y=w986) -> (x+y=w985:dbl)
                n794 = property on="RotStage Exc Angle (°)" class="DigNum (strict)"("Val(Sgnl)"=w985) -> ()  [unwired: 2 in, 2 out]
              }
              frame "Newport Linear Translation Stage Jog Forward" {
                n795 = local read "Newport Linear Translation Stage Position Readout (mm)"() -> (w992:dbl)
                n796 = local read "Newport Linear Translation Stage Step (mm)"() -> (w991:dbl)
                n797 = Add(x=w992, y=w991) -> (x+y=w990:dbl)
                n798 = local read "Right Limit (mm)"() -> (w989:dbl)
                n799 = Less Or Equal?(x=w990, y=w989) -> (x <= y?=w988:bool)
                n800 = case shown="False" w988 {
                  tunnel: w990 -> [_ w996]
                  frame False {
                    n801 = stacked-sequence {
                      frame #0 {
                        n802 = property on="Newport Linear Translation Stage Position Readout (mm)" class="DigNum (strict)"("Blinking"=TRUE) -> ()  [unwired: 2 in, 2 out]
                      }
                      frame #1 {
                        n803 = Wait (ms)(milliseconds to wait=u32 500) -> ()  [unwired: 1 out]
                      }
                      frame #2 {
                        n804 = property on="Newport Linear Translation Stage Position Readout (mm)" class="DigNum (strict)"("Blinking"=FALSE) -> ()  [unwired: 2 in, 2 out]
                      }
                    }
                  }
                  frame True {
                    n805 = property on="Newport Linear Translation Stage Position (mm)" class="DigNum (strict)"("Val(Sgnl)"=w996) -> ()  [unwired: 2 in, 2 out]
                  }
                }
              }
              frame "Newport Linear Translation Stage Jog Backward" {
                n806 = local read "Newport Linear Translation Stage Position Readout (mm)"() -> (w1001:dbl)
                n807 = local read "Newport Linear Translation Stage Step (mm)"() -> (w1000:dbl)
                n808 = local read "Left Limit (mm)"() -> (w999:dbl)
                n809 = Subtract(x=w1001, y=w1000) -> (x-y=w997:dbl)
                n810 = Greater Or Equal?(x=w997, y=w999) -> (x >= y?=w998:bool)
                n811 = case shown="False" w998 {
                  tunnel: w997 -> [_ w1005]
                  frame False {
                    n812 = stacked-sequence {
                      frame #0 {
                        n813 = property on="Newport Linear Translation Stage Position Readout (mm)" class="DigNum (strict)"("Blinking"=TRUE) -> ()  [unwired: 2 in, 2 out]
                      }
                      frame #1 {
                        n814 = Wait (ms)(milliseconds to wait=u32 500) -> ()  [unwired: 1 out]
                      }
                      frame #2 {
                        n815 = property on="Newport Linear Translation Stage Position Readout (mm)" class="DigNum (strict)"("Blinking"=FALSE) -> ()  [unwired: 2 in, 2 out]
                      }
                    }
                  }
                  frame True {
                    n816 = property on="Newport Linear Translation Stage Position (mm)" class="DigNum (strict)"("Val(Sgnl)"=w1005) -> ()  [unwired: 2 in, 2 out]
                  }
                }
              }
              frame "RotStage Exc Jog Backward" {
                n817 = local read "RotStage Exc Angle Readout (°)"() -> (w1008:dbl)
                n818 = local read "RotStage Exc Angle Step (°)"() -> (w1007:dbl)
                n819 = Subtract(x=w1008, y=w1007) -> (x-y=w1006:dbl)
                n820 = property on="RotStage Exc Angle (°)" class="DigNum (strict)"("Val(Sgnl)"=w1006) -> ()  [unwired: 2 in, 2 out]
              }
              frame "PZC Jog Forward" {
                n821 = local read "PZC Speed (usteps/s)"() -> (w1014:u16)
                n822 = local read "PZC200 Instrument Channel"() -> (w1023:string)
                n823 = Number To Decimal String(number=w1014) -> (decimal integer string=w1016:string)  [unwired: 1 in]
                n824 = Concatenate Strings("1JA" ("Command"), w1016) -> (w1022:string)
                n825 = call "SendCommand.vi"("Command"=w1022, "Instrument Channel"=w1023) -> ("error out"=w1020:errorcluster, "Instrument Channel out"=w1021:string)  [unwired: 8 in]
                n826 = call "ReadCommand.vi"("Disable MAV check (F)"=FALSE, "error in"=w1020, "Instrument Channel"=w1021) -> ("error out"=w1017:errorcluster, "Instrument Channel out"=w1019:string)  [unwired: 6 in, 1 out]
                n827 = while {
                  shift-right: [w1027] -> w1013
                  shift-left: w1019 -> [w1031]
                  shift-right: [w1025] -> w1012
                  shift-left: w1017 -> [w1026]
                  tunnel: ["1ST"] -> w1011
                  stop <- w1028 continue-if-true
                  n828 = call "PZCGetPos.vi"("error in"=w1026, "Instrument Channel"=w1031) -> ("Instrument Channel Out"=w1027:string, "Position"=w1030:i32, "error out"=w1025:errorcluster)
                  n829 = local write "PZC Position Readout (usteps)"(w1030) -> ()
                  n830 = Wait (ms)(milliseconds to wait=u32 150) -> ()  [unwired: 1 out]
                  n831 = local read "PZC Jog Forward"() -> (w1028:bool)
                }
                n832 = call "SendCommand.vi"("error in"=w1012, "Command"=w1011, "Instrument Channel"=w1013) -> ("error out"=w1009:errorcluster, "Instrument Channel out"=w1010:string)  [unwired: 7 in]
                n833 = local write "PZC200 Instrument Channel"(w1010) -> ()
                n834 = local write "PZC Error"(w1009) -> ()
              }
              frame Default {
              }
              frame "PZC Jog Backward" {
                n835 = local read "PZC Speed (usteps/s)"() -> (w1032:u16)
                n836 = local read "PZC200 Instrument Channel"() -> (w1046:string)
                n837 = Number To Decimal String(number=w1032) -> (decimal integer string=w1034:string)  [unwired: 1 in]
                n838 = Concatenate Strings("1JA-" ("Command"), w1034) -> (w1045:string)
                n839 = call "SendCommand.vi"("Command"=w1045, "Instrument Channel"=w1046) -> ("error out"=w1043:errorcluster, "Instrument Channel out"=w1044:string)  [unwired: 8 in]
                n840 = call "ReadCommand.vi"("Disable MAV check (F)"=FALSE, "error in"=w1043, "Instrument Channel"=w1044) -> ("error out"=w1040:errorcluster, "Instrument Channel out"=w1041:string)  [unwired: 6 in, 1 out]
                n841 = while {
                  shift-right: [w1048] -> w1039
                  shift-left: w1040 -> [w1049]
                  shift-right: [w1050] -> w1038
                  shift-left: w1041 -> [w1054]
                  tunnel: ["1ST"] -> w1037
                  stop <- w1052 continue-if-true
                  n842 = call "PZCGetPos.vi"("error in"=w1049, "Instrument Channel"=w1054) -> ("Instrument Channel Out"=w1050:string, "Position"=w1053:i32, "error out"=w1048:errorcluster)
                  n843 = local write "PZC Position Readout (usteps)"(w1053) -> ()
                  n844 = Wait (ms)(milliseconds to wait=u32 150) -> ()  [unwired: 1 out]
                  n845 = local read "PZC Jog Backward"() -> (w1052:bool)
                }
                n846 = call "SendCommand.vi"("error in"=w1039, "Command"=w1037, "Instrument Channel"=w1038) -> ("error out"=w1035:errorcluster, "Instrument Channel out"=w1036:string)  [unwired: 7 in]
                n847 = local write "PZC200 Instrument Channel"(w1036) -> ()
                n848 = local write "PZC Error"(w1035) -> ()
              }
            }
          }
          event "RotStage Exc Velocity (°/s)", "RotStage Det Velocity (°/s)", "Newport Linear Translation Stage Velocity (mm/s)": Value Change {
            n849 = event-data() -> ("CtlRef"=w1061:refnum<vi>, "NewVal"=w1059:dbl)  [unwired: 1 in, 4 out]
            n850 = property class="DigNum (strict)"(reference=w1061) -> ("Label.Text"=w1060:string)  [unwired: 1 in, 2 out]
            n851 = local read "ESP 301 COM Port"() -> (w1058:refnum<visa-resource-name>)
            n852 = local read "ESP 301 Error"() -> (w1057:errorcluster)
            n853 = case shown="\"RotStage Det Velocity (°/s)\"" w1060 {
              tunnel: w1059 -> [w1065 _ w1070 w1080]
              tunnel: w1058 -> [w1066 w1069 w1072 w1079]
              tunnel: w1057 -> [w1067 w1068 w1073 w1078]
              tunnel: [w1063 w1069 w1075 w1077] -> w1056
              tunnel: [w1062 w1068 w1074 w1076] -> w1055
              frame "Newport Linear Translation Stage Velocity (mm/s)" {
                n854 = call "Set Velocity.vi"("error in (no error)"=w1067, "Velocity (units/s)"=w1065, "Axis (1)"=1, "VISA resource name"=w1066) -> ("error out"=w1062:errorcluster, "VISA resource name out"=w1063:refnum<visa-resource-name>)  [unwired: 2 in]
              }
              frame Default {
              }
              frame "RotStage Det Velocity (°/s)" {
                n855 = call "Set Velocity.vi"("error in (no error)"=w1073, "Velocity (units/s)"=w1070, "Axis (1)"=2, "VISA resource name"=w1072) -> ("error out"=w1074:errorcluster, "VISA resource name out"=w1075:refnum<visa-resource-name>)  [unwired: 2 in]
              }
              frame "RotStage Exc Velocity (°/s)" {
                n856 = call "Set Velocity.vi"("error in (no error)"=w1078, "Velocity (units/s)"=w1080, "Axis (1)"=3, "VISA resource name"=w1079) -> ("error out"=w1076:errorcluster, "VISA resource name out"=w1077:refnum<visa-resource-name>)  [unwired: 2 in]
              }
            }
            n857 = local write "ESP 301 COM Port"(w1056) -> ()
            n858 = local write "ESP 301 Error"(w1055) -> ()
          }
          event "Exposure Time (ms)": Value Change {
            n859 = event-data() -> ("NewVal"=w1082:dbl)  [unwired: 1 in, 5 out]
            n860 = local read "LightField Automation error out"() -> (w1091:errorcluster)
            n861 = local read "LightField Automation out"() -> (w1090:refnum<class "LightField Automation.lvclass">)
            n862 = Divide(x=w1082, y=1000.0) -> (x/y=w1083:dbl)
            n863 = call "Exp_CCD_GetExposureTime.vi"("error in (no error)"=w1091, "LightField Automation in"=w1090) -> ("error out"=w1084:errorcluster, "Exposure Time (s)"=w1089:dbl, "LightField Automation out"=w1085:refnum<class "LightField Automation.lvclass">)  [unwired: 7 in]
            n864 = Equal?(x=w1089, y=w1083) -> (x = y?=w1088:bool)
            n865 = case shown="False" w1088 {
              tunnel: [w1098 w1114] -> w1087
              tunnel: [w1097 w1115] -> w1086
              tunnel: w1085 -> [w1095 w1115]
              tunnel: w1084 -> [w1094 w1114]
              tunnel: w1083 -> [w1096 _]
              tunnel: w1082 -> [w1093 _]
              frame False {
                n866 = stacked-sequence {
                  seq-local: [w1103 _] -> [_ w1113]
                  seq-local: [w1102 _] -> [_ w1112]
                  tunnel: w1096 -> [w1101 _]
                  tunnel: w1095 -> [w1100 _]
                  tunnel: w1094 -> [w1099 _]
                  tunnel: [_ w1113] -> w1098
                  tunnel: [_ w1112] -> w1097
                  tunnel: w1093 -> [_ w1109]
                  frame #0 {
                    n867 = call "Exp_CCD_SetExposureTime.vi"("error in (no error)"=w1099, "Exposure Time (s)"=w1101, "LightField Automation in"=w1100) -> ("error out"=w1103:errorcluster, "LightField Automation out"=w1102:refnum<class "LightField Automation.lvclass">)  [unwired: 7 in]
                  }
                  frame #1 {
                    n868 = Format Into String(format string="%5d", initial string="Exposure time set to ", w1109) -> (resulting string=w1105:string)  [unwired: 1 in, 1 out]
                    n869 = local read "Log file"() -> (w1111:string)
                    n870 = Concatenate Strings(w1105, " ms") -> (w1104:string)
                    n871 = call "Write2LogFile.vi"("Add to log file"=w1104, "Log file before"=w1111) -> ("Log file after"=w1110:string)
                    n872 = local write "Log file"(w1110) -> ()
                  }
                }
              }
              frame True {
              }
            }
            n873 = local write "Acq Time (ms)"(w1082) -> ()
            n874 = local write "LightField Automation out"(w1086) -> ()
            n875 = local write "LightField Automation error out"(w1087) -> ()
          }
          event "Acq Time (ms)": Value Change {
            n876 = event-data() -> ("NewVal"=w1116:dbl)  [unwired: 1 in, 5 out]
            n877 = local read "Acq Mode"() -> (w1117:T1)
            n878 = case shown="\"Image\"" w1117 {
              tunnel: w1116 -> [w1118 w1119]
              frame "Image" {
                n879 = property on="Exposure Time (ms)" class="DigNum (strict)"("Val(Sgnl)"=w1118) -> ()  [unwired: 2 in, 2 out]
              }
              frame "Spectrum", Default {
                n880 = property on="Exposure Time (ms)" class="DigNum (strict)"("Val(Sgnl)"=w1119) -> ()  [unwired: 2 in, 2 out]
              }
            }
          }
          event "CCD 1D Spectrum Main", "Contrast Oscillations", "Contrast 1D Spectrum": Cursor Release {
            n881 = event-data() -> ("CtlRef"=w1123:refnum<vi>, "CursRef"=w1121:refnum<vi>)  [unwired: 1 in, 7 out]
            n882 = property class="Curs"(reference=w1121) -> ("Cursor Name"=w1120:string)  [unwired: 1 in, 2 out]
            n883 = property class="XYGraph (strict)"(reference=w1123) -> ("Label.Text"=w1122:string)  [unwired: 1 in, 2 out]
            n884 = case shown="\"Contrast Oscillations\"" w1122 {
              tunnel: w1120 -> [w1124 _ _ _]
              frame "Contrast Oscillations" {
                n885 = case shown="\"ContPos\"" w1124 {
                  frame "False", Default {
                  }
                  frame "ContPos" {
                    n886 = local read "Cursor controls"() -> (w1125:bool)
                    n887 = case shown="True" w1125 {
                      frame False {
                      }
                      frame True {
                        n888 = property on="Contrast Oscillations" class="XYGraph (strict)"("Active Cursor"=u32 2) -> ("Cursor.Cursor X"=w1126:dbl)  [unwired: 2 in, 2 out]
                        n889 = Number To Decimal String(number=w1126) -> (decimal integer string=w1128:string)  [unwired: 1 in]
                        n890 = property on="Contrast 1D Spectrum from Cursors" class="XYGraph (strict)"("Caption.Text"=w1128) -> ()  [unwired: 2 in, 2 out]
                      }
                    }
                  }
                  frame "ContInt1" {
                    n891 = property on="Contrast Oscillations" class="XYGraph (strict)"("Active Cursor"=u32 0, "Active Cursor"=u32 1) -> ("Cursor.Cursor Y"=w1131:dbl, "Cursor.Cursor Y"=w1130:dbl)  [unwired: 2 in, 2 out]
                    n892 = call "Contrast.vi"("Y2"=w1130, "Y1"=w1131) -> ("(max(Y1,Y2) - min(Y1,Y2)) / (Y1 + Y2)"=w1129:dbl)
                    n893 = local write "Contrast"(w1129) -> ()
                  }
                  frame "ContInt2" {
                    n894 = property on="Contrast Oscillations" class="XYGraph (strict)"("Active Cursor"=u32 0, "Active Cursor"=u32 1) -> ("Cursor.Cursor Y"=w1136:dbl, "Cursor.Cursor Y"=w1135:dbl)  [unwired: 2 in, 2 out]
                    n895 = call "Contrast.vi"("Y2"=w1135, "Y1"=w1136) -> ("(max(Y1,Y2) - min(Y1,Y2)) / (Y1 + Y2)"=w1134:dbl)
                    n896 = local write "Contrast"(w1134) -> ()
                  }
                }
              }
              frame "Contrast 1D Spectrum" {
                n897 = case shown="True" "Cursor controls" {
                  frame False {
                  }
                  frame True {
                    n898 = property on="Contrast 1D Spectrum" class="XYGraph (strict)"("Active Cursor"=u32 0, "Active Cursor"=u32 1) -> ("Cursor.Cursor X"=w1147:dbl, "Cursor.Cursor X"=w1146:dbl)  [unwired: 2 in, 2 out]
                    n899 = local read "Wavelength calibration"() -> (w1152:dbl[])
                    n900 = local read "Contrast Array Out"() -> (w1148:dbl[][])
                    n901 = Divide(x=1239.841, y=w1152) -> (x/y=w1149:dbl[])
                    n902 = call "Cursors4Contrast_v2.vi"("Cursor 2"=w1146, "Cursor 1"=w1147, "Spectres vs PZA"=w1148, "Energy"=w1149) -> ("Contrast of ROI vs PZC"=w1145:dbl[], "Spectra ROI"=w1142:dbl[][], "Energy ROI"=w1144:dbl[])
                    n903 = Index Array(array=w1142, index (row)=0) -> (element=w1140:dbl[])  [unwired: 1 in]
                    n904 = local read "PZA12 Positions"() -> (w1151:dbl[])
                    n905 = Bundle("Energy ROI"=w1144, "Spectra ROI"=w1140) -> (w1143:cluster{"Energy ROI":dbl[], "Spectra ROI":dbl[]})  [unwired: 1 in]
                    n906 = property on="Contrast 1D Spectrum from Cursors" class="XYGraph (strict)"("Value"=w1143) -> ()  [unwired: 2 in, 2 out]
                    n907 = Bundle("PZA12 Positions"=w1151, "Contrast of ROI vs PZC"=w1145) -> (w1150:T14)  [unwired: 1 in]
                    n908 = property on="Contrast Oscillations" class="XYGraph (strict)"("Value"=w1150) -> ()  [unwired: 2 in, 2 out]
                  }
                }
              }
              frame Default {
              }
              frame "CCD 1D Spectrum Main" {
                n909 = stacked-sequence {
                  seq-local: [w1157 _] -> [_ w1165]
                  seq-local: [w1156 _] -> [_ w1164]
                  frame #0 {
                    n910 = property on="CCD 1D Spectrum Main" class="XYGraph (strict)"("Active Cursor"=u32 0, "Active Cursor"=u32 1) -> ("Cursor.Cursor X"=w1157:dbl, "Cursor.Cursor X"=w1156:dbl)  [unwired: 2 in, 2 out]
                    n911 = local write "CCD 1D Spectrum Main Cursor"(w1157) -> ()
                    n912 = local write "CCD 1D Spectrum Main Cursor 2"(w1156) -> ()
                  }
                  frame #1 {
                    n913 = call "Cursors2Freq.vi"("Cursor 1 eV"=w1165, "Cursor 2 eV"=w1164) -> ("Cursor dE"=w1163:dbl, "Cursor 1 nm"=w1162:dbl, "Cursor 2 nm"=w1161:dbl, "Cursor dnm"=w1160:dbl)
                    n914 = local write "CCD 1D Spectrum Main deltaE"(w1163) -> ()
                    n915 = local write "CCD 1D Spectrum Main Cursor 1 nm"(w1162) -> ()
                    n916 = local write "CCD 1D Spectrum Main Cursor 2 nm"(w1161) -> ()
                    n917 = Multiply(x=w1160, y=1e-09) -> (x*y=w1166:dbl)
                    n918 = local write "CCD 1D Spectrum Main deltanm"(w1166) -> ()
                  }
                }
              }
            }
          }
          event "Shutter Ctrls", "KCubeSolenoidControl": Mouse Down {
            n919 = event-data() -> ()  [unwired: 1 in, 8 out]
            n920 = control-ref of="Shutter Ctrls"() -> (w1169:refnum<vi>)
            n921 = control-ref of="KCube Shutter Device Reference"() -> (w1168:refnum<vi>)
            n922 = call "Shutter.vi"("KCube Shutter Device Reference 2"=w1168, "Shutter Ctrls 2"=w1169) -> ()
          }
          event "Reset origins": Value Change {
            n923 = event-data() -> ("NewVal"=w1170:bool)  [unwired: 1 in, 5 out]
            n924 = case shown="True" w1170 {
              frame False {
              }
              frame True {
                n925 = disable-structure shown="Disabled" {
                  frame Disabled {
                    n926 = local read "Newport Linear Translation Stage Position Readout (mm)"() -> ()  [unwired: 1 out]
                    n927 = local read "PZC Position Readout (usteps)"() -> ()  [unwired: 1 out]
                  }
                  frame Enabled {
                  }
                }
              }
            }
          }
          event "Motor LinT On?", "Motor RotStage Exc On?", "Motor RotStage Det On?", "LinTFine Motor On?": Mouse Down {
            n928 = event-data() -> ("CtlRef"=w1173:refnum<vi>)  [unwired: 1 in, 7 out]
            n929 = property class="Bool (strict)"(reference=w1173) -> ("Label.Text"=w1172:string, "Value"=w1171:bool)  [unwired: 1 in, 2 out]
            n930 = case shown="\"Motor LinT On?\"" w1172 {
              tunnel: w1171 -> [w1174 _ w1182 w1188 w1192]
              frame "Motor RotStage Exc On?" {
                n931 = local read "ESP 301 COM Port"() -> (w1179:refnum<visa-resource-name>)
                n932 = local read "ESP 301 Error"() -> (w1178:errorcluster)
                n933 = call "Enable Disable Motor.vi"("error in (no error)"=w1178, "Action (F - OFF)"=w1174, "Axis (1)"=2, "VISA resource name"=w1179) -> ("error out"=w1176:errorcluster, "VISA resource name out"=w1177:refnum<visa-resource-name>)  [unwired: 2 in]
                n934 = local write "ESP 301 COM Port"(w1177) -> ()
                n935 = local write "ESP 301 Error"(w1176) -> ()
              }
              frame Default {
                # "default do nothing"
              }
              frame "LinTFine Motor On?" {
                n936 = local read "PZC200 Instrument Channel"() -> (w1183:string)
                n937 = case shown="False" w1182 {
                  tunnel: ["1MF" "1MO" ("Command")] -> w1181
                  frame False {
                  }
                  frame True {
                  }
                }
                n938 = call "SendCommand.vi"("Command"=w1181, "Instrument Channel"=w1183) -> ("Instrument Channel out"=w1180:string)  [unwired: 8 in, 1 out]
                n939 = local write "PZC200 Instrument Channel"(w1180) -> ()
              }
              frame "Motor LinT On?" {
                n940 = local read "ESP 301 COM Port"() -> (w1191:refnum<visa-resource-name>)
                n941 = local read "ESP 301 Error"() -> (w1190:errorcluster)
                n942 = call "Enable Disable Motor.vi"("error in (no error)"=w1190, "Action (F - OFF)"=w1188, "Axis (1)"=1, "VISA resource name"=w1191) -> ("error out"=w1186:errorcluster, "VISA resource name out"=w1187:refnum<visa-resource-name>)  [unwired: 2 in]
                n943 = local write "ESP 301 COM Port"(w1187) -> ()
                n944 = local write "ESP 301 Error"(w1186) -> ()
              }
              frame "Motor RotStage Det On?" {
                n945 = local read "ESP 301 COM Port"() -> (w1197:refnum<visa-resource-name>)
                n946 = local read "ESP 301 Error"() -> (w1196:errorcluster)
                n947 = call "Enable Disable Motor.vi"("error in (no error)"=w1196, "Action (F - OFF)"=w1192, "Axis (1)"=3, "VISA resource name"=w1197) -> ("error out"=w1194:errorcluster, "VISA resource name out"=w1195:refnum<visa-resource-name>)  [unwired: 2 in]
                n948 = local write "ESP 301 COM Port"(w1195) -> ()
                n949 = local write "ESP 301 Error"(w1194) -> ()
              }
            }
          }
          event "TEC Output", "TEC Temperature", "Laser on? Control": Mouse Down; "Laser Diode Current Set": Value Change {
            n950 = event-data() -> ("CtlRef"=w1202:refnum<vi>)  [unwired: 1 in, 3 out]
            n951 = local read "Photodiode COM Port"() -> (w1201:refnum<visa-resource-name>)
            n952 = local read "Diode Driver COM"() -> (w1207:refnum<visa-resource-name>)
            n953 = local read "Diode Driver Error"() -> (w1206:errorcluster)
            n954 = local read "Photodiode error out"() -> (w1200:errorcluster)
            n955 = property class="Ctl"(reference=w1202) -> ("Label.Text"=w1203:string)  [unwired: 1 in, 2 out]
            n956 = case shown="\"TEC Temperature\"" w1203 {
              tunnel: w1207 -> [w1213 w1224 w1251 w1285]
              tunnel: w1206 -> [w1212 w1223 w1250 w1284]
              tunnel: [w1211 w1221 w1249 w1276] -> w1205
              tunnel: [w1210 w1222 w1248 w1279] -> w1204
              tunnel: w1201 -> [w1208 w1216 w1245 w1277]
              tunnel: w1200 -> [w1209 w1215 w1244 w1278]
              tunnel: [w1208 w1218 w1243 w1277] -> w1199
              tunnel: [w1209 w1217 w1242 w1278] -> w1198
              frame "TEC Temperature" {
                n957 = call <instrlib>:"TL4000 Measure Temperature.vi"("error in (no error)"=w1212, "instrument handle"=w1213) -> ("error out"=w1210:errorcluster, "Temperature"=w1214:dbl, "instrument handle out"=w1211:refnum<visa-resource-name>)  [unwired: 7 in]
                n958 = local write "TEC Temperature"(w1214) -> ()
              }
              frame "Laser on? Control" {
                n959 = flat-sequence {
                  tunnel: w1224 -> [w1232]
                  tunnel: w1223 -> [w1231]
                  tunnel: [w1230] -> w1220
                  tunnel: [w1229] -> w1219
                  tunnel: [w1240] -> w1221
                  tunnel: [w1241] -> w1222
                  tunnel: w1220 -> [w1241]
                  tunnel: w1219 -> [w1240]
                  tunnel: [w1239] -> w1218
                  tunnel: [w1238] -> w1217
                  tunnel: w1216 -> [w1237]
                  tunnel: w1215 -> [w1236]
                  frame #0 {
                    n960 = call <instrlib>:"TL4000 Get LD Output State.vi"("error in (no error)"=w1231, "instrument handle"=w1232) -> ("error out"=w1226:errorcluster, "LD Output"=w1228:bool, "instrument handle out"=w1227:refnum<visa-resource-name>)  [unwired: 7 in]
                    n961 = case shown="False" w1228 {
                      selector: w1228 -> [w1233 w1234]
                      frame False {
                        n962 = property on="TEC Output" class="Bool (strict)"("Visible"=w1233) -> ()  [unwired: 2 in, 2 out]
                      }
                      frame True {
                        n963 = property on="TEC Output" class="Bool (strict)"("Visible"=w1234) -> ()  [unwired: 2 in, 2 out]
                      }
                    }
                    n964 = Not(x=w1228) -> (.not. x?=w1225:bool)
                    n965 = property on="Laser Safety" class="Ring (strict)"("Visible"=w1225) -> ()  [unwired: 2 in, 2 out]
                    n966 = local write "Laser on?"(w1225) -> ()
                    n967 = call <instrlib>:"TL4000 Switch LD Output.vi"("error in (no error)"=w1226, "LD Output (Off)"=w1225, "instrument handle"=w1227) -> ("error out"=w1230:errorcluster, "instrument handle out"=w1229:refnum<visa-resource-name>)  [unwired: 7 in]
                    n968 = property on="Laser Diode Current Set" class="Slide (strict)"("Visible"=w1225) -> ()  [unwired: 2 in, 2 out]
                  }
                  frame #1 {
                    n969 = call <instrlib>:"TLPM Measure Power.vi"("error in (no error)"=w1236, "instrument handle"=w1237) -> ("error out"=w1238:errorcluster, "Power"=w1235:dbl, "instrument handle out"=w1239:refnum<visa-resource-name>)  [unwired: 7 in]
                    n970 = local write "Excitation Power (uW)"(w1235) -> ()
                  }
                }
              }
              frame "Laser Diode Current Set" {
                n971 = flat-sequence {
                  tunnel: w1251 -> [w1260]
                  tunnel: w1250 -> [w1259]
                  tunnel: [w1255] -> w1247
                  tunnel: [w1254] -> w1246
                  tunnel: [w1273] -> w1248
                  tunnel: [w1274] -> w1249
                  tunnel: w1247 -> [w1274]
                  tunnel: w1246 -> [w1273]
                  tunnel: w1245 -> [w1272]
                  tunnel: w1244 -> [w1271]
                  tunnel: [w1270] -> w1243
                  tunnel: [w1269] -> w1242
                  frame #0 {
                    n972 = local read "Laser Diode Current Set"() -> (w1252:dbl)
                    n973 = call <instrlib>:"TL4000 Get Laser Diode Current Setpoint.vi"("error in (no error)"=w1259, "instrument handle"=w1260) -> ("error out"=w1256:errorcluster, "Laser Diode Current Setpoint"=w1258:dbl, "instrument handle out"=w1257:refnum<visa-resource-name>)  [unwired: 7 in]
                    n974 = Not Equal?(x=w1252, y=w1258) -> (x != y?=w1253:bool)
                    n975 = case shown="True" w1253 {
                      tunnel: w1257 -> [w1262 w1267]
                      tunnel: w1256 -> [w1261 w1266]
                      tunnel: [w1262 w1265] -> w1255
                      tunnel: [w1261 w1264] -> w1254
                      tunnel: w1252 -> [_ w1263]
                      frame False {
                      }
                      frame True {
                        n976 = call <instrlib>:"TL4000 Set Laser Diode Current Setpoint.vi"("error in (no error)"=w1266, "Laser Diode Current Setpoint (0.0)"=w1263, "instrument handle"=w1267) -> ("error out"=w1264:errorcluster, "instrument handle out"=w1265:refnum<visa-resource-name>)  [unwired: 7 in]
                      }
                    }
                  }
                  frame #1 {
                    n977 = call <instrlib>:"TLPM Measure Power.vi"("error in (no error)"=w1271, "instrument handle"=w1272) -> ("error out"=w1269:errorcluster, "Power"=w1268:dbl, "instrument handle out"=w1270:refnum<visa-resource-name>)  [unwired: 7 in]
                    n978 = local write "Excitation Power (uW)"(w1268) -> ()
                  }
                }
              }
              frame "TEC Output", Default {
                n979 = call <instrlib>:"TL4000 Get TEC Output State.vi"("error in (no error)"=w1284, "instrument handle"=w1285) -> ("error out"=w1282:errorcluster, "TEC Output"=w1286:bool, "instrument handle out"=w1283:refnum<visa-resource-name>)  [unwired: 7 in]
                n980 = Not(x=w1286) -> (.not. x?=w1275:bool)
                n981 = call <instrlib>:"TL4000 Switch TEC Output.vi"("error in (no error)"=w1282, "TEC Output (Off)"=w1275, "instrument handle"=w1283) -> ("error out"=w1280:errorcluster, "instrument handle out"=w1281:refnum<visa-resource-name>)  [unwired: 7 in]
                n982 = property on="Laser on? Control" class="Bool (strict)"("Visible"=w1275) -> ()  [unwired: 2 in, 2 out]
                n983 = case shown="True" w1275 {
                  tunnel: w1281 -> [w1288 w1295]
                  tunnel: w1280 -> [w1287 w1294]
                  tunnel: [w1288 w1291] -> w1276
                  tunnel: [w1287 w1290] -> w1279
                  frame False {
                  }
                  frame True {
                    n984 = while {
                      tunnel: w1295 -> [w1309]
                      tunnel: w1294 -> [w1308]
                      tunnel: [w1302] -> w1293
                      tunnel: [w1301] -> w1292
                      stop <- w1296 stop-if-true
                      n985 = call <instrlib>:"TL4000 Measure Temperature.vi"("error in (no error)"=w1308, "instrument handle"=w1309) -> ("error out"=w1302:errorcluster, "Temperature"=w1299:dbl, "instrument handle out"=w1301:refnum<visa-resource-name>)  [unwired: 7 in]
                      n986 = Wait (ms)(milliseconds to wait=u32 50) -> ()  [unwired: 1 out]
                      n987 = local write "TEC Temperature"(w1299) -> ()
                      n988 = Subtract(x=w1299, y=25.0) -> (x-y=w1306:dbl)
                      n989 = Absolute Value(x=w1306) -> (abs(x)=w1305:dbl)
                      n990 = Less?(x=w1305, y=0.01) -> (x < y?=w1300:bool)
                      n991 = Equal?(x=w1299, y=0.0) -> (x = y?=w1297:bool)
                      n992 = Or(x=w1300, y=w1297) -> (x .or. y?=w1296:bool)
                    }
                    n993 = call <instrlib>:"TL4000 Measure Temperature.vi"("error in (no error)"=w1293, "instrument handle"=w1292) -> ("error out"=w1290:errorcluster, "Temperature"=w1289:dbl, "instrument handle out"=w1291:refnum<visa-resource-name>)  [unwired: 7 in]
                    n994 = local write "TEC Temperature"(w1289) -> ()
                  }
                }
                n995 = property on="TEC Temperature" class="DigNum (strict)"("Visible"=w1275) -> ()  [unwired: 2 in, 2 out]
                n996 = local write "TEC Output"(w1275) -> ()
              }
            }
            n997 = local write "Diode Driver COM"(w1205) -> ()
            n998 = local write "Diode Driver Error"(w1204) -> ()
            n999 = local write "Photodiode error out"(w1198) -> ()
            n1000 = local write "Photodiode COM Port"(w1199) -> ()
          }
          event "Center Wavelength (nm)": Value Change {
            n1001 = event-data() -> ("NewVal"=w1310:dbl)  [unwired: 1 in, 5 out]
            n1002 = local read "LightField Automation error out"() -> (w1317:errorcluster)
            n1003 = local read "LightField Automation out"() -> (w1318:refnum<class "LightField Automation.lvclass">)
            n1004 = call "spec_GetCenterWavelength.vi"("error in (no error)"=w1317, "LightField Automation in"=w1318) -> ("error out"=w1313:errorcluster, "Center Wavelength"=w1316:dbl, "LightField Automation out"=w1314:refnum<class "LightField Automation.lvclass">)  [unwired: 7 in]
            n1005 = Equal?(x=w1310, y=w1316) -> (x = y?=w1315:bool)
            n1006 = case shown="False" w1315 {
              tunnel: w1314 -> [w1323 w1343]
              tunnel: w1313 -> [w1322 w1342]
              tunnel: [w1319 w1343] -> w1312
              tunnel: [w1320 w1342] -> w1311
              tunnel: w1310 -> [w1321 _]
              frame False {
                n1007 = stacked-sequence {
                  seq-local: [w1327 _] -> [_ w1341]
                  seq-local: [w1326 _] -> [_ w1340]
                  seq-local: [w1324 _] -> [_ w1339]
                  tunnel: w1323 -> [w1331 _]
                  tunnel: w1322 -> [w1330 _]
                  tunnel: w1321 -> [w1324 _]
                  tunnel: [_ w1341] -> w1320
                  tunnel: [_ w1340] -> w1319
                  frame #0 {
                    n1008 = call "spec_SetCenterWavelength.vi"("error in (no error)"=w1330, "Center Wavelength"=w1324, "LightField Automation in"=w1331) -> ("error out"=w1328:errorcluster, "LightField Automation out"=w1329:refnum<class "LightField Automation.lvclass">)  [unwired: 7 in]
                    n1009 = call "spec_getCalibration.vi"("error in (no error)"=w1328, "LightField Automation in"=w1329) -> ("error out"=w1327:errorcluster, "ColumnCalibration"=w1325:dbl[], "LightField Automation out"=w1326:refnum<class "LightField Automation.lvclass">)  [unwired: 7 in]
                    n1010 = local write "Wavelength calibration"(w1325) -> ()
                  }
                  frame #1 {
                    n1011 = Format Into String(format string="%3.2f", initial string="Wavelength set to ", w1339) -> (resulting string=w1337:string)  [unwired: 1 in, 1 out]
                    n1012 = local read "Log file"() -> (w1334:string)
                    n1013 = Concatenate Strings(w1337, " nm") -> (w1335:string)
                    n1014 = call "Write2LogFile.vi"("Add to log file"=w1335, "Log file before"=w1334) -> ("Log file after"=w1333:string)
                    n1015 = local write "Log file"(w1333) -> ()
                  }
                }
              }
              frame True {
              }
            }
            n1016 = local write "LightField Automation out"(w1312) -> ()
            n1017 = local write "LightField Automation error out"(w1311) -> ()
          }
          event "CCD 1D Spectrum Main  Cursor2WL 1 Mono 1", "CCD 1D Spectrum Main  Cursor2WL 2 Mono 1": Mouse Down {
            n1018 = event-data() -> ("CtlRef"=w1345:refnum<vi>)  [unwired: 1 in, 7 out]
            n1019 = property class="Bool (strict)"(reference=w1345) -> ("Label.Text"=w1344:string)  [unwired: 1 in, 2 out]
            n1020 = case shown="\"CCD 1D Spectrum Main  Cursor2WL 2\"" w1344 {
              tunnel: [w1347 w1348] -> w1346
              frame "CCD 1D Spectrum Main  Cursor2WL 1", Default {
                n1021 = local read "CCD 1D Spectrum Main Cursor 1 nm"() -> (w1347:dbl)
              }
              frame "CCD 1D Spectrum Main  Cursor2WL 2" {
                n1022 = local read "CCD 1D Spectrum Main Cursor 2 nm"() -> (w1348:dbl)
              }
            }
            n1023 = property on="Center Wavelength (nm)" class="DigNum (strict)"("Val(Sgnl)"=w1346) -> ()  [unwired: 2 in, 2 out]
          }
          event "Cryostat": Value Change {
            n1024 = event-data() -> ("NewVal"=w1349:enum16{"Montana", "Oxford"})  [unwired: 1 in, 5 out]
            n1025 = case shown="\"Oxford\"" w1349 {
              frame "Oxford" {
                w1350 = FALSE
                n1026 = property on="FSM Up" class="Bool (strict)"("Visible"=w1350) -> ()  [unwired: 2 in, 2 out]
                n1027 = property on="FSM Left" class="Bool (strict)"("Visible"=w1350) -> ()  [unwired: 2 in, 2 out]
                n1028 = property on="FSM Axis Step" class="DigNum (strict)"("Visible"=w1350) -> ()  [unwired: 2 in, 2 out]
                n1029 = property on="FSM Down" class="Bool (strict)"("Visible"=w1350) -> ()  [unwired: 2 in, 2 out]
                n1030 = property on="FSM Right" class="Bool (strict)"("Visible"=w1350) -> ()  [unwired: 2 in, 2 out]
              }
              frame "Montana" {
                w1351 = TRUE
                n1031 = property on="FSM Up" class="Bool (strict)"("Visible"=w1351) -> ()  [unwired: 2 in, 2 out]
                n1032 = property on="FSM Left" class="Bool (strict)"("Visible"=w1351) -> ()  [unwired: 2 in, 2 out]
                n1033 = property on="FSM Axis Step" class="DigNum (strict)"("Visible"=w1351) -> ()  [unwired: 2 in, 2 out]
                n1034 = property on="FSM Down" class="Bool (strict)"("Visible"=w1351) -> ()  [unwired: 2 in, 2 out]
                n1035 = property on="FSM Right" class="Bool (strict)"("Visible"=w1351) -> ()  [unwired: 2 in, 2 out]
              }
            }
          }
          event "Shutter Mode": Value Change {
            # "1 Active == Laser on / Shutter off\n2 Inactive == Laser off / Shutter on\n\nThere are 4 operating modes for shutter:\n1 Manual\n2 Single Toggle\n3 Automatic Toggle\n4 Triggered"
            n1036 = event-data() -> ()  [unwired: 1 in, 6 out]
            n1037 = local read "KCube Shutter Device Reference"() -> (w1353:refnum<k24>)
            n1038 = local read "Shutter Mode"() -> (w1352:i32)
            n1039 = invoke class="KCubeSolenoid" method="SetOperatingMode"(reference=w1353, "mode"=w1352) -> ()  [unwired: 2 in, 4 out]
          }
          event "Save Spectrum", "Save Spectrum N", "Save XY Map", "Save Polarisation", "Save Contrast": Value Change {
            n1040 = event-data() -> ("CtlRef"=w1355:refnum<vi>)  [unwired: 1 in, 3 out]
            n1041 = property class="Bool (strict)"(reference=w1355) -> ("Label.Text"=w1354:string)  [unwired: 1 in, 2 out]
            n1042 = stacked-sequence {
              tunnel: w1354 -> [w1363 _]
              frame #0 {
                n1043 = local read "Excitation Power (uW)"() -> (w1362:dbl)
                n1044 = local read "Center Wavelength (nm)"() -> (w1368:dbl)
                n1045 = local read "Exposure Time (ms)"() -> (w1369:dbl)
                n1046 = local read "Experiment Name"() -> (w1367:string)
                n1047 = local read "Excitation Wavelength (nm)"() -> (w1358:dbl)
                n1048 = local read "Temperature (K)"() -> (w1371:dbl)
                n1049 = local read "Excitation Source"() -> (w1370:enum16{"P", "CW"})
                n1050 = local read "Wavelength calibration"() -> (w1356:dbl[])
                n1051 = local read "Acq Mode"() -> (w1359:T1)
                n1052 = local read "Exposure Time (ms)"() -> (w1357:dbl)
                n1053 = local read "Comment"() -> (w1366:string)
                n1054 = local read "Log file"() -> (w1365:string)
                n1055 = Multiply(x=w1362, y=1000000.0) -> (x*y=w1360:dbl)
                n1056 = case shown="\"Save Cont\"" w1363 {
                  tunnel: w1360 -> [_ _ w1379 w1395 w1408]
                  tunnel: w1371 -> [_ _ w1381 w1396 w1407]
                  tunnel: w1370 -> [_ _ w1378 w1394 w1406]
                  tunnel: w1369 -> [_ _ w1377 _ w1405]
                  tunnel: w1368 -> [_ _ w1380 _ w1404]
                  tunnel: w1367 -> [_ _ w1383 w1393 w1403]
                  tunnel: w1366 -> [_ _ w1382 w1397 w1402]
                  tunnel: w1365 -> [w1372 w1373 w1384 w1391 w1401]
                  tunnel: [w1372 w1373 w1385 w1390 w1400] -> w1364
                  tunnel: w1359 -> [_ _ w1375 w1392 _]
                  tunnel: w1358 -> [_ _ _ w1389 _]
                  tunnel: w1357 -> [_ _ _ w1388 _]
                  tunnel: w1356 -> [_ _ _ w1386 _]
                  frame "Save Spectrum N" {
                  }
                  frame "Save XY Map" {
                  }
                  frame "Save Cont" {
                    n1057 = local read "Contrast Array Out"() -> (w1374:dbl[][])
                    n1058 = call "Format&SaveDataWithAttributes.vi"("Comment"=w1382, "T_K"=w1381, "Det_Mono1_CenterWL_nm"=w1380, "EPow_uW"=w1379, "ESource"=w1378, "Time_ms"=w1377, "Measurement type"=T12."Contrast", "FileName"=w1383, "Acq Mode"=w1375, "Log File In"=w1384, "Data_CCD_px"=w1374) -> ("Log File Out"=w1385:string)  [unwired: 15 in, 1 out]
                  }
                  frame "Save Polarisation" {
                    n1059 = property on="Polarisation 2D Image" class="IntGraph (strict)"() -> ("Value"=w1398:dbl[][])  [unwired: 2 in, 2 out]
                    n1060 = call "Format&SaveDataWithAttributes.vi"("Comment"=w1397, "T_K"=w1396, "EPow_uW"=w1395, "ESource"=w1394, "EWL_nm"=w1389, "Time_ms"=w1388, "Measurement type"=T12."Polarisation", "FileName"=w1393, "WL_nm"=w1386, "Acq Mode"=w1392, "Log File In"=w1391, "Data_CCD_px"=w1398) -> ("Log File Out"=w1390:string)  [unwired: 14 in, 1 out]
                  }
                  frame "Save Spectrum", Default {
                    n1061 = local read "Acq Mode"() -> (w1399:T1)
                    n1062 = case shown="\"Spectrum\", Default" w1399 {
                      tunnel: w1408 -> [w1422 w1435]
                      tunnel: w1407 -> [w1421 w1434]
                      tunnel: w1406 -> [w1420 w1433]
                      tunnel: w1405 -> [w1419 w1432]
                      tunnel: w1404 -> [w1418 w1431]
                      tunnel: w1403 -> [w1417 w1430]
                      tunnel: w1402 -> [w1416 w1429]
                      tunnel: w1401 -> [w1415 w1428]
                      tunnel: [w1414 w1427] -> w1400
                      tunnel: w1399 -> [w1410 w1426]
                      frame "Spectrum", Default {
                        n1063 = local read "CCD 1D Spectrum Main"() -> (w1413:cluster{dbl[], dbl[]})
                        n1064 = Unbundle(w1413) -> (w1412:dbl[], w1411:dbl[])
                        n1065 = call "Format&SaveDataWithAttributes.vi"("Comment"=w1416, "T_K"=w1421, "Det_Mono1_CenterWL_nm"=w1418, "EPow_uW"=w1422, "ESource"=w1420, "Time_ms"=w1419, "Measurement type"=T12."Spectrum", "Data_PLInt_cts"=w1411, "FileName"=w1417, "WL_nm"=w1412, "Acq Mode"=w1410, "Log File In"=w1415) -> ("Log File Out"=w1414:string)  [unwired: 14 in, 1 out]
                      }
                      frame "Image" {
                        n1066 = local read "Wavelength calibration"() -> (w1425:dbl[])
                        n1067 = local read "CCD 2D Image Main"() -> (w1423:dbl[][])
                        n1068 = call "Format&SaveDataWithAttributes.vi"("Comment"=w1429, "T_K"=w1434, "Det_Mono1_CenterWL_nm"=w1431, "EPow_uW"=w1435, "ESource"=w1433, "Time_ms"=w1432, "Measurement type"=T12."Spectrum", "FileName"=w1430, "WL_nm"=w1425, "Acq Mode"=w1426, "Log File In"=w1428, "Data_CCD_px"=w1423) -> ("Log File Out"=w1427:string)  [unwired: 14 in, 1 out]
                      }
                    }
                  }
                }
                n1069 = local write "Log file"(w1364) -> ()
              }
              frame #1 {
                w1436 = FALSE
                n1070 = local write "Save XY Map"(w1436) -> ()
                n1071 = local write "Save Polarisation"(w1436) -> ()
                n1072 = local write "Save Spectrum N"(w1436) -> ()
                n1073 = local write "Save Spectrum"(w1436) -> ()
              }
            }
          }
          event "Auto< ?": Value Change {
            n1074 = event-data() -> ("NewVal"=w1437:bool)  [unwired: 1 in, 5 out]
            n1075 = case shown="True" w1437 {
              frame False {
                w1438 = TRUE ("Visible")
                n1076 = property on="Save Spectrum N" class="Bool (strict)"("Visible"=w1438) -> ()  [unwired: 2 in, 2 out]
                n1077 = property on="Save XY Map" class="Bool (strict)"("Visible"=w1438) -> ()  [unwired: 2 in, 2 out]
                n1078 = property on="Save Spectrum" class="Bool (strict)"("Visible"=w1438) -> ()  [unwired: 2 in, 2 out]
                n1079 = property on="Save Polarisation" class="Bool (strict)"("Visible"=w1438) -> ()  [unwired: 2 in, 2 out]
              }
              frame True {
                w1439 = FALSE ("Visible")
                n1080 = property on="Save Spectrum N" class="Bool (strict)"("Visible"=w1439) -> ()  [unwired: 2 in, 2 out]
                n1081 = property on="Save XY Map" class="Bool (strict)"("Visible"=w1439) -> ()  [unwired: 2 in, 2 out]
                n1082 = property on="Save Spectrum" class="Bool (strict)"("Visible"=w1439) -> ()  [unwired: 2 in, 2 out]
                n1083 = property on="Save Polarisation" class="Bool (strict)"("Visible"=w1439) -> ()  [unwired: 2 in, 2 out]
              }
            }
          }
        }
      }
    }
    frame #2 {
      # "Shutdown: close all open references and connections"
      n1084 = stacked-sequence {
        frame #0 {
          # "Shutdown all connections"
          n1085 = local read "Initialise all devices?"() -> (w1440:bool)
          n1086 = case shown="True" w1440 {
            frame False {
              # "No devices to deactivate"
            }
            frame True {
              # "Deactivate all the selected devices"
              n1087 = stacked-sequence {
                frame #0 {
                  # "Message to user"
                  n1088 = local read "Log file"() -> (w1443:string)
                  n1089 = call "Write2LogFile.vi"("Add to log file"="Closing all connections ...", "Log file before"=w1443) -> ("Log file after"=w1442:string)
                  n1090 = local write "Log file"(w1442) -> ()
                }
                frame #1 {
                  # "KCubes: 1 Shutter + 3 Piezos"
                  n1091 = local read "KCubes Piezo On?"() -> (w1445:bool)
                  n1092 = case shown="True" w1445 {
                    frame False {
                    }
                    frame True {
                      # "Close piezo controls and shutter device"
                      n1093 = local read "KCubePiezoControl Y Reference"() -> (w1448:refnum<k24>)
                      n1094 = local read "KCubePiezoControl X Reference"() -> (w1447:refnum<k24>)
                      n1095 = local read "KCubePiezoControl Z Reference"() -> (w1449:refnum<k24>)
                      n1096 = invoke class="KCubePiezoControl" method="CloseDevice"(reference=w1448) -> ()  [unwired: 2 in, 3 out]
                      n1097 = invoke class="KCubePiezoControl" method="CloseDevice"(reference=w1447) -> ()  [unwired: 2 in, 3 out]
                      n1098 = invoke class="KCubePiezoControl" method="CloseDevice"(reference=w1449) -> ()  [unwired: 2 in, 3 out]
                    }
                  }
                  n1099 = local read "KCube Shutter On?"() -> (w1444:bool)
                  n1100 = case shown="True" w1444 {
                    frame False {
                    }
                    frame True {
                      n1101 = local read "KCubeSolenoidControl Reference"() -> (w1446:refnum<k24>)
                      n1102 = invoke class="KCubeSolenoidControl" method="CloseDevice"(reference=w1446) -> ()  [unwired: 2 in, 3 out]
                    }
                  }
                }
                frame #2 {
                  # "LightField: SpectraPro Mono + CCD"
                  n1103 = local read "LightField On?"() -> (w1450:bool)
                  n1104 = case shown="True" w1450 {
                    frame False {
                    }
                    frame True {
                      n1105 = local read "LightField Automation error out"() -> (w1451:errorcluster)
                      n1106 = local read "LightField Automation out"() -> (w1452:refnum<class "LightField Automation.lvclass">)
                      n1107 = call "LFA_Close.vi"("error in (no error)"=w1451, "LightField Automation in"=w1452) -> ()  [unwired: 8 in, 2 out]
                    }
                  }
                }
                frame #3 {
                  # "ESP 301: 2 rotation stages + 1 linear translation stage"
                  n1108 = local read "ESP 301 On?"() -> (w1453:bool)
                  n1109 = case shown="True" w1453 {
                    frame False {
                    }
                    frame True {
                      n1110 = local read "ESP 301 COM Port"() -> (w1455:refnum<visa-resource-name>)
                      n1111 = local read "ESP 301 Error"() -> (w1454:errorcluster)
                      n1112 = call "Close.vi"("error in (no error)"=w1454, "VISA resource name"=w1455) -> ()  [unwired: 9 in, 1 out]
                    }
                  }
                }
                frame #4 {
                  # "ESP 300: Mono Jobin Yvon"
                  n1113 = local read "ESP 300 On?"() -> (w1456:bool)
                  n1114 = case shown="True" w1456 {
                    frame False {
                    }
                    frame True {
                      n1115 = local read "ESP 300 COM Port"() -> (w1457:refnum<visa-resource-name>)
                      n1116 = local read "ESP300 Error"() -> (w1458:errorcluster)
                      n1117 = call "Uninit Communication.vi"("error in (no error)"=w1458, "VISA resource name in"=w1457) -> ()  [unwired: 9 in, 1 out]
                    }
                  }
                }
                frame #5 {
                  # "turn off laser output, TEC and close connection"
                  # "448.3nm Laser Diode + Temp Controller & Driver"
                  n1118 = local read "Laser Comm On?"() -> (w1459:bool)
                  n1119 = case shown="True" w1459 {
                    frame False {
                    }
                    frame True {
                      w1460 = FALSE ("LD Output (Off)")
                      n1120 = local read "Diode Driver COM"() -> (w1467:refnum<visa-resource-name>)
                      n1121 = local read "Diode Driver Error"() -> (w1466:errorcluster)
                      n1122 = property on="TEC Temperature" class="DigNum (strict)"("Visible"=w1460) -> ()  [unwired: 2 in, 2 out]
                      n1123 = property on="Laser on? Control" class="Bool (strict)"("Visible"=w1460) -> ()  [unwired: 2 in, 2 out]
                      n1124 = Not(x=w1460) -> (.not. x?=w1461:bool)
                      n1125 = call <instrlib>:"TL4000 Switch LD Output.vi"("error in (no error)"=w1466, "LD Output (Off)"=w1460, "instrument handle"=w1467) -> ("error out"=w1465:errorcluster, "instrument handle out"=w1464:refnum<visa-resource-name>)  [unwired: 7 in]
                      n1126 = property on="Laser Safety" class="Ring (strict)"("Visible"=w1460) -> ()  [unwired: 2 in, 2 out]
                      n1127 = local write "Laser on? Control"(w1460) -> ()
                      n1128 = local write "Laser on?"(w1460) -> ()
                      n1129 = property on="TEC Output" class="Bool (strict)"("Visible"=w1461) -> ()  [unwired: 2 in, 2 out]
                      n1130 = call <instrlib>:"TL4000 Switch TEC Output.vi"("error in (no error)"=w1465, "TEC Output (Off)"=w1460, "instrument handle"=w1464) -> ("error out"=w1462:errorcluster, "instrument handle out"=w1463:refnum<visa-resource-name>)  [unwired: 7 in]
                      n1131 = call <instrlib>:"TL4000 Close.vi"("error in (no error)"=w1462, "instrument handle"=w1463) -> ("error out"=w1468:errorcluster)  [unwired: 9 in]
                      n1132 = local write "Diode Driver Error"(w1468) -> ()
                      n1133 = property on="Laser Diode Current Set" class="Slide (strict)"("Visible"=w1460) -> ()  [unwired: 2 in, 2 out]
                      n1134 = local write "TEC Output"(w1460) -> ()
                    }
                  }
                }
                frame #6 {
                  # "Thorlabs USB photodiode"
                  n1135 = local read "PM16-120 On?"() -> (w1469:bool)
                  n1136 = case shown="True" w1469 {
                    frame False {
                    }
                    frame True {
                      n1137 = local read "Photodiode handle out"() -> (w1474:refnum<visa-resource-name>)
                      n1138 = local read "Photodiode error out"() -> (w1473:errorcluster)
                      n1139 = call <instrlib>:"TLPM Measure Power.vi"("error in (no error)"=w1473, "instrument handle"=w1474) -> ("error out"=w1471:errorcluster, "Power"=w1470:dbl, "instrument handle out"=w1472:refnum<visa-resource-name>)  [unwired: 7 in]
                      n1140 = call <instrlib>:"TLPM Close.vi"("error in (no error)"=w1471, "instrument handle"=w1472) -> ("error out"=w1475:errorcluster)  [unwired: 9 in]
                      n1141 = local write "Excitation Power (uW)"(w1470) -> ()
                      n1142 = local write "Photodiode error out"(w1475) -> ()
                    }
                  }
                }
              }
            }
          }
        }
        frame #1 {
          # "Save log file & empty strings for next operation"
          n1143 = property on="Experiment Graph Controls" class="TabCtl (strict)"() -> ("Pages"=w1479:refnum<vi>[])  [unwired: 2 in, 2 out]
          n1144 = stacked-sequence {
            frame #0 {
              # "save log file"
              n1145 = local read "Experiment Name"() -> (w1483:string)
              n1146 = local read "Log file"() -> (w1484:string)
              n1147 = call "CreatePath.vi"("filetype"=enum16{".h5", ".txt"}.".txt", "FileName"=w1483) -> ("File path"=w1481:path)
              n1148 = Write to Text File(file (use dialog)=w1481, text=w1484) -> ()  [unwired: 2 in, 3 out]
            }
            frame #1 {
              w1485 = ""
              # "reset log file and \ncomment to empty"
              n1149 = local write "Log file"(w1485) -> ()
              n1150 = local write "Comment"(w1485) -> ()
            }
          }
          n1151 = property on="Experiment Graph Controls" class="TabCtl (strict)"("Value"=T2."Settings" ("Experiment Graph Controls")) -> ()  [unwired: 2 in, 2 out]
          n1152 = Index Array(array=w1479, index=6) -> (element=w1477:refnum<vi>)
          n1153 = property class="Page"(reference=w1477, "PageVis"=TRUE ("Page Visible")) -> ()  [unwired: 1 in, 2 out]
        }
      }
    }
  }
  n1154 = disable-structure shown="Enabled" {
    frame Disabled {
    }
    frame Enabled {
      # "Progress bars"
      # "XYZ objective piezos and shutter"
      # "connected through"
      # "XY Scanning measurements"
      # "Polarisation measurement"
      # "Spectrum with CCD"
      # "Spectrum with APDs"
      # "Acquire controls"
      # "Save controls"
      # "CCD"
      # "MonochromatorS"
      # "Rotation stages PR50PP"
      # "Main"
      # "Photodiode PM16-120"
      # "Steering mirror FSM 300"
      # "Settings for instrumentation"
      # "Contrôle manip GH013"
      n1155 = property on="CCD 1D Spectrum Main Energy Scale" class="XYGraph (strict)"("Plot.Visible?"=FALSE ("Plot.Visible"), "Plot.Line Width"=u8 0) -> ()  [unwired: 2 in, 2 out]
      n1156 = local write "Photodiode Status"(FALSE) -> ()
      n1157 = property on="Polarisation 1D Spectrum Energy Scale" class="XYGraph (strict)"("Plot.Visible?"=FALSE ("Plot.Visible"), "Plot.Line Width"=u8 0) -> ()  [unwired: 2 in, 2 out]
      n1158 = control-ref of="Scan Fast Axis"() -> (w1504:refnum<vi>)
      n1159 = control-ref of="Scan X Num. Pts"() -> (w1500:refnum<vi>)
      n1160 = control-ref of="Scanning Mode"() -> (w1503:refnum<vi>)
      n1161 = control-ref of="Scan Y Center (V)"() -> (w1499:refnum<vi>)
      n1162 = control-ref of="Scan X Center (V)"() -> (w1502:refnum<vi>)
      n1163 = control-ref of="Scan Y Res. (V)"() -> (w1498:refnum<vi>)
      n1164 = control-ref of="Scan Y Num. Pts"() -> (w1497:refnum<vi>)
      n1165 = control-ref of="Polar Start Angle (°)"() -> (w1495:refnum<vi>)
      n1166 = control-ref of="Polar Step Angle (°)"() -> (w1493:refnum<vi>)
      n1167 = control-ref of="Polar End Angle (°)"() -> (w1494:refnum<vi>)
      n1168 = control-ref of="Scan X Res. (V)"() -> (w1501:refnum<vi>)
      n1169 = control-ref of="Polar mode"() -> (w1492:refnum<vi>)
      n1170 = Build Array(w1504, w1503, w1502, w1501, w1500, w1499, w1498, w1497) -> (→"Scan XY Map Params":refnum<vi>[])
      n1171 = Build Array(w1492, w1495, w1494, w1493) -> (→"Scan Polar Params":refnum<vi>[])
      n1172 = control-ref of="LinTFine Start Pos (usteps)"() -> (w1490:refnum<vi>)
      n1173 = control-ref of="LinTFines Step Pos (usteps)"() -> (w1489:refnum<vi>)
      n1174 = control-ref of="LinTFine End Pos (usteps)"() -> (w1488:refnum<vi>)
      n1175 = control-ref of="Acquire Contrast"() -> (w1487:refnum<vi>)
      n1176 = Build Array(w1490, w1489, w1488, w1487) -> (→"Scan LinTFine Params":refnum<vi>[])
    }
  }
